vi "RDG822 User.vi"() -> ()   [LabVIEW 2013]
panel:
  in  "MenuCount":u32=1
  in  "RemoveReq?":bool=TRUE
  in  "userID":string="0001"
  out "error out":errorcluster
  in  "E:\\Study\\НИР_Маг\\FP":path=path "E:/Study/НИР_Маг/FP"
  in  "error in":errorcluster
  in  "DC":bool
  in  "FallEdgeDBL":dbl=10.0 format="%.3f"
  in  "RisEdgeDBL":dbl=10.0 format="%.3f"
  out "FallEdgeStr":string="10.0 ns"
  out "RisEdgeStr":string="10.0 ns"
  in  "Duty/Width":bool
  in  "Width":dbl=500.0 format="%.4f"
  in  "SymmDBL":dbl=50.0 format="%.1f"
  out "SymmStr":string="50.0 %"
  in  "Duty":dbl=50.0 format="%.3f"
  out "Duty-Width":string="50.000 %"
  in  "Noise":bool
  in  "Pulse":bool
  in  "Ramp":bool
  in  "Square":bool
  in  "Sine":bool
  in  "Slider":bool
  in  "PhaseDBL":dbl format="%.3f"
  in  "OK":bool
  out "PhaseStr":string="0.000 °"
  in  "LowL":dbl=-2.5 format="%.4f"
  in  "Offset":dbl format="%.4f"
  out "Offset-LowL":string="0.0000 Vdc"
  in  "Offset/LowL":bool
  in  "HighL":dbl=1.0 format="%.4f"
  in  "Ampl":dbl=5.0 format="%.4f"
  out "Ampl-HighL":string="5.0000 Vpp"
  in  "Ampl/HighL":bool
  in  "Freq":dbl=1000.0 format="%.6f"
  in  "Period":dbl=1.0 format="%.7f"
  out "Freq-Period":string="1000.000000000 kHz"
  in  "Freq/Period":bool
  in  "Left":bool
  in  "Right":bool
  in  "Out2":bool
  in  "Out1":bool
  out "Screen":picture
  in  "Menu":bool
  in  "Home":bool
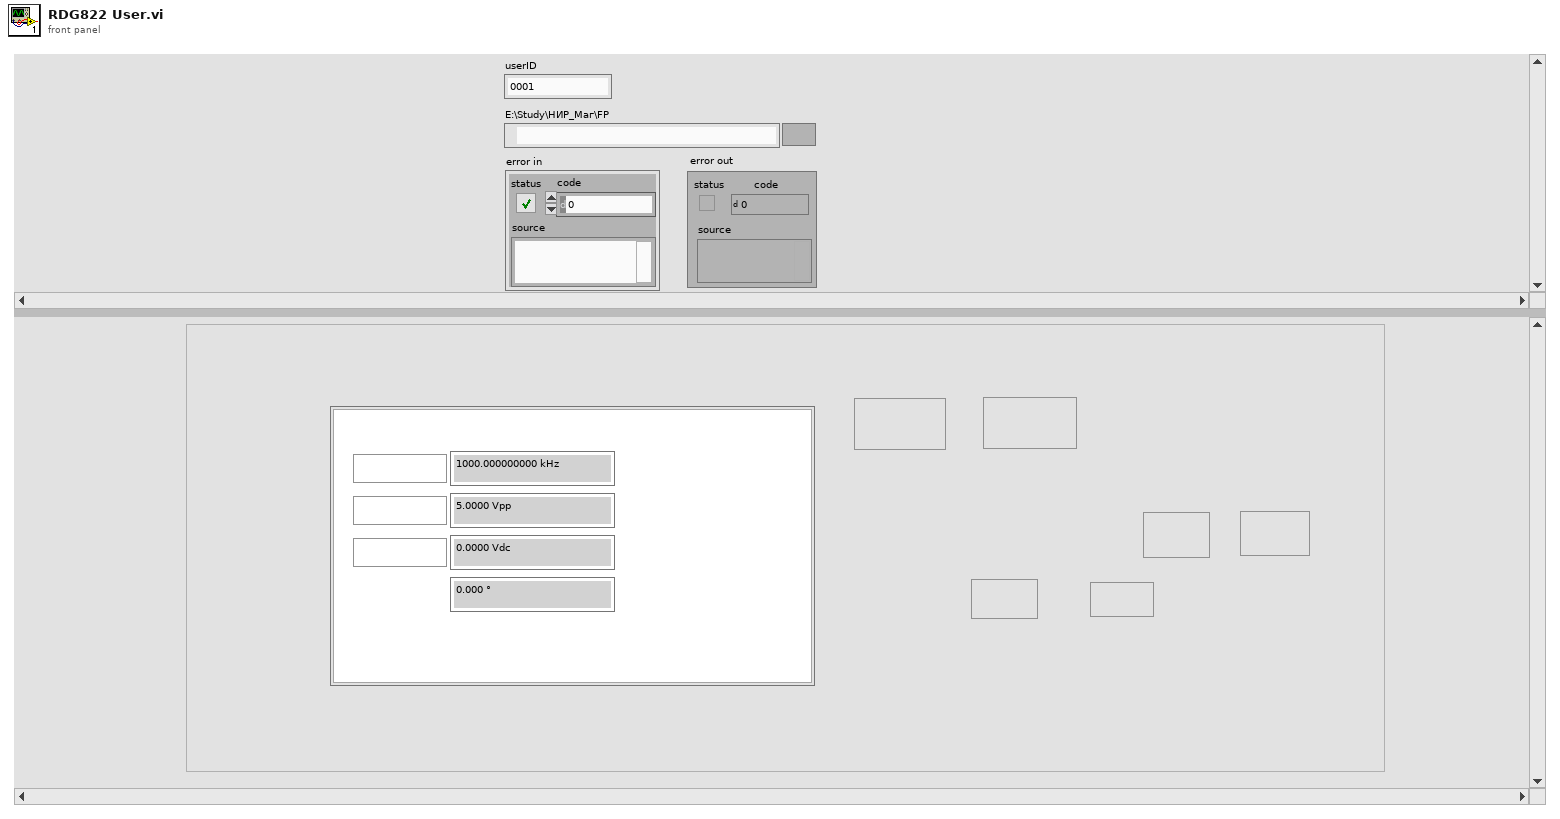
[diagram p1: front panel]
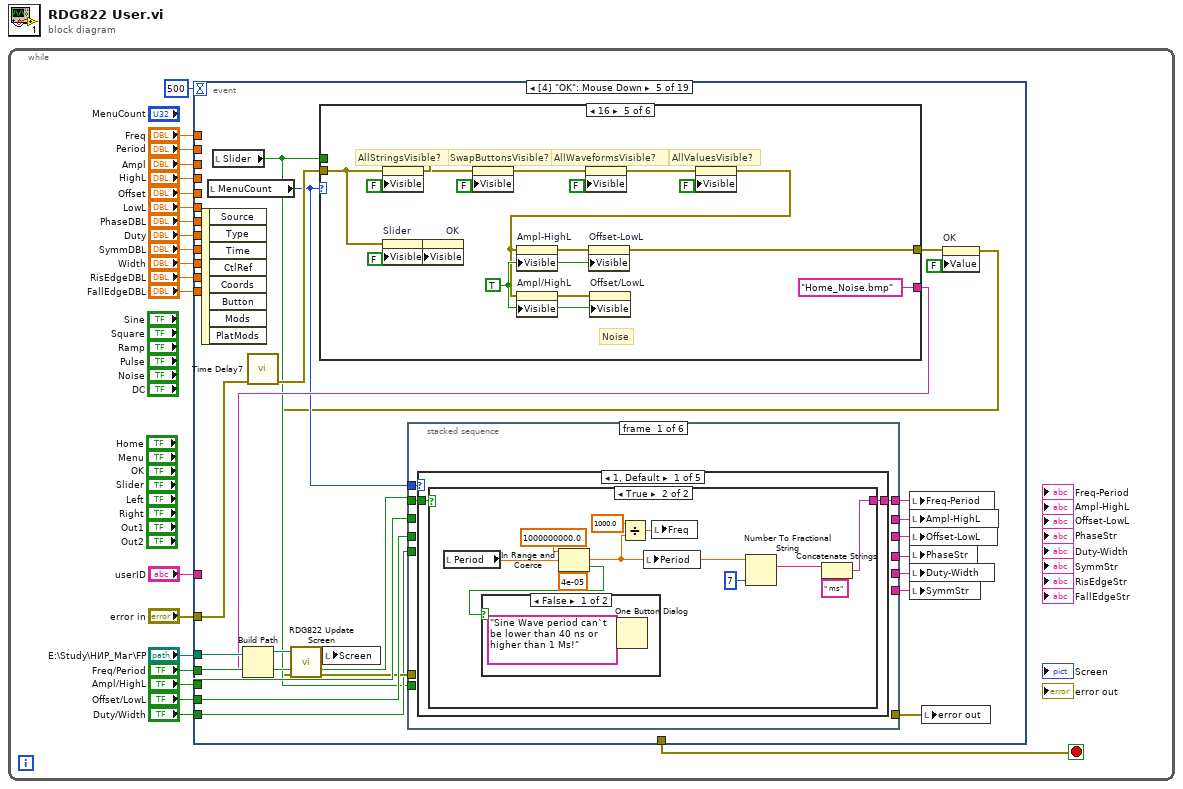
[diagram p0: block diagram]
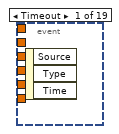
[diagram p2: hidden frame]
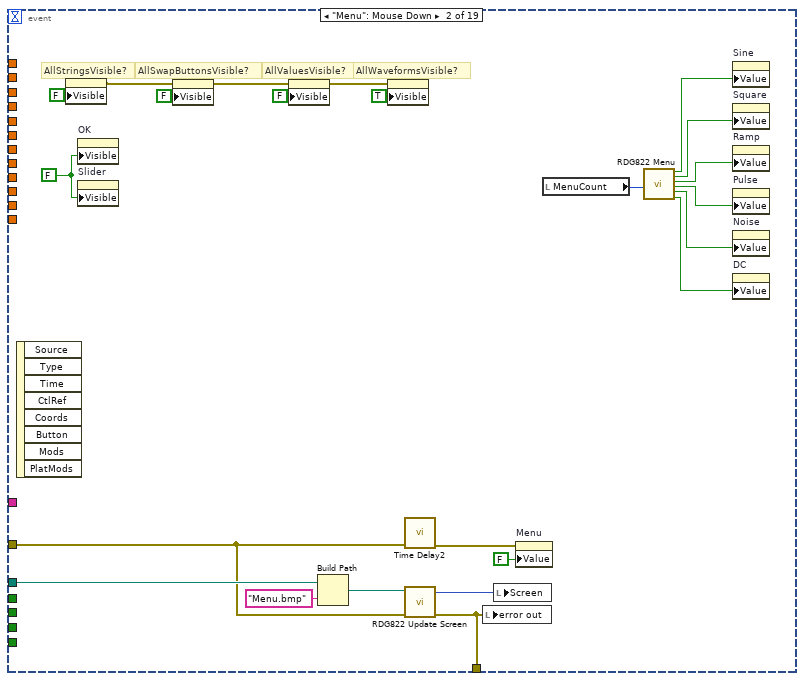
[diagram p3: hidden frame]
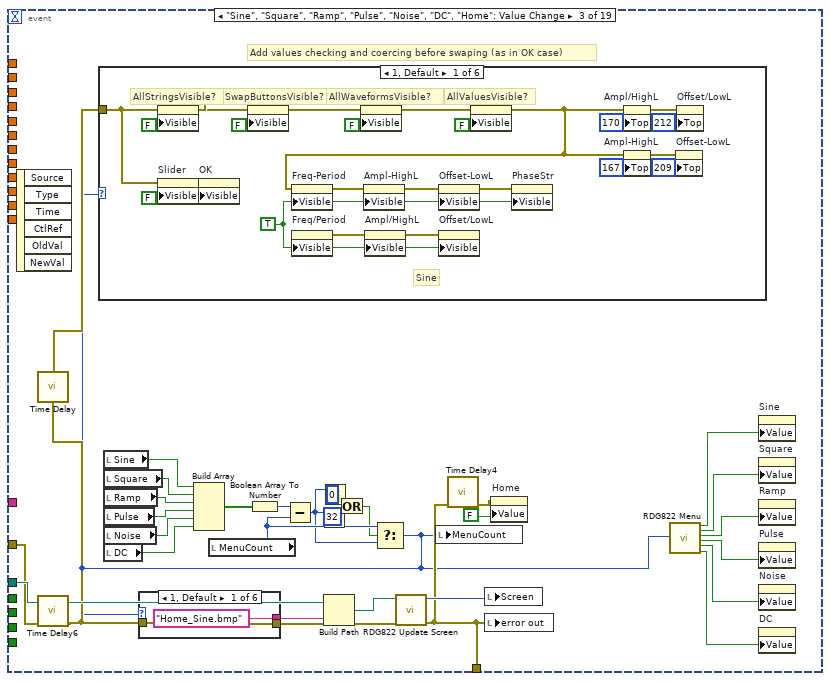
[diagram p4: hidden frame]
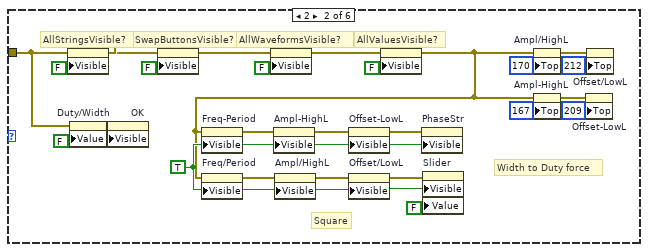
[diagram p5: hidden frame]
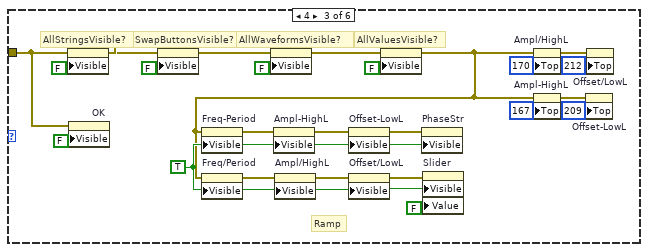
[diagram p6: hidden frame]
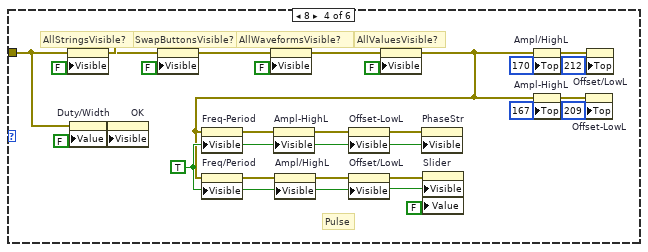
[diagram p7: hidden frame]
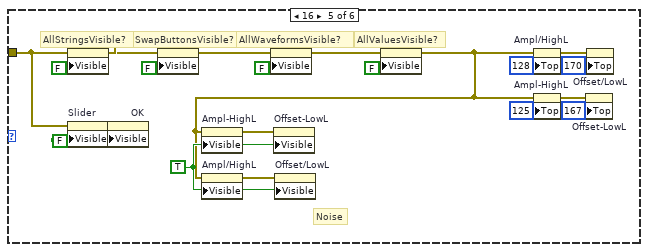
[diagram p8: hidden frame]
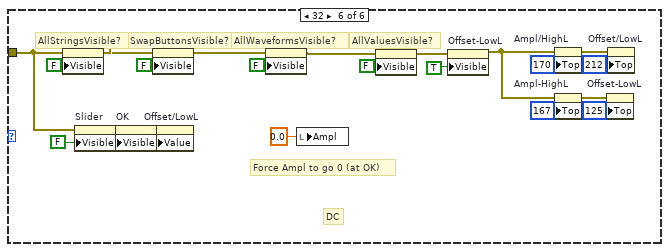
[diagram p9: hidden frame]
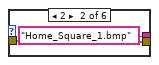
[diagram p10: hidden frame]
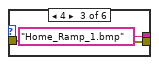
[diagram p11: hidden frame]
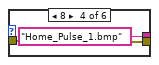
[diagram p12: hidden frame]
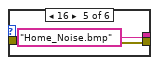
[diagram p13: hidden frame]
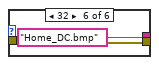
[diagram p14: hidden frame]
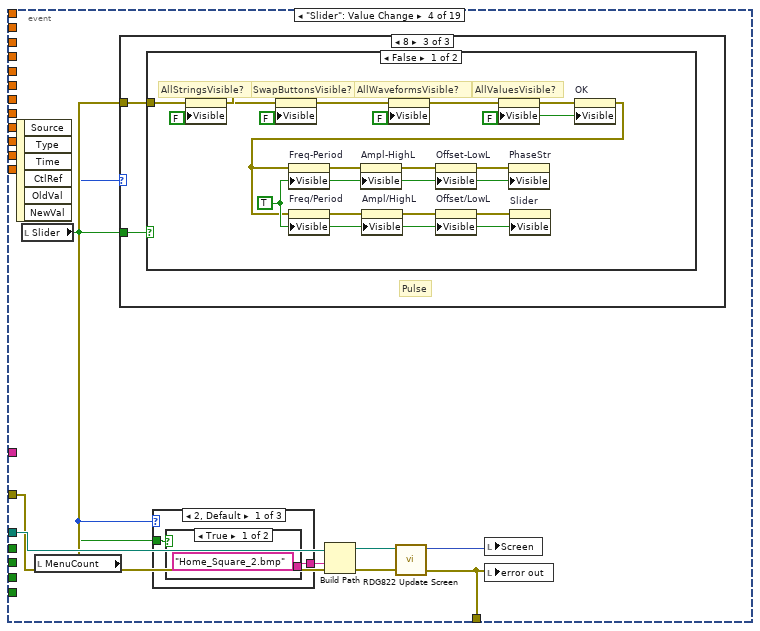
[diagram p15: hidden frame]
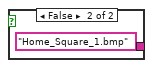
[diagram p16: hidden frame]
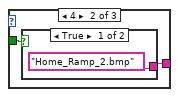
[diagram p17: hidden frame]
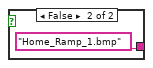
[diagram p18: hidden frame]
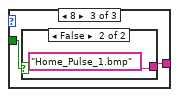
[diagram p19: hidden frame]
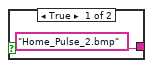
[diagram p20: hidden frame]
diagram:
  n1 = while {
    stop <- w21 stop-if-true
    n2 = event shown="[4] \"OK\": Mouse Down" {
      selector: _ -> [_ _ _ _ _ _ _ _ _ _ _ _ _ _ _ _ _ _ _]
      dyn-events: _ -> [_ _ _ _ _ _ _ _ _ _ _ _ _ _ _ _ _ _ _]
      timeout: 500 -> [_ _ _ _ _ _ _ _ _ _ _ _ _ _ _ _ _ _ _]
      tunnel: [_ w65 w89 w409 _ w1410 w1457 w1504 w1551 w1591 w1635 w1670 w1704 _ _ _ _ w1825 _] -> w21
      tunnel: "error in" -> [_ w63 w85 w408 w684 _ _ _ _ _ _ _ _ _ _ _ _ w1892 _]
      tunnel: "E:\\Study\\НИР_Маг\\FP" -> [_ w66 w93 w410 w693 w1415 w1462 w1509 w1556 w1587 w1639 w1675 w1709 _ _ _ _ w1880 _]
      tunnel: "Freq/Period" -> [_ _ _ _ w696 w1414 _ _ _ _ _ _ _ _ _ _ _ w1902 _]
      tunnel: "Ampl/HighL" -> [_ _ _ _ w695 _ w1461 _ _ _ _ _ _ _ _ _ _ w1903 _]
      tunnel: "Freq" -> [_ _ _ _ _ _ _ _ _ _ _ _ _ _ _ _ _ w1901 _]
      tunnel: "Ampl" -> [_ _ _ _ _ _ _ _ _ _ _ _ _ _ _ _ _ w1900 _]
      tunnel: "Period" -> [_ _ _ _ _ _ _ _ _ _ _ _ _ _ _ _ _ w1862 _]
      tunnel: "HighL" -> [_ _ _ _ _ _ _ _ _ _ _ _ _ _ _ _ _ w1897 _]
      tunnel: "Offset/LowL" -> [_ _ _ _ w694 _ _ w1508 _ _ _ _ _ _ _ _ _ w1899 _]
      tunnel: "Offset" -> [_ _ _ _ _ _ _ _ _ _ _ _ _ _ _ _ _ w1873 _]
      tunnel: "LowL" -> [_ _ _ _ _ _ _ _ _ _ _ _ _ _ _ _ _ w1898 _]
      tunnel: "PhaseDBL" -> [_ _ _ _ _ _ _ _ _ _ _ _ _ _ _ _ _ w1860 _]
      tunnel: "userID" -> [_ _ _ _ _ _ _ _ _ _ _ _ _ _ _ _ _ w1891 _]
      tunnel: "Duty" -> [_ _ _ _ _ _ _ _ _ _ _ _ _ _ _ _ _ w1865 _]
      tunnel: "SymmDBL" -> [_ _ _ _ _ _ _ _ _ _ _ _ _ _ _ _ _ w1868 _]
      tunnel: "Width" -> [_ _ _ _ _ _ _ _ _ _ _ _ _ _ _ _ _ w1863 _]
      tunnel: "Duty/Width" -> [_ _ _ _ w678 _ _ _ _ w1586 _ _ _ _ _ _ _ w1866 _]
      tunnel: "RisEdgeDBL" -> [_ _ _ _ _ _ _ _ _ _ _ _ _ _ _ _ _ _ _]
      tunnel: "FallEdgeDBL" -> [_ _ _ _ _ _ _ _ _ _ _ _ _ _ _ _ _ _ _]
      event Timeout {
        n3 = event-data() -> ()  [unwired: 1 in, 3 out]
      }
      event "Menu": Mouse Down {
        w34 = TRUE ("Visible")
        w47 = FALSE ("Visible")
        w54 = FALSE ("Visible")
        w57 = FALSE ("Visible")
        w61 = FALSE ("Visible")
        # "AllWaveformsVisible?"
        # "AllValuesVisible?"
        # "AllStringsVisible?"
        # "AllSwapButtonsVisible?"
        n4 = event-data() -> ()  [unwired: 1 in, 8 out]
        n5 = property on="Freq-Period" class="Str"("Visible"=w54) -> (error out=w52:errorcluster)  [unwired: 2 in, 1 out]
        n6 = property on="Ampl-HighL" class="Str"(error in=w52, "Visible"=w54) -> (error out=w51:errorcluster)  [unwired: 1 in, 1 out]
        n7 = property on="Offset-LowL" class="Str"(error in=w51, "Visible"=w54) -> (error out=w50:errorcluster)  [unwired: 1 in, 1 out]
        n8 = property on="PhaseStr" class="Str"(error in=w50, "Visible"=w54) -> (error out=w53:errorcluster)  [unwired: 1 in, 1 out]
        n9 = property on="Duty-Width" class="Str"(error in=w53, "Visible"=w54) -> (error out=w56:errorcluster)  [unwired: 1 in, 1 out]
        n10 = property on="SymmStr" class="Str"(error in=w56, "Visible"=w54) -> (error out=w55:errorcluster)  [unwired: 1 in, 1 out]
        n11 = property on="RisEdgeStr" class="Str"(error in=w55, "Visible"=w54) -> (error out=w49:errorcluster)  [unwired: 1 in, 1 out]
        n12 = property on="FallEdgeStr" class="Str"(error in=w49, "Visible"=w54) -> (error out=w48:errorcluster)  [unwired: 1 in, 1 out]
        n13 = property on="OK" class="Bool (strict)"("Visible"=w61) -> ()  [unwired: 2 in, 2 out]
        n14 = property on="Slider" class="Bool (strict)"("Visible"=w61) -> ()  [unwired: 2 in, 2 out]
        n15 = property on="Freq/Period" class="Bool (strict)"(error in=w48, "Visible"=w57) -> (error out=w60:errorcluster)  [unwired: 1 in, 1 out]
        n16 = property on="Ampl/HighL" class="Bool (strict)"(error in=w60, "Visible"=w57) -> (error out=w59:errorcluster)  [unwired: 1 in, 1 out]
        n17 = property on="Offset/LowL" class="Bool (strict)"(error in=w59, "Visible"=w57) -> (error out=w58:errorcluster)  [unwired: 1 in, 1 out]
        n18 = property on="Duty/Width" class="Bool (strict)"(error in=w58, "Visible"=w57) -> (error out=w35:errorcluster)  [unwired: 1 in, 1 out]
        n19 = property on="Freq" class="DigNum (strict)"(error in=w35, "Visible"=w47) -> (error out=w43:errorcluster)  [unwired: 1 in, 1 out]
        n20 = property on="Period" class="DigNum (strict)"(error in=w43, "Visible"=w47) -> (error out=w42:errorcluster)  [unwired: 1 in, 1 out]
        n21 = property on="Ampl" class="DigNum (strict)"(error in=w42, "Visible"=w47) -> (error out=w41:errorcluster)  [unwired: 1 in, 1 out]
        n22 = property on="HighL" class="DigNum (strict)"(error in=w41, "Visible"=w47) -> (error out=w44:errorcluster)  [unwired: 1 in, 1 out]
        n23 = property on="Offset" class="DigNum (strict)"(error in=w44, "Visible"=w47) -> (error out=w40:errorcluster)  [unwired: 1 in, 1 out]
        n24 = property on="LowL" class="DigNum (strict)"(error in=w40, "Visible"=w47) -> (error out=w39:errorcluster)  [unwired: 1 in, 1 out]
        n25 = property on="PhaseDBL" class="DigNum (strict)"(error in=w39, "Visible"=w47) -> (error out=w45:errorcluster)  [unwired: 1 in, 1 out]
        n26 = property on="Duty" class="DigNum (strict)"(error in=w45, "Visible"=w47) -> (error out=w46:errorcluster)  [unwired: 1 in, 1 out]
        n27 = property on="SymmDBL" class="DigNum (strict)"(error in=w46, "Visible"=w47) -> (error out=w38:errorcluster)  [unwired: 1 in, 1 out]
        n28 = property on="Width" class="DigNum (strict)"(error in=w38, "Visible"=w47) -> (error out=w37:errorcluster)  [unwired: 1 in, 1 out]
        n29 = property on="RisEdgeDBL" class="DigNum (strict)"(error in=w37, "Visible"=w47) -> (error out=w36:errorcluster)  [unwired: 1 in, 1 out]
        n30 = property on="FallEdgeDBL" class="DigNum (strict)"(error in=w36, "Visible"=w47) -> (error out=w28:errorcluster)  [unwired: 1 in, 1 out]
        n31 = Build Path(base path=w66, name or relative path="Menu.bmp") -> (appended path=w67:path)
        n32 = property on="Sine" class="Bool (strict)"(error in=w28, "Visible"=w34) -> (error out=w31:errorcluster)  [unwired: 1 in, 1 out]
        n33 = property on="Square" class="Bool (strict)"(error in=w31, "Visible"=w34) -> (error out=w30:errorcluster)  [unwired: 1 in, 1 out]
        n34 = property on="Ramp" class="Bool (strict)"(error in=w30, "Visible"=w34) -> (error out=w29:errorcluster)  [unwired: 1 in, 1 out]
        n35 = property on="Pulse" class="Bool (strict)"(error in=w29, "Visible"=w34) -> (error out=w32:errorcluster)  [unwired: 1 in, 1 out]
        n36 = property on="Noise" class="Bool (strict)"(error in=w32, "Visible"=w34) -> (error out=w33:errorcluster)  [unwired: 1 in, 1 out]
        n37 = property on="DC" class="Bool (strict)"(error in=w33, "Visible"=w34) -> ()  [unwired: 1 in, 2 out]
        n38 = call "Time Delay2"("error in (no error)"=w63) -> ("error out"=w70:errorcluster)  [unwired: 10 in]
        n39 = call "RDG822 Update Screen.vi"("error in"=w63, "Path to file"=w67) -> ("error out"=w65:errorcluster, "Screen"=w64:picture)  [unwired: 8 in]
        n40 = local write "error out"(w65) -> ()
        n41 = local write "Screen"(w64) -> ()
        n42 = property on="Menu" class="Bool (strict)"(error in=w70, "Value"=FALSE ("Visible")) -> ()  [unwired: 1 in, 2 out]
        n43 = local read "MenuCount"() -> (w62:u32)
        n44 = call "RDG822 Menu.vi"("MenuID"=w62) -> ("Sine"=w27:bool, "Square"=w26:bool, "Ramp"=w25:bool, "Pulse"=w24:bool, "Noise"=w23:bool, "DC"=w22:bool)  [unwired: 13 in]
        n45 = property on="Sine" class="Bool (strict)"("Value"=w27) -> ()  [unwired: 2 in, 2 out]
        n46 = property on="Square" class="Bool (strict)"("Value"=w26) -> ()  [unwired: 2 in, 2 out]
        n47 = property on="Ramp" class="Bool (strict)"("Value"=w25) -> ()  [unwired: 2 in, 2 out]
        n48 = property on="Pulse" class="Bool (strict)"("Value"=w24) -> ()  [unwired: 2 in, 2 out]
        n49 = property on="Noise" class="Bool (strict)"("Value"=w23) -> ()  [unwired: 2 in, 2 out]
        n50 = property on="DC" class="Bool (strict)"("Value"=w22) -> ()  [unwired: 2 in, 2 out]
      }
      event "Sine", "Square", "Ramp", "Pulse", "Noise", "DC", "Home": Value Change {
        # "Add values checking and coercing before swaping (as in OK case)"
        n51 = event-data() -> ()  [unwired: 1 in, 6 out]
        n52 = call "Time Delay6"("error in (no error)"=w85) -> ("error out"=w82:errorcluster)  [unwired: 10 in]
        n53 = call "Time Delay"("error in (no error)"=w82) -> ("error out"=w83:errorcluster)  [unwired: 10 in]
        n54 = local read "Sine"() -> (w98:bool)
        n55 = local read "Square"() -> (w99:bool)
        n56 = local read "Ramp"() -> (w100:bool)
        n57 = local read "Pulse"() -> (w97:bool)
        n58 = local read "Noise"() -> (w96:bool)
        n59 = local read "DC"() -> (w78:bool)
        n60 = Build Array(w98, w99, w100, w97, w96, w78) -> (w101:bool[])
        n61 = local read "MenuCount"() -> (w81:u32)
        n62 = Boolean Array To Number(Boolean array=w101) -> (number=w95:u32)
        n63 = Subtract(x=w95, y=w81) -> (x-y=w80:u32)
        n64 = Greater?(x=w80, y=u32 32) -> (0:w87:bool)
        n65 = Less Or Equal?(x=w80, y=u32 0) -> (x <= y?=w88:bool)
        n66 = Or(x=w88, y=w87) -> (x .or. y?=w79:bool)
        n67 = Select(t=w81, s=w79, f=w80) -> (s? t:f=w71:u32)
        n68 = case shown="1, Default" w71 {
          tunnel: w83 -> [w105 w157 w203 w257 w305 w350]
          frame 1, Default {
            w108 = FALSE ("Visible")
            w117 = FALSE ("Visible")
            w132 = FALSE ("Visible")
            w138 = FALSE ("Visible")
            w139 = FALSE ("Visible")
            w140 = TRUE ("Visible")
            # "Sine"
            # "AllSwapButtonsVisible?"
            # "AllStringsVisible?"
            # "AllValuesVisible?"
            # "AllWaveformsVisible?"
            n69 = property on="Freq-Period" class="Str"(error in=w105, "Visible"=w117) -> (error out=w115:errorcluster)  [unwired: 1 in, 1 out]
            n70 = property on="Ampl-HighL" class="Str"(error in=w115, "Visible"=w117) -> (error out=w114:errorcluster)  [unwired: 1 in, 1 out]
            n71 = property on="Offset-LowL" class="Str"(error in=w114, "Visible"=w117) -> (error out=w113:errorcluster)  [unwired: 1 in, 1 out]
            n72 = property on="PhaseStr" class="Str"(error in=w113, "Visible"=w117) -> (error out=w116:errorcluster)  [unwired: 1 in, 1 out]
            n73 = property on="Duty-Width" class="Str"(error in=w116, "Visible"=w117) -> (error out=w119:errorcluster)  [unwired: 1 in, 1 out]
            n74 = property on="SymmStr" class="Str"(error in=w119, "Visible"=w117) -> (error out=w118:errorcluster)  [unwired: 1 in, 1 out]
            n75 = property on="RisEdgeStr" class="Str"(error in=w118, "Visible"=w117) -> (error out=w112:errorcluster)  [unwired: 1 in, 1 out]
            n76 = property on="FallEdgeStr" class="Str"(error in=w112, "Visible"=w117) -> (error out=w107:errorcluster)  [unwired: 1 in, 1 out]
            n77 = property on="Slider" class="Bool (strict)"(error in=w105, "Visible"=w139) -> ()  [unwired: 1 in, 2 out]
            n78 = property on="OK" class="Bool (strict)"("Visible"=w139) -> ()  [unwired: 2 in, 2 out]
            n79 = property on="Freq/Period" class="Bool (strict)"(error in=w107, "Visible"=w108) -> (error out=w111:errorcluster)  [unwired: 1 in, 1 out]
            n80 = property on="Ampl/HighL" class="Bool (strict)"(error in=w111, "Visible"=w108) -> (error out=w110:errorcluster)  [unwired: 1 in, 1 out]
            n81 = property on="Offset/LowL" class="Bool (strict)"(error in=w110, "Visible"=w108) -> (error out=w109:errorcluster)  [unwired: 1 in, 1 out]
            n82 = property on="Duty/Width" class="Bool (strict)"(error in=w109, "Visible"=w108) -> (error out=w106:errorcluster)  [unwired: 1 in, 1 out]
            n83 = property on="Freq/Period" class="Bool (strict)"("Visible"=w140) -> (error out=w148:errorcluster)  [unwired: 2 in, 1 out]
            n84 = property on="Sine" class="Bool (strict)"(error in=w106, "Visible"=w138) -> (error out=w135:errorcluster)  [unwired: 1 in, 1 out]
            n85 = property on="Square" class="Bool (strict)"(error in=w135, "Visible"=w138) -> (error out=w134:errorcluster)  [unwired: 1 in, 1 out]
            n86 = property on="Ramp" class="Bool (strict)"(error in=w134, "Visible"=w138) -> (error out=w133:errorcluster)  [unwired: 1 in, 1 out]
            n87 = property on="Pulse" class="Bool (strict)"(error in=w133, "Visible"=w138) -> (error out=w136:errorcluster)  [unwired: 1 in, 1 out]
            n88 = property on="Noise" class="Bool (strict)"(error in=w136, "Visible"=w138) -> (error out=w137:errorcluster)  [unwired: 1 in, 1 out]
            n89 = property on="DC" class="Bool (strict)"(error in=w137, "Visible"=w138) -> (error out=w120:errorcluster)  [unwired: 1 in, 1 out]
            n90 = property on="Ampl/HighL" class="Bool (strict)"(error in=w148, "Visible"=w140) -> (error out=w147:errorcluster)  [unwired: 1 in, 1 out]
            n91 = property on="Offset/LowL" class="Bool (strict)"(error in=w147, "Visible"=w140) -> ()  [unwired: 1 in, 2 out]
            n92 = property on="Freq" class="DigNum (strict)"(error in=w120, "Visible"=w132) -> (error out=w128:errorcluster)  [unwired: 1 in, 1 out]
            n93 = property on="Period" class="DigNum (strict)"(error in=w128, "Visible"=w132) -> (error out=w127:errorcluster)  [unwired: 1 in, 1 out]
            n94 = property on="Ampl" class="DigNum (strict)"(error in=w127, "Visible"=w132) -> (error out=w126:errorcluster)  [unwired: 1 in, 1 out]
            n95 = property on="HighL" class="DigNum (strict)"(error in=w126, "Visible"=w132) -> (error out=w129:errorcluster)  [unwired: 1 in, 1 out]
            n96 = property on="Offset" class="DigNum (strict)"(error in=w129, "Visible"=w132) -> (error out=w125:errorcluster)  [unwired: 1 in, 1 out]
            n97 = property on="LowL" class="DigNum (strict)"(error in=w125, "Visible"=w132) -> (error out=w124:errorcluster)  [unwired: 1 in, 1 out]
            n98 = property on="PhaseDBL" class="DigNum (strict)"(error in=w124, "Visible"=w132) -> (error out=w130:errorcluster)  [unwired: 1 in, 1 out]
            n99 = property on="Duty" class="DigNum (strict)"(error in=w130, "Visible"=w132) -> (error out=w131:errorcluster)  [unwired: 1 in, 1 out]
            n100 = property on="SymmDBL" class="DigNum (strict)"(error in=w131, "Visible"=w132) -> (error out=w123:errorcluster)  [unwired: 1 in, 1 out]
            n101 = property on="Width" class="DigNum (strict)"(error in=w123, "Visible"=w132) -> (error out=w122:errorcluster)  [unwired: 1 in, 1 out]
            n102 = property on="RisEdgeDBL" class="DigNum (strict)"(error in=w122, "Visible"=w132) -> (error out=w121:errorcluster)  [unwired: 1 in, 1 out]
            n103 = property on="FallEdgeDBL" class="DigNum (strict)"(error in=w121, "Visible"=w132) -> (error out=w104:errorcluster)  [unwired: 1 in, 1 out]
            n104 = property on="Freq-Period" class="Str"(error in=w104, "Visible"=w140) -> (error out=w151:errorcluster)  [unwired: 1 in, 1 out]
            n105 = property on="Ampl-HighL" class="Str"(error in=w151, "Visible"=w140) -> (error out=w150:errorcluster)  [unwired: 1 in, 1 out]
            n106 = property on="Offset-LowL" class="Str"(error in=w150, "Visible"=w140) -> (error out=w149:errorcluster)  [unwired: 1 in, 1 out]
            n107 = property on="PhaseStr" class="Str"(error in=w149, "Visible"=w140) -> ()  [unwired: 1 in, 2 out]
            n108 = property on="Ampl/HighL" class="Bool (strict)"(error in=w104, "Top"=170 ("Position:Top")) -> (error out=w144:errorcluster)  [unwired: 1 in, 1 out]
            n109 = property on="Ampl-HighL" class="Str"(error in=w104, "Top"=167 ("Position:Top")) -> (error out=w141:errorcluster)  [unwired: 1 in, 1 out]
            n110 = property on="Offset-LowL" class="Str"(error in=w141, "Top"=209 ("Position:Top")) -> ()  [unwired: 1 in, 2 out]
            n111 = property on="Offset/LowL" class="Bool (strict)"(error in=w144, "Top"=212 ("Position:Top")) -> ()  [unwired: 1 in, 2 out]
          }
          frame 2 {
            w160 = FALSE ("Visible")
            w169 = FALSE ("Visible")
            w184 = FALSE ("Visible")
            w190 = FALSE ("Visible")
            w156 = FALSE ("Visible")
            w154 = TRUE ("Visible")
            # "Square"
            # "Width to Duty force"
            # "AllSwapButtonsVisible?"
            # "AllStringsVisible?"
            # "AllValuesVisible?"
            # "AllWaveformsVisible?"
            n112 = property on="Freq-Period" class="Str"(error in=w157, "Visible"=w169) -> (error out=w167:errorcluster)  [unwired: 1 in, 1 out]
            n113 = property on="Ampl-HighL" class="Str"(error in=w167, "Visible"=w169) -> (error out=w166:errorcluster)  [unwired: 1 in, 1 out]
            n114 = property on="Offset-LowL" class="Str"(error in=w166, "Visible"=w169) -> (error out=w165:errorcluster)  [unwired: 1 in, 1 out]
            n115 = property on="PhaseStr" class="Str"(error in=w165, "Visible"=w169) -> (error out=w168:errorcluster)  [unwired: 1 in, 1 out]
            n116 = property on="Duty-Width" class="Str"(error in=w168, "Visible"=w169) -> (error out=w171:errorcluster)  [unwired: 1 in, 1 out]
            n117 = property on="SymmStr" class="Str"(error in=w171, "Visible"=w169) -> (error out=w170:errorcluster)  [unwired: 1 in, 1 out]
            n118 = property on="RisEdgeStr" class="Str"(error in=w170, "Visible"=w169) -> (error out=w164:errorcluster)  [unwired: 1 in, 1 out]
            n119 = property on="FallEdgeStr" class="Str"(error in=w164, "Visible"=w169) -> (error out=w159:errorcluster)  [unwired: 1 in, 1 out]
            n120 = property on="Duty/Width" class="Bool (strict)"(error in=w157, "Value"=w156) -> ()  [unwired: 1 in, 2 out]
            n121 = property on="OK" class="Bool (strict)"("Visible"=w156) -> ()  [unwired: 2 in, 2 out]
            n122 = property on="Freq/Period" class="Bool (strict)"(error in=w159, "Visible"=w160) -> (error out=w163:errorcluster)  [unwired: 1 in, 1 out]
            n123 = property on="Ampl/HighL" class="Bool (strict)"(error in=w163, "Visible"=w160) -> (error out=w162:errorcluster)  [unwired: 1 in, 1 out]
            n124 = property on="Offset/LowL" class="Bool (strict)"(error in=w162, "Visible"=w160) -> (error out=w161:errorcluster)  [unwired: 1 in, 1 out]
            n125 = property on="Duty/Width" class="Bool (strict)"(error in=w161, "Visible"=w160) -> (error out=w158:errorcluster)  [unwired: 1 in, 1 out]
            n126 = property on="Sine" class="Bool (strict)"(error in=w158, "Visible"=w190) -> (error out=w187:errorcluster)  [unwired: 1 in, 1 out]
            n127 = property on="Square" class="Bool (strict)"(error in=w187, "Visible"=w190) -> (error out=w186:errorcluster)  [unwired: 1 in, 1 out]
            n128 = property on="Ramp" class="Bool (strict)"(error in=w186, "Visible"=w190) -> (error out=w185:errorcluster)  [unwired: 1 in, 1 out]
            n129 = property on="Pulse" class="Bool (strict)"(error in=w185, "Visible"=w190) -> (error out=w188:errorcluster)  [unwired: 1 in, 1 out]
            n130 = property on="Noise" class="Bool (strict)"(error in=w188, "Visible"=w190) -> (error out=w189:errorcluster)  [unwired: 1 in, 1 out]
            n131 = property on="DC" class="Bool (strict)"(error in=w189, "Visible"=w190) -> (error out=w172:errorcluster)  [unwired: 1 in, 1 out]
            n132 = property on="Freq" class="DigNum (strict)"(error in=w172, "Visible"=w184) -> (error out=w180:errorcluster)  [unwired: 1 in, 1 out]
            n133 = property on="Period" class="DigNum (strict)"(error in=w180, "Visible"=w184) -> (error out=w179:errorcluster)  [unwired: 1 in, 1 out]
            n134 = property on="Ampl" class="DigNum (strict)"(error in=w179, "Visible"=w184) -> (error out=w178:errorcluster)  [unwired: 1 in, 1 out]
            n135 = property on="HighL" class="DigNum (strict)"(error in=w178, "Visible"=w184) -> (error out=w181:errorcluster)  [unwired: 1 in, 1 out]
            n136 = property on="Offset" class="DigNum (strict)"(error in=w181, "Visible"=w184) -> (error out=w177:errorcluster)  [unwired: 1 in, 1 out]
            n137 = property on="LowL" class="DigNum (strict)"(error in=w177, "Visible"=w184) -> (error out=w176:errorcluster)  [unwired: 1 in, 1 out]
            n138 = property on="PhaseDBL" class="DigNum (strict)"(error in=w176, "Visible"=w184) -> (error out=w182:errorcluster)  [unwired: 1 in, 1 out]
            n139 = property on="Duty" class="DigNum (strict)"(error in=w182, "Visible"=w184) -> (error out=w183:errorcluster)  [unwired: 1 in, 1 out]
            n140 = property on="SymmDBL" class="DigNum (strict)"(error in=w183, "Visible"=w184) -> (error out=w175:errorcluster)  [unwired: 1 in, 1 out]
            n141 = property on="Width" class="DigNum (strict)"(error in=w175, "Visible"=w184) -> (error out=w174:errorcluster)  [unwired: 1 in, 1 out]
            n142 = property on="RisEdgeDBL" class="DigNum (strict)"(error in=w174, "Visible"=w184) -> (error out=w173:errorcluster)  [unwired: 1 in, 1 out]
            n143 = property on="FallEdgeDBL" class="DigNum (strict)"(error in=w173, "Visible"=w184) -> (error out=w152:errorcluster)  [unwired: 1 in, 1 out]
            n144 = property on="Freq-Period" class="Str"(error in=w152, "Visible"=w154) -> (error out=w201:errorcluster)  [unwired: 1 in, 1 out]
            n145 = property on="Freq/Period" class="Bool (strict)"(error in=w152, "Visible"=w154) -> (error out=w198:errorcluster)  [unwired: 1 in, 1 out]
            n146 = property on="Ampl-HighL" class="Str"(error in=w201, "Visible"=w154) -> (error out=w200:errorcluster)  [unwired: 1 in, 1 out]
            n147 = property on="Ampl/HighL" class="Bool (strict)"(error in=w198, "Visible"=w154) -> (error out=w197:errorcluster)  [unwired: 1 in, 1 out]
            n148 = property on="Offset-LowL" class="Str"(error in=w200, "Visible"=w154) -> (error out=w199:errorcluster)  [unwired: 1 in, 1 out]
            n149 = property on="Offset/LowL" class="Bool (strict)"(error in=w197, "Visible"=w154) -> (error out=w155:errorcluster)  [unwired: 1 in, 1 out]
            n150 = property on="PhaseStr" class="Str"(error in=w199, "Visible"=w154) -> ()  [unwired: 1 in, 2 out]
            n151 = property on="Slider" class="Bool (strict)"(error in=w155, "Visible"=w154, "Value"=FALSE ("Slider")) -> ()  [unwired: 1 in, 2 out]
            n152 = property on="Ampl/HighL" class="Bool (strict)"(error in=w152, "Top"=170 ("Position:Top")) -> (error out=w194:errorcluster)  [unwired: 1 in, 1 out]
            n153 = property on="Ampl-HighL" class="Str"(error in=w152, "Top"=167 ("Position:Top")) -> (error out=w191:errorcluster)  [unwired: 1 in, 1 out]
            n154 = property on="Offset-LowL" class="Str"(error in=w191, "Top"=209 ("Position:Top")) -> ()  [unwired: 1 in, 2 out]
            n155 = property on="Offset/LowL" class="Bool (strict)"(error in=w194, "Top"=212 ("Position:Top")) -> ()  [unwired: 1 in, 2 out]
          }
          frame 4 {
            w210 = FALSE ("Visible")
            w219 = FALSE ("Visible")
            w234 = FALSE ("Visible")
            w240 = FALSE ("Visible")
            w205 = TRUE ("Visible")
            # "Ramp"
            # "AllSwapButtonsVisible?"
            # "AllStringsVisible?"
            # "AllValuesVisible?"
            # "AllWaveformsVisible?"
            n156 = property on="Freq-Period" class="Str"(error in=w203, "Visible"=w219) -> (error out=w217:errorcluster)  [unwired: 1 in, 1 out]
            n157 = property on="Ampl-HighL" class="Str"(error in=w217, "Visible"=w219) -> (error out=w216:errorcluster)  [unwired: 1 in, 1 out]
            n158 = property on="Offset-LowL" class="Str"(error in=w216, "Visible"=w219) -> (error out=w215:errorcluster)  [unwired: 1 in, 1 out]
            n159 = property on="PhaseStr" class="Str"(error in=w215, "Visible"=w219) -> (error out=w218:errorcluster)  [unwired: 1 in, 1 out]
            n160 = property on="Duty-Width" class="Str"(error in=w218, "Visible"=w219) -> (error out=w221:errorcluster)  [unwired: 1 in, 1 out]
            n161 = property on="SymmStr" class="Str"(error in=w221, "Visible"=w219) -> (error out=w220:errorcluster)  [unwired: 1 in, 1 out]
            n162 = property on="RisEdgeStr" class="Str"(error in=w220, "Visible"=w219) -> (error out=w214:errorcluster)  [unwired: 1 in, 1 out]
            n163 = property on="FallEdgeStr" class="Str"(error in=w214, "Visible"=w219) -> (error out=w209:errorcluster)  [unwired: 1 in, 1 out]
            n164 = property on="OK" class="Bool (strict)"(error in=w203, "Visible"=FALSE) -> ()  [unwired: 1 in, 2 out]
            n165 = property on="Freq/Period" class="Bool (strict)"(error in=w209, "Visible"=w210) -> (error out=w213:errorcluster)  [unwired: 1 in, 1 out]
            n166 = property on="Ampl/HighL" class="Bool (strict)"(error in=w213, "Visible"=w210) -> (error out=w212:errorcluster)  [unwired: 1 in, 1 out]
            n167 = property on="Offset/LowL" class="Bool (strict)"(error in=w212, "Visible"=w210) -> (error out=w211:errorcluster)  [unwired: 1 in, 1 out]
            n168 = property on="Duty/Width" class="Bool (strict)"(error in=w211, "Visible"=w210) -> (error out=w208:errorcluster)  [unwired: 1 in, 1 out]
            n169 = property on="Sine" class="Bool (strict)"(error in=w208, "Visible"=w240) -> (error out=w237:errorcluster)  [unwired: 1 in, 1 out]
            n170 = property on="Square" class="Bool (strict)"(error in=w237, "Visible"=w240) -> (error out=w236:errorcluster)  [unwired: 1 in, 1 out]
            n171 = property on="Ramp" class="Bool (strict)"(error in=w236, "Visible"=w240) -> (error out=w235:errorcluster)  [unwired: 1 in, 1 out]
            n172 = property on="Pulse" class="Bool (strict)"(error in=w235, "Visible"=w240) -> (error out=w238:errorcluster)  [unwired: 1 in, 1 out]
            n173 = property on="Noise" class="Bool (strict)"(error in=w238, "Visible"=w240) -> (error out=w239:errorcluster)  [unwired: 1 in, 1 out]
            n174 = property on="DC" class="Bool (strict)"(error in=w239, "Visible"=w240) -> (error out=w222:errorcluster)  [unwired: 1 in, 1 out]
            n175 = property on="Freq" class="DigNum (strict)"(error in=w222, "Visible"=w234) -> (error out=w230:errorcluster)  [unwired: 1 in, 1 out]
            n176 = property on="Period" class="DigNum (strict)"(error in=w230, "Visible"=w234) -> (error out=w229:errorcluster)  [unwired: 1 in, 1 out]
            n177 = property on="Ampl" class="DigNum (strict)"(error in=w229, "Visible"=w234) -> (error out=w228:errorcluster)  [unwired: 1 in, 1 out]
            n178 = property on="HighL" class="DigNum (strict)"(error in=w228, "Visible"=w234) -> (error out=w231:errorcluster)  [unwired: 1 in, 1 out]
            n179 = property on="Offset" class="DigNum (strict)"(error in=w231, "Visible"=w234) -> (error out=w227:errorcluster)  [unwired: 1 in, 1 out]
            n180 = property on="LowL" class="DigNum (strict)"(error in=w227, "Visible"=w234) -> (error out=w226:errorcluster)  [unwired: 1 in, 1 out]
            n181 = property on="PhaseDBL" class="DigNum (strict)"(error in=w226, "Visible"=w234) -> (error out=w232:errorcluster)  [unwired: 1 in, 1 out]
            n182 = property on="Duty" class="DigNum (strict)"(error in=w232, "Visible"=w234) -> (error out=w233:errorcluster)  [unwired: 1 in, 1 out]
            n183 = property on="SymmDBL" class="DigNum (strict)"(error in=w233, "Visible"=w234) -> (error out=w225:errorcluster)  [unwired: 1 in, 1 out]
            n184 = property on="Width" class="DigNum (strict)"(error in=w225, "Visible"=w234) -> (error out=w224:errorcluster)  [unwired: 1 in, 1 out]
            n185 = property on="RisEdgeDBL" class="DigNum (strict)"(error in=w224, "Visible"=w234) -> (error out=w223:errorcluster)  [unwired: 1 in, 1 out]
            n186 = property on="FallEdgeDBL" class="DigNum (strict)"(error in=w223, "Visible"=w234) -> (error out=w202:errorcluster)  [unwired: 1 in, 1 out]
            n187 = property on="Freq-Period" class="Str"(error in=w202, "Visible"=w205) -> (error out=w251:errorcluster)  [unwired: 1 in, 1 out]
            n188 = property on="Freq/Period" class="Bool (strict)"(error in=w202, "Visible"=w205) -> (error out=w248:errorcluster)  [unwired: 1 in, 1 out]
            n189 = property on="Ampl-HighL" class="Str"(error in=w251, "Visible"=w205) -> (error out=w250:errorcluster)  [unwired: 1 in, 1 out]
            n190 = property on="Ampl/HighL" class="Bool (strict)"(error in=w248, "Visible"=w205) -> (error out=w247:errorcluster)  [unwired: 1 in, 1 out]
            n191 = property on="Offset-LowL" class="Str"(error in=w250, "Visible"=w205) -> (error out=w249:errorcluster)  [unwired: 1 in, 1 out]
            n192 = property on="Offset/LowL" class="Bool (strict)"(error in=w247, "Visible"=w205) -> (error out=w206:errorcluster)  [unwired: 1 in, 1 out]
            n193 = property on="PhaseStr" class="Str"(error in=w249, "Visible"=w205) -> ()  [unwired: 1 in, 2 out]
            n194 = property on="Slider" class="Bool (strict)"(error in=w206, "Visible"=w205, "Value"=FALSE ("Slider")) -> ()  [unwired: 1 in, 2 out]
            n195 = property on="Ampl/HighL" class="Bool (strict)"(error in=w202, "Top"=170 ("Position:Top")) -> (error out=w244:errorcluster)  [unwired: 1 in, 1 out]
            n196 = property on="Ampl-HighL" class="Str"(error in=w202, "Top"=167 ("Position:Top")) -> (error out=w241:errorcluster)  [unwired: 1 in, 1 out]
            n197 = property on="Offset-LowL" class="Str"(error in=w241, "Top"=209 ("Position:Top")) -> ()  [unwired: 1 in, 2 out]
            n198 = property on="Offset/LowL" class="Bool (strict)"(error in=w244, "Top"=212 ("Position:Top")) -> ()  [unwired: 1 in, 2 out]
          }
          frame 8 {
            w260 = FALSE ("Visible")
            w269 = FALSE ("Visible")
            w284 = FALSE ("Visible")
            w290 = FALSE ("Visible")
            w256 = FALSE ("Visible")
            w254 = TRUE ("Visible")
            # "Pulse"
            # "AllSwapButtonsVisible?"
            # "AllStringsVisible?"
            # "AllValuesVisible?"
            # "AllWaveformsVisible?"
            n199 = property on="Freq-Period" class="Str"(error in=w257, "Visible"=w269) -> (error out=w267:errorcluster)  [unwired: 1 in, 1 out]
            n200 = property on="Ampl-HighL" class="Str"(error in=w267, "Visible"=w269) -> (error out=w266:errorcluster)  [unwired: 1 in, 1 out]
            n201 = property on="Offset-LowL" class="Str"(error in=w266, "Visible"=w269) -> (error out=w265:errorcluster)  [unwired: 1 in, 1 out]
            n202 = property on="PhaseStr" class="Str"(error in=w265, "Visible"=w269) -> (error out=w268:errorcluster)  [unwired: 1 in, 1 out]
            n203 = property on="Duty-Width" class="Str"(error in=w268, "Visible"=w269) -> (error out=w271:errorcluster)  [unwired: 1 in, 1 out]
            n204 = property on="SymmStr" class="Str"(error in=w271, "Visible"=w269) -> (error out=w270:errorcluster)  [unwired: 1 in, 1 out]
            n205 = property on="RisEdgeStr" class="Str"(error in=w270, "Visible"=w269) -> (error out=w264:errorcluster)  [unwired: 1 in, 1 out]
            n206 = property on="FallEdgeStr" class="Str"(error in=w264, "Visible"=w269) -> (error out=w259:errorcluster)  [unwired: 1 in, 1 out]
            n207 = property on="Duty/Width" class="Bool (strict)"(error in=w257, "Value"=w256) -> ()  [unwired: 1 in, 2 out]
            n208 = property on="OK" class="Bool (strict)"("Visible"=w256) -> ()  [unwired: 2 in, 2 out]
            n209 = property on="Freq/Period" class="Bool (strict)"(error in=w259, "Visible"=w260) -> (error out=w263:errorcluster)  [unwired: 1 in, 1 out]
            n210 = property on="Ampl/HighL" class="Bool (strict)"(error in=w263, "Visible"=w260) -> (error out=w262:errorcluster)  [unwired: 1 in, 1 out]
            n211 = property on="Offset/LowL" class="Bool (strict)"(error in=w262, "Visible"=w260) -> (error out=w261:errorcluster)  [unwired: 1 in, 1 out]
            n212 = property on="Duty/Width" class="Bool (strict)"(error in=w261, "Visible"=w260) -> (error out=w258:errorcluster)  [unwired: 1 in, 1 out]
            n213 = property on="Sine" class="Bool (strict)"(error in=w258, "Visible"=w290) -> (error out=w287:errorcluster)  [unwired: 1 in, 1 out]
            n214 = property on="Square" class="Bool (strict)"(error in=w287, "Visible"=w290) -> (error out=w286:errorcluster)  [unwired: 1 in, 1 out]
            n215 = property on="Ramp" class="Bool (strict)"(error in=w286, "Visible"=w290) -> (error out=w285:errorcluster)  [unwired: 1 in, 1 out]
            n216 = property on="Pulse" class="Bool (strict)"(error in=w285, "Visible"=w290) -> (error out=w288:errorcluster)  [unwired: 1 in, 1 out]
            n217 = property on="Noise" class="Bool (strict)"(error in=w288, "Visible"=w290) -> (error out=w289:errorcluster)  [unwired: 1 in, 1 out]
            n218 = property on="DC" class="Bool (strict)"(error in=w289, "Visible"=w290) -> (error out=w272:errorcluster)  [unwired: 1 in, 1 out]
            n219 = property on="Freq" class="DigNum (strict)"(error in=w272, "Visible"=w284) -> (error out=w280:errorcluster)  [unwired: 1 in, 1 out]
            n220 = property on="Period" class="DigNum (strict)"(error in=w280, "Visible"=w284) -> (error out=w279:errorcluster)  [unwired: 1 in, 1 out]
            n221 = property on="Ampl" class="DigNum (strict)"(error in=w279, "Visible"=w284) -> (error out=w278:errorcluster)  [unwired: 1 in, 1 out]
            n222 = property on="HighL" class="DigNum (strict)"(error in=w278, "Visible"=w284) -> (error out=w281:errorcluster)  [unwired: 1 in, 1 out]
            n223 = property on="Offset" class="DigNum (strict)"(error in=w281, "Visible"=w284) -> (error out=w277:errorcluster)  [unwired: 1 in, 1 out]
            n224 = property on="LowL" class="DigNum (strict)"(error in=w277, "Visible"=w284) -> (error out=w276:errorcluster)  [unwired: 1 in, 1 out]
            n225 = property on="PhaseDBL" class="DigNum (strict)"(error in=w276, "Visible"=w284) -> (error out=w282:errorcluster)  [unwired: 1 in, 1 out]
            n226 = property on="Duty" class="DigNum (strict)"(error in=w282, "Visible"=w284) -> (error out=w283:errorcluster)  [unwired: 1 in, 1 out]
            n227 = property on="SymmDBL" class="DigNum (strict)"(error in=w283, "Visible"=w284) -> (error out=w275:errorcluster)  [unwired: 1 in, 1 out]
            n228 = property on="Width" class="DigNum (strict)"(error in=w275, "Visible"=w284) -> (error out=w274:errorcluster)  [unwired: 1 in, 1 out]
            n229 = property on="RisEdgeDBL" class="DigNum (strict)"(error in=w274, "Visible"=w284) -> (error out=w273:errorcluster)  [unwired: 1 in, 1 out]
            n230 = property on="FallEdgeDBL" class="DigNum (strict)"(error in=w273, "Visible"=w284) -> (error out=w252:errorcluster)  [unwired: 1 in, 1 out]
            n231 = property on="Freq-Period" class="Str"(error in=w252, "Visible"=w254) -> (error out=w301:errorcluster)  [unwired: 1 in, 1 out]
            n232 = property on="Freq/Period" class="Bool (strict)"(error in=w252, "Visible"=w254) -> (error out=w298:errorcluster)  [unwired: 1 in, 1 out]
            n233 = property on="Ampl-HighL" class="Str"(error in=w301, "Visible"=w254) -> (error out=w300:errorcluster)  [unwired: 1 in, 1 out]
            n234 = property on="Ampl/HighL" class="Bool (strict)"(error in=w298, "Visible"=w254) -> (error out=w297:errorcluster)  [unwired: 1 in, 1 out]
            n235 = property on="Offset-LowL" class="Str"(error in=w300, "Visible"=w254) -> (error out=w299:errorcluster)  [unwired: 1 in, 1 out]
            n236 = property on="Offset/LowL" class="Bool (strict)"(error in=w297, "Visible"=w254) -> (error out=w255:errorcluster)  [unwired: 1 in, 1 out]
            n237 = property on="PhaseStr" class="Str"(error in=w299, "Visible"=w254) -> ()  [unwired: 1 in, 2 out]
            n238 = property on="Slider" class="Bool (strict)"(error in=w255, "Visible"=w254, "Value"=FALSE ("Slider")) -> ()  [unwired: 1 in, 2 out]
            n239 = property on="Ampl/HighL" class="Bool (strict)"(error in=w252, "Top"=170 ("Position:Top")) -> (error out=w294:errorcluster)  [unwired: 1 in, 1 out]
            n240 = property on="Ampl-HighL" class="Str"(error in=w252, "Top"=167 ("Position:Top")) -> (error out=w291:errorcluster)  [unwired: 1 in, 1 out]
            n241 = property on="Offset-LowL" class="Str"(error in=w291, "Top"=209 ("Position:Top")) -> ()  [unwired: 1 in, 2 out]
            n242 = property on="Offset/LowL" class="Bool (strict)"(error in=w294, "Top"=212 ("Position:Top")) -> ()  [unwired: 1 in, 2 out]
          }
          frame 16 {
            w308 = FALSE ("Visible")
            w317 = FALSE ("Visible")
            w332 = FALSE ("Visible")
            w338 = FALSE ("Visible")
            w302 = FALSE ("Visible")
            w304 = TRUE ("Visible")
            # "Noise"
            # "AllSwapButtonsVisible?"
            # "AllStringsVisible?"
            # "AllValuesVisible?"
            # "AllWaveformsVisible?"
            n243 = property on="Freq-Period" class="Str"(error in=w305, "Visible"=w317) -> (error out=w315:errorcluster)  [unwired: 1 in, 1 out]
            n244 = property on="Ampl-HighL" class="Str"(error in=w315, "Visible"=w317) -> (error out=w314:errorcluster)  [unwired: 1 in, 1 out]
            n245 = property on="Offset-LowL" class="Str"(error in=w314, "Visible"=w317) -> (error out=w313:errorcluster)  [unwired: 1 in, 1 out]
            n246 = property on="PhaseStr" class="Str"(error in=w313, "Visible"=w317) -> (error out=w316:errorcluster)  [unwired: 1 in, 1 out]
            n247 = property on="Duty-Width" class="Str"(error in=w316, "Visible"=w317) -> (error out=w319:errorcluster)  [unwired: 1 in, 1 out]
            n248 = property on="SymmStr" class="Str"(error in=w319, "Visible"=w317) -> (error out=w318:errorcluster)  [unwired: 1 in, 1 out]
            n249 = property on="RisEdgeStr" class="Str"(error in=w318, "Visible"=w317) -> (error out=w312:errorcluster)  [unwired: 1 in, 1 out]
            n250 = property on="FallEdgeStr" class="Str"(error in=w312, "Visible"=w317) -> (error out=w307:errorcluster)  [unwired: 1 in, 1 out]
            n251 = property on="Slider" class="Bool (strict)"(error in=w305, "Visible"=w302) -> ()  [unwired: 1 in, 2 out]
            n252 = property on="OK" class="Bool (strict)"("Visible"=w302) -> ()  [unwired: 2 in, 2 out]
            n253 = property on="Freq/Period" class="Bool (strict)"(error in=w307, "Visible"=w308) -> (error out=w311:errorcluster)  [unwired: 1 in, 1 out]
            n254 = property on="Ampl/HighL" class="Bool (strict)"(error in=w311, "Visible"=w308) -> (error out=w310:errorcluster)  [unwired: 1 in, 1 out]
            n255 = property on="Offset/LowL" class="Bool (strict)"(error in=w310, "Visible"=w308) -> (error out=w309:errorcluster)  [unwired: 1 in, 1 out]
            n256 = property on="Duty/Width" class="Bool (strict)"(error in=w309, "Visible"=w308) -> (error out=w306:errorcluster)  [unwired: 1 in, 1 out]
            n257 = property on="Sine" class="Bool (strict)"(error in=w306, "Visible"=w338) -> (error out=w335:errorcluster)  [unwired: 1 in, 1 out]
            n258 = property on="Square" class="Bool (strict)"(error in=w335, "Visible"=w338) -> (error out=w334:errorcluster)  [unwired: 1 in, 1 out]
            n259 = property on="Ramp" class="Bool (strict)"(error in=w334, "Visible"=w338) -> (error out=w333:errorcluster)  [unwired: 1 in, 1 out]
            n260 = property on="Pulse" class="Bool (strict)"(error in=w333, "Visible"=w338) -> (error out=w336:errorcluster)  [unwired: 1 in, 1 out]
            n261 = property on="Noise" class="Bool (strict)"(error in=w336, "Visible"=w338) -> (error out=w337:errorcluster)  [unwired: 1 in, 1 out]
            n262 = property on="DC" class="Bool (strict)"(error in=w337, "Visible"=w338) -> (error out=w320:errorcluster)  [unwired: 1 in, 1 out]
            n263 = property on="Freq" class="DigNum (strict)"(error in=w320, "Visible"=w332) -> (error out=w328:errorcluster)  [unwired: 1 in, 1 out]
            n264 = property on="Period" class="DigNum (strict)"(error in=w328, "Visible"=w332) -> (error out=w327:errorcluster)  [unwired: 1 in, 1 out]
            n265 = property on="Ampl" class="DigNum (strict)"(error in=w327, "Visible"=w332) -> (error out=w326:errorcluster)  [unwired: 1 in, 1 out]
            n266 = property on="HighL" class="DigNum (strict)"(error in=w326, "Visible"=w332) -> (error out=w329:errorcluster)  [unwired: 1 in, 1 out]
            n267 = property on="Offset" class="DigNum (strict)"(error in=w329, "Visible"=w332) -> (error out=w325:errorcluster)  [unwired: 1 in, 1 out]
            n268 = property on="LowL" class="DigNum (strict)"(error in=w325, "Visible"=w332) -> (error out=w324:errorcluster)  [unwired: 1 in, 1 out]
            n269 = property on="PhaseDBL" class="DigNum (strict)"(error in=w324, "Visible"=w332) -> (error out=w330:errorcluster)  [unwired: 1 in, 1 out]
            n270 = property on="Duty" class="DigNum (strict)"(error in=w330, "Visible"=w332) -> (error out=w331:errorcluster)  [unwired: 1 in, 1 out]
            n271 = property on="SymmDBL" class="DigNum (strict)"(error in=w331, "Visible"=w332) -> (error out=w323:errorcluster)  [unwired: 1 in, 1 out]
            n272 = property on="Width" class="DigNum (strict)"(error in=w323, "Visible"=w332) -> (error out=w322:errorcluster)  [unwired: 1 in, 1 out]
            n273 = property on="RisEdgeDBL" class="DigNum (strict)"(error in=w322, "Visible"=w332) -> (error out=w321:errorcluster)  [unwired: 1 in, 1 out]
            n274 = property on="FallEdgeDBL" class="DigNum (strict)"(error in=w321, "Visible"=w332) -> (error out=w303:errorcluster)  [unwired: 1 in, 1 out]
            n275 = property on="Ampl-HighL" class="Str"(error in=w303, "Visible"=w304) -> (error out=w346:errorcluster)  [unwired: 1 in, 1 out]
            n276 = property on="Ampl/HighL" class="Bool (strict)"(error in=w303, "Visible"=w304) -> (error out=w345:errorcluster)  [unwired: 1 in, 1 out]
            n277 = property on="Offset-LowL" class="Str"(error in=w346, "Visible"=w304) -> ()  [unwired: 1 in, 2 out]
            n278 = property on="Offset/LowL" class="Bool (strict)"(error in=w345, "Visible"=w304) -> ()  [unwired: 1 in, 2 out]
            n279 = property on="Ampl/HighL" class="Bool (strict)"(error in=w303, "Top"=128 ("Position:Top")) -> (error out=w342:errorcluster)  [unwired: 1 in, 1 out]
            n280 = property on="Ampl-HighL" class="Str"(error in=w303, "Top"=125 ("Position:Top")) -> (error out=w339:errorcluster)  [unwired: 1 in, 1 out]
            n281 = property on="Offset-LowL" class="Str"(error in=w339, "Top"=167 ("Position:Top")) -> ()  [unwired: 1 in, 2 out]
            n282 = property on="Offset/LowL" class="Bool (strict)"(error in=w342, "Top"=170 ("Position:Top")) -> ()  [unwired: 1 in, 2 out]
          }
          frame 32 {
            w353 = FALSE ("Visible")
            w362 = FALSE ("Visible")
            w379 = FALSE ("Visible")
            w385 = FALSE ("Visible")
            w348 = FALSE ("Visible")
            # "DC"
            # "Force Ampl to go 0 (at OK)"
            # "AllSwapButtonsVisible?"
            # "AllStringsVisible?"
            # "AllValuesVisible?"
            # "AllWaveformsVisible?"
            n283 = property on="Freq-Period" class="Str"(error in=w350, "Visible"=w362) -> (error out=w360:errorcluster)  [unwired: 1 in, 1 out]
            n284 = property on="Ampl-HighL" class="Str"(error in=w360, "Visible"=w362) -> (error out=w359:errorcluster)  [unwired: 1 in, 1 out]
            n285 = property on="Offset-LowL" class="Str"(error in=w359, "Visible"=w362) -> (error out=w358:errorcluster)  [unwired: 1 in, 1 out]
            n286 = property on="PhaseStr" class="Str"(error in=w358, "Visible"=w362) -> (error out=w361:errorcluster)  [unwired: 1 in, 1 out]
            n287 = property on="Duty-Width" class="Str"(error in=w361, "Visible"=w362) -> (error out=w364:errorcluster)  [unwired: 1 in, 1 out]
            n288 = property on="SymmStr" class="Str"(error in=w364, "Visible"=w362) -> (error out=w363:errorcluster)  [unwired: 1 in, 1 out]
            n289 = property on="RisEdgeStr" class="Str"(error in=w363, "Visible"=w362) -> (error out=w357:errorcluster)  [unwired: 1 in, 1 out]
            n290 = property on="FallEdgeStr" class="Str"(error in=w357, "Visible"=w362) -> (error out=w352:errorcluster)  [unwired: 1 in, 1 out]
            n291 = property on="Slider" class="Bool (strict)"(error in=w350, "Visible"=w348) -> ()  [unwired: 1 in, 2 out]
            n292 = property on="OK" class="Bool (strict)"("Visible"=w348) -> (error out=w349:errorcluster)  [unwired: 2 in, 1 out]
            n293 = property on="Freq/Period" class="Bool (strict)"(error in=w352, "Visible"=w353) -> (error out=w356:errorcluster)  [unwired: 1 in, 1 out]
            n294 = property on="Ampl/HighL" class="Bool (strict)"(error in=w356, "Visible"=w353) -> (error out=w355:errorcluster)  [unwired: 1 in, 1 out]
            n295 = property on="Offset/LowL" class="Bool (strict)"(error in=w355, "Visible"=w353) -> (error out=w354:errorcluster)  [unwired: 1 in, 1 out]
            n296 = property on="Duty/Width" class="Bool (strict)"(error in=w354, "Visible"=w353) -> (error out=w351:errorcluster)  [unwired: 1 in, 1 out]
            n297 = property on="Offset/LowL" class="Bool (strict)"(error in=w349, "Value"=w348) -> ()  [unwired: 1 in, 2 out]
            n298 = property on="Sine" class="Bool (strict)"(error in=w351, "Visible"=w385) -> (error out=w382:errorcluster)  [unwired: 1 in, 1 out]
            n299 = property on="Square" class="Bool (strict)"(error in=w382, "Visible"=w385) -> (error out=w381:errorcluster)  [unwired: 1 in, 1 out]
            n300 = property on="Ramp" class="Bool (strict)"(error in=w381, "Visible"=w385) -> (error out=w380:errorcluster)  [unwired: 1 in, 1 out]
            n301 = property on="Pulse" class="Bool (strict)"(error in=w380, "Visible"=w385) -> (error out=w383:errorcluster)  [unwired: 1 in, 1 out]
            n302 = property on="Noise" class="Bool (strict)"(error in=w383, "Visible"=w385) -> (error out=w384:errorcluster)  [unwired: 1 in, 1 out]
            n303 = property on="DC" class="Bool (strict)"(error in=w384, "Visible"=w385) -> (error out=w367:errorcluster)  [unwired: 1 in, 1 out]
            n304 = local write "Ampl"(0.0 ("Ampl")) -> ()
            n305 = property on="Freq" class="DigNum (strict)"(error in=w367, "Visible"=w379) -> (error out=w375:errorcluster)  [unwired: 1 in, 1 out]
            n306 = property on="Period" class="DigNum (strict)"(error in=w375, "Visible"=w379) -> (error out=w374:errorcluster)  [unwired: 1 in, 1 out]
            n307 = property on="Ampl" class="DigNum (strict)"(error in=w374, "Visible"=w379) -> (error out=w373:errorcluster)  [unwired: 1 in, 1 out]
            n308 = property on="HighL" class="DigNum (strict)"(error in=w373, "Visible"=w379) -> (error out=w376:errorcluster)  [unwired: 1 in, 1 out]
            n309 = property on="Offset" class="DigNum (strict)"(error in=w376, "Visible"=w379) -> (error out=w372:errorcluster)  [unwired: 1 in, 1 out]
            n310 = property on="LowL" class="DigNum (strict)"(error in=w372, "Visible"=w379) -> (error out=w371:errorcluster)  [unwired: 1 in, 1 out]
            n311 = property on="PhaseDBL" class="DigNum (strict)"(error in=w371, "Visible"=w379) -> (error out=w377:errorcluster)  [unwired: 1 in, 1 out]
            n312 = property on="Duty" class="DigNum (strict)"(error in=w377, "Visible"=w379) -> (error out=w378:errorcluster)  [unwired: 1 in, 1 out]
            n313 = property on="SymmDBL" class="DigNum (strict)"(error in=w378, "Visible"=w379) -> (error out=w370:errorcluster)  [unwired: 1 in, 1 out]
            n314 = property on="Width" class="DigNum (strict)"(error in=w370, "Visible"=w379) -> (error out=w369:errorcluster)  [unwired: 1 in, 1 out]
            n315 = property on="RisEdgeDBL" class="DigNum (strict)"(error in=w369, "Visible"=w379) -> (error out=w368:errorcluster)  [unwired: 1 in, 1 out]
            n316 = property on="FallEdgeDBL" class="DigNum (strict)"(error in=w368, "Visible"=w379) -> (error out=w366:errorcluster)  [unwired: 1 in, 1 out]
            n317 = property on="Offset-LowL" class="Str"(error in=w366, "Visible"=TRUE) -> (error out=w365:errorcluster)  [unwired: 1 in, 1 out]
            n318 = property on="Ampl/HighL" class="Bool (strict)"(error in=w365, "Top"=170 ("Position:Top")) -> (error out=w389:errorcluster)  [unwired: 1 in, 1 out]
            n319 = property on="Ampl-HighL" class="Str"(error in=w365, "Top"=167 ("Position:Top")) -> (error out=w386:errorcluster)  [unwired: 1 in, 1 out]
            n320 = property on="Offset-LowL" class="Str"(error in=w386, "Top"=125 ("Position:Top")) -> ()  [unwired: 1 in, 2 out]
            n321 = property on="Offset/LowL" class="Bool (strict)"(error in=w389, "Top"=212 ("Position:Top")) -> ()  [unwired: 1 in, 2 out]
          }
        }
        n322 = case shown="1, Default" w71 {
          tunnel: ["Home_Sine.bmp" "Home_Square_1.bmp" "Home_Ramp_1.bmp" "Home_Pulse_1.bmp" "Home_Noise.bmp" "Home_DC.bmp"] -> w94
          tunnel: w82 -> [w393 w395 w397 w399 w401 w403]
          tunnel: [w393 w395 w397 w399 w401 w403] -> w84
          frame 1, Default {
          }
          frame 2 {
          }
          frame 4 {
          }
          frame 8 {
          }
          frame 16 {
          }
          frame 32 {
          }
        }
        n323 = Build Path(base path=w93, name or relative path=w94) -> (appended path=w103:path)
        n324 = call "RDG822 Update Screen.vi"("error in"=w84, "Path to file"=w103) -> ("error out"=w89:errorcluster, "Screen"=w102:picture)  [unwired: 8 in]
        n325 = local write "MenuCount"(w71) -> ()
        n326 = call "Time Delay4"("error in (no error)"=w89) -> ("error out"=w91:errorcluster)  [unwired: 10 in]
        n327 = local write "Screen"(w102) -> ()
        n328 = local write "error out"(w89) -> ()
        n329 = property on="Home" class="Bool (strict)"(error in=w91, "Value"=FALSE ("Home")) -> ()  [unwired: 1 in, 2 out]
        n330 = call "RDG822 Menu.vi"("MenuID"=w71) -> ("Sine"=w77:bool, "Square"=w76:bool, "Ramp"=w75:bool, "Pulse"=w74:bool, "Noise"=w73:bool, "DC"=w72:bool)  [unwired: 13 in]
        n331 = property on="Sine" class="Bool (strict)"("Value"=w77) -> ()  [unwired: 2 in, 2 out]
        n332 = property on="Square" class="Bool (strict)"("Value"=w76) -> ()  [unwired: 2 in, 2 out]
        n333 = property on="Ramp" class="Bool (strict)"("Value"=w75) -> ()  [unwired: 2 in, 2 out]
        n334 = property on="Pulse" class="Bool (strict)"("Value"=w74) -> ()  [unwired: 2 in, 2 out]
        n335 = property on="Noise" class="Bool (strict)"("Value"=w73) -> ()  [unwired: 2 in, 2 out]
        n336 = property on="DC" class="Bool (strict)"("Value"=w72) -> ()  [unwired: 2 in, 2 out]
      }
      event "Slider": Value Change {
        n337 = event-data() -> ()  [unwired: 1 in, 6 out]
        n338 = local read "Slider"() -> (w406:bool)
        n339 = local read "MenuCount"() -> (w407:u32)
        n340 = case shown="8" w407 {
          tunnel: w408 -> [w426 w508 w590]
          tunnel: w406 -> [w425 w507 w589]
          frame 2, Default {
            # "Square"
            n341 = case shown="True" w425 {
              tunnel: w426 -> [w430 w474]
              frame False {
                w433 = FALSE ("Visible")
                w442 = FALSE ("Visible")
                w428 = FALSE ("Visible")
                w462 = FALSE ("Visible")
                w463 = TRUE ("Visible")
                # "AllSwapButtonsVisible?"
                # "AllStringsVisible?"
                # "AllValuesVisible?"
                # "AllWaveformsVisible?"
                n342 = property on="Freq-Period" class="Str"(error in=w430, "Visible"=w442) -> (error out=w440:errorcluster)  [unwired: 1 in, 1 out]
                n343 = property on="Ampl-HighL" class="Str"(error in=w440, "Visible"=w442) -> (error out=w439:errorcluster)  [unwired: 1 in, 1 out]
                n344 = property on="Offset-LowL" class="Str"(error in=w439, "Visible"=w442) -> (error out=w438:errorcluster)  [unwired: 1 in, 1 out]
                n345 = property on="PhaseStr" class="Str"(error in=w438, "Visible"=w442) -> (error out=w441:errorcluster)  [unwired: 1 in, 1 out]
                n346 = property on="Duty-Width" class="Str"(error in=w441, "Visible"=w442) -> (error out=w444:errorcluster)  [unwired: 1 in, 1 out]
                n347 = property on="SymmStr" class="Str"(error in=w444, "Visible"=w442) -> (error out=w443:errorcluster)  [unwired: 1 in, 1 out]
                n348 = property on="RisEdgeStr" class="Str"(error in=w443, "Visible"=w442) -> (error out=w437:errorcluster)  [unwired: 1 in, 1 out]
                n349 = property on="FallEdgeStr" class="Str"(error in=w437, "Visible"=w442) -> (error out=w432:errorcluster)  [unwired: 1 in, 1 out]
                n350 = property on="Freq/Period" class="Bool (strict)"(error in=w432, "Visible"=w433) -> (error out=w436:errorcluster)  [unwired: 1 in, 1 out]
                n351 = property on="Ampl/HighL" class="Bool (strict)"(error in=w436, "Visible"=w433) -> (error out=w435:errorcluster)  [unwired: 1 in, 1 out]
                n352 = property on="Offset/LowL" class="Bool (strict)"(error in=w435, "Visible"=w433) -> (error out=w434:errorcluster)  [unwired: 1 in, 1 out]
                n353 = property on="Duty/Width" class="Bool (strict)"(error in=w434, "Visible"=w433) -> (error out=w431:errorcluster)  [unwired: 1 in, 1 out]
                n354 = property on="Sine" class="Bool (strict)"(error in=w431, "Visible"=w462) -> (error out=w459:errorcluster)  [unwired: 1 in, 1 out]
                n355 = property on="Square" class="Bool (strict)"(error in=w459, "Visible"=w462) -> (error out=w458:errorcluster)  [unwired: 1 in, 1 out]
                n356 = property on="Ramp" class="Bool (strict)"(error in=w458, "Visible"=w462) -> (error out=w457:errorcluster)  [unwired: 1 in, 1 out]
                n357 = property on="Pulse" class="Bool (strict)"(error in=w457, "Visible"=w462) -> (error out=w460:errorcluster)  [unwired: 1 in, 1 out]
                n358 = property on="Noise" class="Bool (strict)"(error in=w460, "Visible"=w462) -> (error out=w461:errorcluster)  [unwired: 1 in, 1 out]
                n359 = property on="DC" class="Bool (strict)"(error in=w461, "Visible"=w462) -> (error out=w445:errorcluster)  [unwired: 1 in, 1 out]
                n360 = property on="Freq" class="DigNum (strict)"(error in=w445, "Visible"=w428) -> (error out=w453:errorcluster)  [unwired: 1 in, 1 out]
                n361 = property on="Period" class="DigNum (strict)"(error in=w453, "Visible"=w428) -> (error out=w452:errorcluster)  [unwired: 1 in, 1 out]
                n362 = property on="Ampl" class="DigNum (strict)"(error in=w452, "Visible"=w428) -> (error out=w451:errorcluster)  [unwired: 1 in, 1 out]
                n363 = property on="HighL" class="DigNum (strict)"(error in=w451, "Visible"=w428) -> (error out=w454:errorcluster)  [unwired: 1 in, 1 out]
                n364 = property on="Offset" class="DigNum (strict)"(error in=w454, "Visible"=w428) -> (error out=w450:errorcluster)  [unwired: 1 in, 1 out]
                n365 = property on="LowL" class="DigNum (strict)"(error in=w450, "Visible"=w428) -> (error out=w449:errorcluster)  [unwired: 1 in, 1 out]
                n366 = property on="PhaseDBL" class="DigNum (strict)"(error in=w449, "Visible"=w428) -> (error out=w455:errorcluster)  [unwired: 1 in, 1 out]
                n367 = property on="Duty" class="DigNum (strict)"(error in=w455, "Visible"=w428) -> (error out=w456:errorcluster)  [unwired: 1 in, 1 out]
                n368 = property on="SymmDBL" class="DigNum (strict)"(error in=w456, "Visible"=w428) -> (error out=w448:errorcluster)  [unwired: 1 in, 1 out]
                n369 = property on="Width" class="DigNum (strict)"(error in=w448, "Visible"=w428) -> (error out=w447:errorcluster)  [unwired: 1 in, 1 out]
                n370 = property on="RisEdgeDBL" class="DigNum (strict)"(error in=w447, "Visible"=w428) -> (error out=w446:errorcluster)  [unwired: 1 in, 1 out]
                n371 = property on="FallEdgeDBL" class="DigNum (strict)"(error in=w446, "Visible"=w428) -> (error out=w429:errorcluster)  [unwired: 1 in, 1 out]
                n372 = property on="OK" class="Bool (strict)"(error in=w429, "Visible"=w428) -> (error out=w427:errorcluster)  [unwired: 1 in, 1 out]
                n373 = property on="Freq-Period" class="Str"(error in=w427, "Visible"=w463) -> (error out=w469:errorcluster)  [unwired: 1 in, 1 out]
                n374 = property on="Freq/Period" class="Bool (strict)"(error in=w427, "Visible"=w463) -> (error out=w466:errorcluster)  [unwired: 1 in, 1 out]
                n375 = property on="Ampl-HighL" class="Str"(error in=w469, "Visible"=w463) -> (error out=w468:errorcluster)  [unwired: 1 in, 1 out]
                n376 = property on="Ampl/HighL" class="Bool (strict)"(error in=w466, "Visible"=w463) -> (error out=w465:errorcluster)  [unwired: 1 in, 1 out]
                n377 = property on="Offset-LowL" class="Str"(error in=w468, "Visible"=w463) -> (error out=w467:errorcluster)  [unwired: 1 in, 1 out]
                n378 = property on="Offset/LowL" class="Bool (strict)"(error in=w465, "Visible"=w463) -> (error out=w464:errorcluster)  [unwired: 1 in, 1 out]
                n379 = property on="PhaseStr" class="Str"(error in=w467, "Visible"=w463) -> ()  [unwired: 1 in, 2 out]
                n380 = property on="Slider" class="Bool (strict)"(error in=w464, "Visible"=w463) -> ()  [unwired: 1 in, 2 out]
              }
              frame True {
                w477 = FALSE ("Visible")
                w486 = FALSE ("Visible")
                w472 = FALSE ("Visible")
                w506 = FALSE ("Visible")
                w471 = TRUE ("Visible")
                # "AllSwapButtonsVisible?"
                # "AllStringsVisible?"
                # "AllValuesVisible?"
                # "AllWaveformsVisible?"
                n381 = property on="Freq-Period" class="Str"(error in=w474, "Visible"=w486) -> (error out=w484:errorcluster)  [unwired: 1 in, 1 out]
                n382 = property on="Ampl-HighL" class="Str"(error in=w484, "Visible"=w486) -> (error out=w483:errorcluster)  [unwired: 1 in, 1 out]
                n383 = property on="Offset-LowL" class="Str"(error in=w483, "Visible"=w486) -> (error out=w482:errorcluster)  [unwired: 1 in, 1 out]
                n384 = property on="PhaseStr" class="Str"(error in=w482, "Visible"=w486) -> (error out=w485:errorcluster)  [unwired: 1 in, 1 out]
                n385 = property on="Duty-Width" class="Str"(error in=w485, "Visible"=w486) -> (error out=w488:errorcluster)  [unwired: 1 in, 1 out]
                n386 = property on="SymmStr" class="Str"(error in=w488, "Visible"=w486) -> (error out=w487:errorcluster)  [unwired: 1 in, 1 out]
                n387 = property on="RisEdgeStr" class="Str"(error in=w487, "Visible"=w486) -> (error out=w481:errorcluster)  [unwired: 1 in, 1 out]
                n388 = property on="FallEdgeStr" class="Str"(error in=w481, "Visible"=w486) -> (error out=w476:errorcluster)  [unwired: 1 in, 1 out]
                n389 = property on="Freq/Period" class="Bool (strict)"(error in=w476, "Visible"=w477) -> (error out=w480:errorcluster)  [unwired: 1 in, 1 out]
                n390 = property on="Ampl/HighL" class="Bool (strict)"(error in=w480, "Visible"=w477) -> (error out=w479:errorcluster)  [unwired: 1 in, 1 out]
                n391 = property on="Offset/LowL" class="Bool (strict)"(error in=w479, "Visible"=w477) -> (error out=w478:errorcluster)  [unwired: 1 in, 1 out]
                n392 = property on="Duty/Width" class="Bool (strict)"(error in=w478, "Visible"=w477) -> (error out=w475:errorcluster)  [unwired: 1 in, 1 out]
                n393 = property on="Sine" class="Bool (strict)"(error in=w475, "Visible"=w506) -> (error out=w503:errorcluster)  [unwired: 1 in, 1 out]
                n394 = property on="Square" class="Bool (strict)"(error in=w503, "Visible"=w506) -> (error out=w502:errorcluster)  [unwired: 1 in, 1 out]
                n395 = property on="Ramp" class="Bool (strict)"(error in=w502, "Visible"=w506) -> (error out=w501:errorcluster)  [unwired: 1 in, 1 out]
                n396 = property on="Pulse" class="Bool (strict)"(error in=w501, "Visible"=w506) -> (error out=w504:errorcluster)  [unwired: 1 in, 1 out]
                n397 = property on="Noise" class="Bool (strict)"(error in=w504, "Visible"=w506) -> (error out=w505:errorcluster)  [unwired: 1 in, 1 out]
                n398 = property on="DC" class="Bool (strict)"(error in=w505, "Visible"=w506) -> (error out=w489:errorcluster)  [unwired: 1 in, 1 out]
                n399 = property on="Freq" class="DigNum (strict)"(error in=w489, "Visible"=w472) -> (error out=w497:errorcluster)  [unwired: 1 in, 1 out]
                n400 = property on="Period" class="DigNum (strict)"(error in=w497, "Visible"=w472) -> (error out=w496:errorcluster)  [unwired: 1 in, 1 out]
                n401 = property on="Ampl" class="DigNum (strict)"(error in=w496, "Visible"=w472) -> (error out=w495:errorcluster)  [unwired: 1 in, 1 out]
                n402 = property on="HighL" class="DigNum (strict)"(error in=w495, "Visible"=w472) -> (error out=w498:errorcluster)  [unwired: 1 in, 1 out]
                n403 = property on="Offset" class="DigNum (strict)"(error in=w498, "Visible"=w472) -> (error out=w494:errorcluster)  [unwired: 1 in, 1 out]
                n404 = property on="LowL" class="DigNum (strict)"(error in=w494, "Visible"=w472) -> (error out=w493:errorcluster)  [unwired: 1 in, 1 out]
                n405 = property on="PhaseDBL" class="DigNum (strict)"(error in=w493, "Visible"=w472) -> (error out=w499:errorcluster)  [unwired: 1 in, 1 out]
                n406 = property on="Duty" class="DigNum (strict)"(error in=w499, "Visible"=w472) -> (error out=w500:errorcluster)  [unwired: 1 in, 1 out]
                n407 = property on="SymmDBL" class="DigNum (strict)"(error in=w500, "Visible"=w472) -> (error out=w492:errorcluster)  [unwired: 1 in, 1 out]
                n408 = property on="Width" class="DigNum (strict)"(error in=w492, "Visible"=w472) -> (error out=w491:errorcluster)  [unwired: 1 in, 1 out]
                n409 = property on="RisEdgeDBL" class="DigNum (strict)"(error in=w491, "Visible"=w472) -> (error out=w490:errorcluster)  [unwired: 1 in, 1 out]
                n410 = property on="FallEdgeDBL" class="DigNum (strict)"(error in=w490, "Visible"=w472) -> (error out=w473:errorcluster)  [unwired: 1 in, 1 out]
                n411 = property on="OK" class="Bool (strict)"(error in=w473, "Visible"=w472) -> (error out=w470:errorcluster)  [unwired: 1 in, 1 out]
                n412 = property on="Duty-Width" class="Str"(error in=w470, "Visible"=w471) -> ()  [unwired: 1 in, 2 out]
                n413 = property on="Slider" class="Bool (strict)"(error in=w470, "Visible"=w471) -> ()  [unwired: 1 in, 2 out]
              }
            }
          }
          frame 4 {
            # "Ramp"
            n414 = case shown="False" w507 {
              tunnel: w508 -> [w512 w556]
              frame False {
                w515 = FALSE ("Visible")
                w524 = FALSE ("Visible")
                w510 = FALSE ("Visible")
                w544 = FALSE ("Visible")
                w545 = TRUE ("Visible")
                # "AllSwapButtonsVisible?"
                # "AllStringsVisible?"
                # "AllValuesVisible?"
                # "AllWaveformsVisible?"
                n415 = property on="Freq-Period" class="Str"(error in=w512, "Visible"=w524) -> (error out=w522:errorcluster)  [unwired: 1 in, 1 out]
                n416 = property on="Ampl-HighL" class="Str"(error in=w522, "Visible"=w524) -> (error out=w521:errorcluster)  [unwired: 1 in, 1 out]
                n417 = property on="Offset-LowL" class="Str"(error in=w521, "Visible"=w524) -> (error out=w520:errorcluster)  [unwired: 1 in, 1 out]
                n418 = property on="PhaseStr" class="Str"(error in=w520, "Visible"=w524) -> (error out=w523:errorcluster)  [unwired: 1 in, 1 out]
                n419 = property on="Duty-Width" class="Str"(error in=w523, "Visible"=w524) -> (error out=w526:errorcluster)  [unwired: 1 in, 1 out]
                n420 = property on="SymmStr" class="Str"(error in=w526, "Visible"=w524) -> (error out=w525:errorcluster)  [unwired: 1 in, 1 out]
                n421 = property on="RisEdgeStr" class="Str"(error in=w525, "Visible"=w524) -> (error out=w519:errorcluster)  [unwired: 1 in, 1 out]
                n422 = property on="FallEdgeStr" class="Str"(error in=w519, "Visible"=w524) -> (error out=w514:errorcluster)  [unwired: 1 in, 1 out]
                n423 = property on="Freq/Period" class="Bool (strict)"(error in=w514, "Visible"=w515) -> (error out=w518:errorcluster)  [unwired: 1 in, 1 out]
                n424 = property on="Ampl/HighL" class="Bool (strict)"(error in=w518, "Visible"=w515) -> (error out=w517:errorcluster)  [unwired: 1 in, 1 out]
                n425 = property on="Offset/LowL" class="Bool (strict)"(error in=w517, "Visible"=w515) -> (error out=w516:errorcluster)  [unwired: 1 in, 1 out]
                n426 = property on="Duty/Width" class="Bool (strict)"(error in=w516, "Visible"=w515) -> (error out=w513:errorcluster)  [unwired: 1 in, 1 out]
                n427 = property on="Sine" class="Bool (strict)"(error in=w513, "Visible"=w544) -> (error out=w541:errorcluster)  [unwired: 1 in, 1 out]
                n428 = property on="Square" class="Bool (strict)"(error in=w541, "Visible"=w544) -> (error out=w540:errorcluster)  [unwired: 1 in, 1 out]
                n429 = property on="Ramp" class="Bool (strict)"(error in=w540, "Visible"=w544) -> (error out=w539:errorcluster)  [unwired: 1 in, 1 out]
                n430 = property on="Pulse" class="Bool (strict)"(error in=w539, "Visible"=w544) -> (error out=w542:errorcluster)  [unwired: 1 in, 1 out]
                n431 = property on="Noise" class="Bool (strict)"(error in=w542, "Visible"=w544) -> (error out=w543:errorcluster)  [unwired: 1 in, 1 out]
                n432 = property on="DC" class="Bool (strict)"(error in=w543, "Visible"=w544) -> (error out=w527:errorcluster)  [unwired: 1 in, 1 out]
                n433 = property on="Freq" class="DigNum (strict)"(error in=w527, "Visible"=w510) -> (error out=w535:errorcluster)  [unwired: 1 in, 1 out]
                n434 = property on="Period" class="DigNum (strict)"(error in=w535, "Visible"=w510) -> (error out=w534:errorcluster)  [unwired: 1 in, 1 out]
                n435 = property on="Ampl" class="DigNum (strict)"(error in=w534, "Visible"=w510) -> (error out=w533:errorcluster)  [unwired: 1 in, 1 out]
                n436 = property on="HighL" class="DigNum (strict)"(error in=w533, "Visible"=w510) -> (error out=w536:errorcluster)  [unwired: 1 in, 1 out]
                n437 = property on="Offset" class="DigNum (strict)"(error in=w536, "Visible"=w510) -> (error out=w532:errorcluster)  [unwired: 1 in, 1 out]
                n438 = property on="LowL" class="DigNum (strict)"(error in=w532, "Visible"=w510) -> (error out=w531:errorcluster)  [unwired: 1 in, 1 out]
                n439 = property on="PhaseDBL" class="DigNum (strict)"(error in=w531, "Visible"=w510) -> (error out=w537:errorcluster)  [unwired: 1 in, 1 out]
                n440 = property on="Duty" class="DigNum (strict)"(error in=w537, "Visible"=w510) -> (error out=w538:errorcluster)  [unwired: 1 in, 1 out]
                n441 = property on="SymmDBL" class="DigNum (strict)"(error in=w538, "Visible"=w510) -> (error out=w530:errorcluster)  [unwired: 1 in, 1 out]
                n442 = property on="Width" class="DigNum (strict)"(error in=w530, "Visible"=w510) -> (error out=w529:errorcluster)  [unwired: 1 in, 1 out]
                n443 = property on="RisEdgeDBL" class="DigNum (strict)"(error in=w529, "Visible"=w510) -> (error out=w528:errorcluster)  [unwired: 1 in, 1 out]
                n444 = property on="FallEdgeDBL" class="DigNum (strict)"(error in=w528, "Visible"=w510) -> (error out=w511:errorcluster)  [unwired: 1 in, 1 out]
                n445 = property on="OK" class="Bool (strict)"(error in=w511, "Visible"=w510) -> (error out=w509:errorcluster)  [unwired: 1 in, 1 out]
                n446 = property on="Freq-Period" class="Str"(error in=w509, "Visible"=w545) -> (error out=w551:errorcluster)  [unwired: 1 in, 1 out]
                n447 = property on="Freq/Period" class="Bool (strict)"(error in=w509, "Visible"=w545) -> (error out=w548:errorcluster)  [unwired: 1 in, 1 out]
                n448 = property on="Ampl-HighL" class="Str"(error in=w551, "Visible"=w545) -> (error out=w550:errorcluster)  [unwired: 1 in, 1 out]
                n449 = property on="Ampl/HighL" class="Bool (strict)"(error in=w548, "Visible"=w545) -> (error out=w547:errorcluster)  [unwired: 1 in, 1 out]
                n450 = property on="Offset-LowL" class="Str"(error in=w550, "Visible"=w545) -> (error out=w549:errorcluster)  [unwired: 1 in, 1 out]
                n451 = property on="Offset/LowL" class="Bool (strict)"(error in=w547, "Visible"=w545) -> (error out=w546:errorcluster)  [unwired: 1 in, 1 out]
                n452 = property on="PhaseStr" class="Str"(error in=w549, "Visible"=w545) -> ()  [unwired: 1 in, 2 out]
                n453 = property on="Slider" class="Bool (strict)"(error in=w546, "Visible"=w545) -> ()  [unwired: 1 in, 2 out]
              }
              frame True {
                w559 = FALSE ("Visible")
                w568 = FALSE ("Visible")
                w554 = FALSE ("Visible")
                w588 = FALSE ("Visible")
                w553 = TRUE ("Visible")
                # "AllSwapButtonsVisible?"
                # "AllStringsVisible?"
                # "AllValuesVisible?"
                # "AllWaveformsVisible?"
                n454 = property on="Freq-Period" class="Str"(error in=w556, "Visible"=w568) -> (error out=w566:errorcluster)  [unwired: 1 in, 1 out]
                n455 = property on="Ampl-HighL" class="Str"(error in=w566, "Visible"=w568) -> (error out=w565:errorcluster)  [unwired: 1 in, 1 out]
                n456 = property on="Offset-LowL" class="Str"(error in=w565, "Visible"=w568) -> (error out=w564:errorcluster)  [unwired: 1 in, 1 out]
                n457 = property on="PhaseStr" class="Str"(error in=w564, "Visible"=w568) -> (error out=w567:errorcluster)  [unwired: 1 in, 1 out]
                n458 = property on="Duty-Width" class="Str"(error in=w567, "Visible"=w568) -> (error out=w570:errorcluster)  [unwired: 1 in, 1 out]
                n459 = property on="SymmStr" class="Str"(error in=w570, "Visible"=w568) -> (error out=w569:errorcluster)  [unwired: 1 in, 1 out]
                n460 = property on="RisEdgeStr" class="Str"(error in=w569, "Visible"=w568) -> (error out=w563:errorcluster)  [unwired: 1 in, 1 out]
                n461 = property on="FallEdgeStr" class="Str"(error in=w563, "Visible"=w568) -> (error out=w558:errorcluster)  [unwired: 1 in, 1 out]
                n462 = property on="Freq/Period" class="Bool (strict)"(error in=w558, "Visible"=w559) -> (error out=w562:errorcluster)  [unwired: 1 in, 1 out]
                n463 = property on="Ampl/HighL" class="Bool (strict)"(error in=w562, "Visible"=w559) -> (error out=w561:errorcluster)  [unwired: 1 in, 1 out]
                n464 = property on="Offset/LowL" class="Bool (strict)"(error in=w561, "Visible"=w559) -> (error out=w560:errorcluster)  [unwired: 1 in, 1 out]
                n465 = property on="Duty/Width" class="Bool (strict)"(error in=w560, "Visible"=w559) -> (error out=w557:errorcluster)  [unwired: 1 in, 1 out]
                n466 = property on="Sine" class="Bool (strict)"(error in=w557, "Visible"=w588) -> (error out=w585:errorcluster)  [unwired: 1 in, 1 out]
                n467 = property on="Square" class="Bool (strict)"(error in=w585, "Visible"=w588) -> (error out=w584:errorcluster)  [unwired: 1 in, 1 out]
                n468 = property on="Ramp" class="Bool (strict)"(error in=w584, "Visible"=w588) -> (error out=w583:errorcluster)  [unwired: 1 in, 1 out]
                n469 = property on="Pulse" class="Bool (strict)"(error in=w583, "Visible"=w588) -> (error out=w586:errorcluster)  [unwired: 1 in, 1 out]
                n470 = property on="Noise" class="Bool (strict)"(error in=w586, "Visible"=w588) -> (error out=w587:errorcluster)  [unwired: 1 in, 1 out]
                n471 = property on="DC" class="Bool (strict)"(error in=w587, "Visible"=w588) -> (error out=w571:errorcluster)  [unwired: 1 in, 1 out]
                n472 = property on="Freq" class="DigNum (strict)"(error in=w571, "Visible"=w554) -> (error out=w579:errorcluster)  [unwired: 1 in, 1 out]
                n473 = property on="Period" class="DigNum (strict)"(error in=w579, "Visible"=w554) -> (error out=w578:errorcluster)  [unwired: 1 in, 1 out]
                n474 = property on="Ampl" class="DigNum (strict)"(error in=w578, "Visible"=w554) -> (error out=w577:errorcluster)  [unwired: 1 in, 1 out]
                n475 = property on="HighL" class="DigNum (strict)"(error in=w577, "Visible"=w554) -> (error out=w580:errorcluster)  [unwired: 1 in, 1 out]
                n476 = property on="Offset" class="DigNum (strict)"(error in=w580, "Visible"=w554) -> (error out=w576:errorcluster)  [unwired: 1 in, 1 out]
                n477 = property on="LowL" class="DigNum (strict)"(error in=w576, "Visible"=w554) -> (error out=w575:errorcluster)  [unwired: 1 in, 1 out]
                n478 = property on="PhaseDBL" class="DigNum (strict)"(error in=w575, "Visible"=w554) -> (error out=w581:errorcluster)  [unwired: 1 in, 1 out]
                n479 = property on="Duty" class="DigNum (strict)"(error in=w581, "Visible"=w554) -> (error out=w582:errorcluster)  [unwired: 1 in, 1 out]
                n480 = property on="SymmDBL" class="DigNum (strict)"(error in=w582, "Visible"=w554) -> (error out=w574:errorcluster)  [unwired: 1 in, 1 out]
                n481 = property on="Width" class="DigNum (strict)"(error in=w574, "Visible"=w554) -> (error out=w573:errorcluster)  [unwired: 1 in, 1 out]
                n482 = property on="RisEdgeDBL" class="DigNum (strict)"(error in=w573, "Visible"=w554) -> (error out=w572:errorcluster)  [unwired: 1 in, 1 out]
                n483 = property on="FallEdgeDBL" class="DigNum (strict)"(error in=w572, "Visible"=w554) -> (error out=w555:errorcluster)  [unwired: 1 in, 1 out]
                n484 = property on="OK" class="Bool (strict)"(error in=w555, "Visible"=w554) -> (error out=w552:errorcluster)  [unwired: 1 in, 1 out]
                n485 = property on="SymmStr" class="Str"(error in=w552, "Visible"=w553) -> ()  [unwired: 1 in, 2 out]
                n486 = property on="Slider" class="Bool (strict)"(error in=w552, "Visible"=w553) -> ()  [unwired: 1 in, 2 out]
              }
            }
          }
          frame 8 {
            # "Pulse"
            n487 = case shown="False" w589 {
              tunnel: w590 -> [w594 w641]
              frame False {
                w597 = FALSE ("Visible")
                w606 = FALSE ("Visible")
                w592 = FALSE ("Visible")
                w626 = FALSE ("Visible")
                w627 = TRUE ("Visible")
                # "AllSwapButtonsVisible?"
                # "AllStringsVisible?"
                # "AllValuesVisible?"
                # "AllWaveformsVisible?"
                n488 = property on="Freq-Period" class="Str"(error in=w594, "Visible"=w606) -> (error out=w604:errorcluster)  [unwired: 1 in, 1 out]
                n489 = property on="Ampl-HighL" class="Str"(error in=w604, "Visible"=w606) -> (error out=w603:errorcluster)  [unwired: 1 in, 1 out]
                n490 = property on="Offset-LowL" class="Str"(error in=w603, "Visible"=w606) -> (error out=w602:errorcluster)  [unwired: 1 in, 1 out]
                n491 = property on="PhaseStr" class="Str"(error in=w602, "Visible"=w606) -> (error out=w605:errorcluster)  [unwired: 1 in, 1 out]
                n492 = property on="Duty-Width" class="Str"(error in=w605, "Visible"=w606) -> (error out=w608:errorcluster)  [unwired: 1 in, 1 out]
                n493 = property on="SymmStr" class="Str"(error in=w608, "Visible"=w606) -> (error out=w607:errorcluster)  [unwired: 1 in, 1 out]
                n494 = property on="RisEdgeStr" class="Str"(error in=w607, "Visible"=w606) -> (error out=w601:errorcluster)  [unwired: 1 in, 1 out]
                n495 = property on="FallEdgeStr" class="Str"(error in=w601, "Visible"=w606) -> (error out=w596:errorcluster)  [unwired: 1 in, 1 out]
                n496 = property on="Freq/Period" class="Bool (strict)"(error in=w596, "Visible"=w597) -> (error out=w600:errorcluster)  [unwired: 1 in, 1 out]
                n497 = property on="Ampl/HighL" class="Bool (strict)"(error in=w600, "Visible"=w597) -> (error out=w599:errorcluster)  [unwired: 1 in, 1 out]
                n498 = property on="Offset/LowL" class="Bool (strict)"(error in=w599, "Visible"=w597) -> (error out=w598:errorcluster)  [unwired: 1 in, 1 out]
                n499 = property on="Duty/Width" class="Bool (strict)"(error in=w598, "Visible"=w597) -> (error out=w595:errorcluster)  [unwired: 1 in, 1 out]
                n500 = property on="Sine" class="Bool (strict)"(error in=w595, "Visible"=w626) -> (error out=w623:errorcluster)  [unwired: 1 in, 1 out]
                n501 = property on="Square" class="Bool (strict)"(error in=w623, "Visible"=w626) -> (error out=w622:errorcluster)  [unwired: 1 in, 1 out]
                n502 = property on="Ramp" class="Bool (strict)"(error in=w622, "Visible"=w626) -> (error out=w621:errorcluster)  [unwired: 1 in, 1 out]
                n503 = property on="Pulse" class="Bool (strict)"(error in=w621, "Visible"=w626) -> (error out=w624:errorcluster)  [unwired: 1 in, 1 out]
                n504 = property on="Noise" class="Bool (strict)"(error in=w624, "Visible"=w626) -> (error out=w625:errorcluster)  [unwired: 1 in, 1 out]
                n505 = property on="DC" class="Bool (strict)"(error in=w625, "Visible"=w626) -> (error out=w609:errorcluster)  [unwired: 1 in, 1 out]
                n506 = property on="Freq" class="DigNum (strict)"(error in=w609, "Visible"=w592) -> (error out=w617:errorcluster)  [unwired: 1 in, 1 out]
                n507 = property on="Period" class="DigNum (strict)"(error in=w617, "Visible"=w592) -> (error out=w616:errorcluster)  [unwired: 1 in, 1 out]
                n508 = property on="Ampl" class="DigNum (strict)"(error in=w616, "Visible"=w592) -> (error out=w615:errorcluster)  [unwired: 1 in, 1 out]
                n509 = property on="HighL" class="DigNum (strict)"(error in=w615, "Visible"=w592) -> (error out=w618:errorcluster)  [unwired: 1 in, 1 out]
                n510 = property on="Offset" class="DigNum (strict)"(error in=w618, "Visible"=w592) -> (error out=w614:errorcluster)  [unwired: 1 in, 1 out]
                n511 = property on="LowL" class="DigNum (strict)"(error in=w614, "Visible"=w592) -> (error out=w613:errorcluster)  [unwired: 1 in, 1 out]
                n512 = property on="PhaseDBL" class="DigNum (strict)"(error in=w613, "Visible"=w592) -> (error out=w619:errorcluster)  [unwired: 1 in, 1 out]
                n513 = property on="Duty" class="DigNum (strict)"(error in=w619, "Visible"=w592) -> (error out=w620:errorcluster)  [unwired: 1 in, 1 out]
                n514 = property on="SymmDBL" class="DigNum (strict)"(error in=w620, "Visible"=w592) -> (error out=w612:errorcluster)  [unwired: 1 in, 1 out]
                n515 = property on="Width" class="DigNum (strict)"(error in=w612, "Visible"=w592) -> (error out=w611:errorcluster)  [unwired: 1 in, 1 out]
                n516 = property on="RisEdgeDBL" class="DigNum (strict)"(error in=w611, "Visible"=w592) -> (error out=w610:errorcluster)  [unwired: 1 in, 1 out]
                n517 = property on="FallEdgeDBL" class="DigNum (strict)"(error in=w610, "Visible"=w592) -> (error out=w593:errorcluster)  [unwired: 1 in, 1 out]
                n518 = property on="OK" class="Bool (strict)"(error in=w593, "Visible"=w592) -> (error out=w591:errorcluster)  [unwired: 1 in, 1 out]
                n519 = property on="Freq-Period" class="Str"(error in=w591, "Visible"=w627) -> (error out=w633:errorcluster)  [unwired: 1 in, 1 out]
                n520 = property on="Freq/Period" class="Bool (strict)"(error in=w591, "Visible"=w627) -> (error out=w630:errorcluster)  [unwired: 1 in, 1 out]
                n521 = property on="Ampl-HighL" class="Str"(error in=w633, "Visible"=w627) -> (error out=w632:errorcluster)  [unwired: 1 in, 1 out]
                n522 = property on="Ampl/HighL" class="Bool (strict)"(error in=w630, "Visible"=w627) -> (error out=w629:errorcluster)  [unwired: 1 in, 1 out]
                n523 = property on="Offset-LowL" class="Str"(error in=w632, "Visible"=w627) -> (error out=w631:errorcluster)  [unwired: 1 in, 1 out]
                n524 = property on="Offset/LowL" class="Bool (strict)"(error in=w629, "Visible"=w627) -> (error out=w628:errorcluster)  [unwired: 1 in, 1 out]
                n525 = property on="PhaseStr" class="Str"(error in=w631, "Visible"=w627) -> ()  [unwired: 1 in, 2 out]
                n526 = property on="Slider" class="Bool (strict)"(error in=w628, "Visible"=w627) -> ()  [unwired: 1 in, 2 out]
              }
              frame True {
                w644 = FALSE ("Visible")
                w653 = FALSE ("Visible")
                w639 = FALSE ("Visible")
                w673 = FALSE ("Visible")
                w634 = TRUE ("Visible")
                # "AllSwapButtonsVisible?"
                # "AllStringsVisible?"
                # "AllValuesVisible?"
                # "AllWaveformsVisible?"
                n527 = property on="Freq-Period" class="Str"(error in=w641, "Visible"=w653) -> (error out=w651:errorcluster)  [unwired: 1 in, 1 out]
                n528 = property on="Ampl-HighL" class="Str"(error in=w651, "Visible"=w653) -> (error out=w650:errorcluster)  [unwired: 1 in, 1 out]
                n529 = property on="Offset-LowL" class="Str"(error in=w650, "Visible"=w653) -> (error out=w649:errorcluster)  [unwired: 1 in, 1 out]
                n530 = property on="PhaseStr" class="Str"(error in=w649, "Visible"=w653) -> (error out=w652:errorcluster)  [unwired: 1 in, 1 out]
                n531 = property on="Duty-Width" class="Str"(error in=w652, "Visible"=w653) -> (error out=w655:errorcluster)  [unwired: 1 in, 1 out]
                n532 = property on="SymmStr" class="Str"(error in=w655, "Visible"=w653) -> (error out=w654:errorcluster)  [unwired: 1 in, 1 out]
                n533 = property on="RisEdgeStr" class="Str"(error in=w654, "Visible"=w653) -> (error out=w648:errorcluster)  [unwired: 1 in, 1 out]
                n534 = property on="FallEdgeStr" class="Str"(error in=w648, "Visible"=w653) -> (error out=w643:errorcluster)  [unwired: 1 in, 1 out]
                n535 = property on="Freq/Period" class="Bool (strict)"(error in=w643, "Visible"=w644) -> (error out=w647:errorcluster)  [unwired: 1 in, 1 out]
                n536 = property on="Ampl/HighL" class="Bool (strict)"(error in=w647, "Visible"=w644) -> (error out=w646:errorcluster)  [unwired: 1 in, 1 out]
                n537 = property on="Offset/LowL" class="Bool (strict)"(error in=w646, "Visible"=w644) -> (error out=w645:errorcluster)  [unwired: 1 in, 1 out]
                n538 = property on="Duty/Width" class="Bool (strict)"(error in=w645, "Visible"=w644) -> (error out=w642:errorcluster)  [unwired: 1 in, 1 out]
                n539 = property on="Sine" class="Bool (strict)"(error in=w642, "Visible"=w673) -> (error out=w670:errorcluster)  [unwired: 1 in, 1 out]
                n540 = property on="Square" class="Bool (strict)"(error in=w670, "Visible"=w673) -> (error out=w669:errorcluster)  [unwired: 1 in, 1 out]
                n541 = property on="Ramp" class="Bool (strict)"(error in=w669, "Visible"=w673) -> (error out=w668:errorcluster)  [unwired: 1 in, 1 out]
                n542 = property on="Pulse" class="Bool (strict)"(error in=w668, "Visible"=w673) -> (error out=w671:errorcluster)  [unwired: 1 in, 1 out]
                n543 = property on="Noise" class="Bool (strict)"(error in=w671, "Visible"=w673) -> (error out=w672:errorcluster)  [unwired: 1 in, 1 out]
                n544 = property on="DC" class="Bool (strict)"(error in=w672, "Visible"=w673) -> (error out=w656:errorcluster)  [unwired: 1 in, 1 out]
                n545 = property on="Freq" class="DigNum (strict)"(error in=w656, "Visible"=w639) -> (error out=w664:errorcluster)  [unwired: 1 in, 1 out]
                n546 = property on="Period" class="DigNum (strict)"(error in=w664, "Visible"=w639) -> (error out=w663:errorcluster)  [unwired: 1 in, 1 out]
                n547 = property on="Ampl" class="DigNum (strict)"(error in=w663, "Visible"=w639) -> (error out=w662:errorcluster)  [unwired: 1 in, 1 out]
                n548 = property on="HighL" class="DigNum (strict)"(error in=w662, "Visible"=w639) -> (error out=w665:errorcluster)  [unwired: 1 in, 1 out]
                n549 = property on="Offset" class="DigNum (strict)"(error in=w665, "Visible"=w639) -> (error out=w661:errorcluster)  [unwired: 1 in, 1 out]
                n550 = property on="LowL" class="DigNum (strict)"(error in=w661, "Visible"=w639) -> (error out=w660:errorcluster)  [unwired: 1 in, 1 out]
                n551 = property on="PhaseDBL" class="DigNum (strict)"(error in=w660, "Visible"=w639) -> (error out=w666:errorcluster)  [unwired: 1 in, 1 out]
                n552 = property on="Duty" class="DigNum (strict)"(error in=w666, "Visible"=w639) -> (error out=w667:errorcluster)  [unwired: 1 in, 1 out]
                n553 = property on="SymmDBL" class="DigNum (strict)"(error in=w667, "Visible"=w639) -> (error out=w659:errorcluster)  [unwired: 1 in, 1 out]
                n554 = property on="Width" class="DigNum (strict)"(error in=w659, "Visible"=w639) -> (error out=w658:errorcluster)  [unwired: 1 in, 1 out]
                n555 = property on="RisEdgeDBL" class="DigNum (strict)"(error in=w658, "Visible"=w639) -> (error out=w657:errorcluster)  [unwired: 1 in, 1 out]
                n556 = property on="FallEdgeDBL" class="DigNum (strict)"(error in=w657, "Visible"=w639) -> (error out=w640:errorcluster)  [unwired: 1 in, 1 out]
                n557 = property on="OK" class="Bool (strict)"(error in=w640, "Visible"=w639) -> (error out=w637:errorcluster)  [unwired: 1 in, 1 out]
                n558 = property on="Duty-Width" class="Str"(error in=w637, "Visible"=w634) -> (error out=w635:errorcluster)  [unwired: 1 in, 1 out]
                n559 = property on="Duty/Width" class="Bool (strict)"(error in=w637, "Visible"=w634) -> (error out=w638:errorcluster)  [unwired: 1 in, 1 out]
                n560 = property on="Slider" class="Bool (strict)"(error in=w638, "Visible"=w634) -> ()  [unwired: 1 in, 2 out]
                n561 = property on="RisEdgeStr" class="Str"(error in=w635, "Visible"=w634) -> (error out=w636:errorcluster)  [unwired: 1 in, 1 out]
                n562 = property on="FallEdgeStr" class="Str"(error in=w636, "Visible"=w634) -> ()  [unwired: 1 in, 2 out]
              }
            }
          }
        }
        n563 = case shown="2, Default" w407 {
          tunnel: [w414 w418 w422] -> w405
          tunnel: w406 -> [w413 w417 w421]
          frame 2, Default {
            n564 = case shown="True" w413 {
              tunnel: ["Home_Square_2.bmp" "Home_Square_1.bmp"] -> w414
              frame True {
              }
              frame False {
              }
            }
          }
          frame 4 {
            n565 = case shown="True" w417 {
              tunnel: ["Home_Ramp_2.bmp" "Home_Ramp_1.bmp"] -> w418
              frame True {
              }
              frame False {
              }
            }
          }
          frame 8 {
            n566 = case shown="False" w421 {
              tunnel: ["Home_Pulse_2.bmp" "Home_Pulse_1.bmp"] -> w422
              frame True {
              }
              frame False {
              }
            }
          }
        }
        n567 = Build Path(base path=w410, name or relative path=w405) -> (appended path=w412:path)
        n568 = call "RDG822 Update Screen.vi"("error in"=w408, "Path to file"=w412) -> ("error out"=w409:errorcluster, "Screen"=w411:picture)  [unwired: 8 in]
        n569 = local write "Screen"(w411) -> ()
        n570 = local write "error out"(w409) -> ()
      }
      event "OK": Mouse Down {
        n571 = event-data() -> ()  [unwired: 1 in, 8 out]
        n572 = local read "MenuCount"() -> (w682:u32)
        n573 = local read "Slider"() -> (w677:bool)
        n574 = call "Time Delay7"("error in (no error)"=w684) -> ("error out"=w683:errorcluster)  [unwired: 10 in]
        n575 = case shown="16" w682 {
          tunnel: w677 -> [_ w742 w831 w920 _ _]
          tunnel: w683 -> [w699 w743 w832 w919 w1009 w1052]
          tunnel: ["Home_Sine.bmp" w744 w829 w918 "Home_Noise.bmp" "Home_DC.bmp"] -> w685
          tunnel: [w698 w741 w830 w917 w1008 w1051] -> w676
          frame 1, Default {
            w702 = FALSE ("Visible")
            w711 = FALSE ("Visible")
            w726 = FALSE ("Visible")
            w732 = FALSE ("Visible")
            w733 = FALSE ("Visible")
            w734 = TRUE ("Visible")
            # "Sine"
            # "AllSwapButtonsVisible?"
            # "AllStringsVisible?"
            # "AllValuesVisible?"
            # "AllWaveformsVisible?"
            n576 = property on="Freq-Period" class="Str"(error in=w699, "Visible"=w711) -> (error out=w709:errorcluster)  [unwired: 1 in, 1 out]
            n577 = property on="Ampl-HighL" class="Str"(error in=w709, "Visible"=w711) -> (error out=w708:errorcluster)  [unwired: 1 in, 1 out]
            n578 = property on="Offset-LowL" class="Str"(error in=w708, "Visible"=w711) -> (error out=w707:errorcluster)  [unwired: 1 in, 1 out]
            n579 = property on="PhaseStr" class="Str"(error in=w707, "Visible"=w711) -> (error out=w710:errorcluster)  [unwired: 1 in, 1 out]
            n580 = property on="Duty-Width" class="Str"(error in=w710, "Visible"=w711) -> (error out=w713:errorcluster)  [unwired: 1 in, 1 out]
            n581 = property on="SymmStr" class="Str"(error in=w713, "Visible"=w711) -> (error out=w712:errorcluster)  [unwired: 1 in, 1 out]
            n582 = property on="RisEdgeStr" class="Str"(error in=w712, "Visible"=w711) -> (error out=w706:errorcluster)  [unwired: 1 in, 1 out]
            n583 = property on="FallEdgeStr" class="Str"(error in=w706, "Visible"=w711) -> (error out=w701:errorcluster)  [unwired: 1 in, 1 out]
            n584 = property on="Slider" class="Bool (strict)"(error in=w699, "Visible"=w733) -> ()  [unwired: 1 in, 2 out]
            n585 = property on="OK" class="Bool (strict)"("Visible"=w733) -> ()  [unwired: 2 in, 2 out]
            n586 = property on="Freq/Period" class="Bool (strict)"(error in=w701, "Visible"=w702) -> (error out=w705:errorcluster)  [unwired: 1 in, 1 out]
            n587 = property on="Ampl/HighL" class="Bool (strict)"(error in=w705, "Visible"=w702) -> (error out=w704:errorcluster)  [unwired: 1 in, 1 out]
            n588 = property on="Offset/LowL" class="Bool (strict)"(error in=w704, "Visible"=w702) -> (error out=w703:errorcluster)  [unwired: 1 in, 1 out]
            n589 = property on="Duty/Width" class="Bool (strict)"(error in=w703, "Visible"=w702) -> (error out=w700:errorcluster)  [unwired: 1 in, 1 out]
            n590 = property on="Sine" class="Bool (strict)"(error in=w700, "Visible"=w732) -> (error out=w729:errorcluster)  [unwired: 1 in, 1 out]
            n591 = property on="Square" class="Bool (strict)"(error in=w729, "Visible"=w732) -> (error out=w728:errorcluster)  [unwired: 1 in, 1 out]
            n592 = property on="Ramp" class="Bool (strict)"(error in=w728, "Visible"=w732) -> (error out=w727:errorcluster)  [unwired: 1 in, 1 out]
            n593 = property on="Pulse" class="Bool (strict)"(error in=w727, "Visible"=w732) -> (error out=w730:errorcluster)  [unwired: 1 in, 1 out]
            n594 = property on="Noise" class="Bool (strict)"(error in=w730, "Visible"=w732) -> (error out=w731:errorcluster)  [unwired: 1 in, 1 out]
            n595 = property on="DC" class="Bool (strict)"(error in=w731, "Visible"=w732) -> (error out=w714:errorcluster)  [unwired: 1 in, 1 out]
            n596 = property on="Freq" class="DigNum (strict)"(error in=w714, "Visible"=w726) -> (error out=w722:errorcluster)  [unwired: 1 in, 1 out]
            n597 = property on="Period" class="DigNum (strict)"(error in=w722, "Visible"=w726) -> (error out=w721:errorcluster)  [unwired: 1 in, 1 out]
            n598 = property on="Ampl" class="DigNum (strict)"(error in=w721, "Visible"=w726) -> (error out=w720:errorcluster)  [unwired: 1 in, 1 out]
            n599 = property on="HighL" class="DigNum (strict)"(error in=w720, "Visible"=w726) -> (error out=w723:errorcluster)  [unwired: 1 in, 1 out]
            n600 = property on="Offset" class="DigNum (strict)"(error in=w723, "Visible"=w726) -> (error out=w719:errorcluster)  [unwired: 1 in, 1 out]
            n601 = property on="LowL" class="DigNum (strict)"(error in=w719, "Visible"=w726) -> (error out=w718:errorcluster)  [unwired: 1 in, 1 out]
            n602 = property on="PhaseDBL" class="DigNum (strict)"(error in=w718, "Visible"=w726) -> (error out=w724:errorcluster)  [unwired: 1 in, 1 out]
            n603 = property on="Duty" class="DigNum (strict)"(error in=w724, "Visible"=w726) -> (error out=w725:errorcluster)  [unwired: 1 in, 1 out]
            n604 = property on="SymmDBL" class="DigNum (strict)"(error in=w725, "Visible"=w726) -> (error out=w717:errorcluster)  [unwired: 1 in, 1 out]
            n605 = property on="Width" class="DigNum (strict)"(error in=w717, "Visible"=w726) -> (error out=w716:errorcluster)  [unwired: 1 in, 1 out]
            n606 = property on="RisEdgeDBL" class="DigNum (strict)"(error in=w716, "Visible"=w726) -> (error out=w715:errorcluster)  [unwired: 1 in, 1 out]
            n607 = property on="FallEdgeDBL" class="DigNum (strict)"(error in=w715, "Visible"=w726) -> (error out=w697:errorcluster)  [unwired: 1 in, 1 out]
            n608 = property on="Freq-Period" class="Str"(error in=w697, "Visible"=w734) -> (error out=w739:errorcluster)  [unwired: 1 in, 1 out]
            n609 = property on="Freq/Period" class="Bool (strict)"(error in=w697, "Visible"=w734) -> (error out=w736:errorcluster)  [unwired: 1 in, 1 out]
            n610 = property on="Ampl-HighL" class="Str"(error in=w739, "Visible"=w734) -> (error out=w738:errorcluster)  [unwired: 1 in, 1 out]
            n611 = property on="Ampl/HighL" class="Bool (strict)"(error in=w736, "Visible"=w734) -> (error out=w735:errorcluster)  [unwired: 1 in, 1 out]
            n612 = property on="Offset-LowL" class="Str"(error in=w738, "Visible"=w734) -> (error out=w737:errorcluster)  [unwired: 1 in, 1 out]
            n613 = property on="Offset/LowL" class="Bool (strict)"(error in=w735, "Visible"=w734) -> ()  [unwired: 1 in, 2 out]
            n614 = property on="PhaseStr" class="Str"(error in=w737, "Visible"=w734) -> (error out=w698:errorcluster)  [unwired: 1 in, 1 out]
          }
          frame 2 {
            # "Square"
            n615 = case shown="True" w742 {
              tunnel: w743 -> [w750 w796]
              tunnel: ["Home_Square_1.bmp" "Home_Square_2.bmp"] -> w744
              tunnel: [w745 w790] -> w741
              frame False {
                w753 = FALSE ("Visible")
                w762 = FALSE ("Visible")
                w748 = FALSE ("Visible")
                w782 = FALSE ("Visible")
                w783 = TRUE ("Visible")
                # "AllSwapButtonsVisible?"
                # "AllStringsVisible?"
                # "AllValuesVisible?"
                # "AllWaveformsVisible?"
                n616 = property on="Freq-Period" class="Str"(error in=w750, "Visible"=w762) -> (error out=w760:errorcluster)  [unwired: 1 in, 1 out]
                n617 = property on="Ampl-HighL" class="Str"(error in=w760, "Visible"=w762) -> (error out=w759:errorcluster)  [unwired: 1 in, 1 out]
                n618 = property on="Offset-LowL" class="Str"(error in=w759, "Visible"=w762) -> (error out=w758:errorcluster)  [unwired: 1 in, 1 out]
                n619 = property on="PhaseStr" class="Str"(error in=w758, "Visible"=w762) -> (error out=w761:errorcluster)  [unwired: 1 in, 1 out]
                n620 = property on="Duty-Width" class="Str"(error in=w761, "Visible"=w762) -> (error out=w764:errorcluster)  [unwired: 1 in, 1 out]
                n621 = property on="SymmStr" class="Str"(error in=w764, "Visible"=w762) -> (error out=w763:errorcluster)  [unwired: 1 in, 1 out]
                n622 = property on="RisEdgeStr" class="Str"(error in=w763, "Visible"=w762) -> (error out=w757:errorcluster)  [unwired: 1 in, 1 out]
                n623 = property on="FallEdgeStr" class="Str"(error in=w757, "Visible"=w762) -> (error out=w752:errorcluster)  [unwired: 1 in, 1 out]
                n624 = property on="Freq/Period" class="Bool (strict)"(error in=w752, "Visible"=w753) -> (error out=w756:errorcluster)  [unwired: 1 in, 1 out]
                n625 = property on="Ampl/HighL" class="Bool (strict)"(error in=w756, "Visible"=w753) -> (error out=w755:errorcluster)  [unwired: 1 in, 1 out]
                n626 = property on="Offset/LowL" class="Bool (strict)"(error in=w755, "Visible"=w753) -> (error out=w754:errorcluster)  [unwired: 1 in, 1 out]
                n627 = property on="Duty/Width" class="Bool (strict)"(error in=w754, "Visible"=w753) -> (error out=w751:errorcluster)  [unwired: 1 in, 1 out]
                n628 = property on="Sine" class="Bool (strict)"(error in=w751, "Visible"=w782) -> (error out=w779:errorcluster)  [unwired: 1 in, 1 out]
                n629 = property on="Square" class="Bool (strict)"(error in=w779, "Visible"=w782) -> (error out=w778:errorcluster)  [unwired: 1 in, 1 out]
                n630 = property on="Ramp" class="Bool (strict)"(error in=w778, "Visible"=w782) -> (error out=w777:errorcluster)  [unwired: 1 in, 1 out]
                n631 = property on="Pulse" class="Bool (strict)"(error in=w777, "Visible"=w782) -> (error out=w780:errorcluster)  [unwired: 1 in, 1 out]
                n632 = property on="Noise" class="Bool (strict)"(error in=w780, "Visible"=w782) -> (error out=w781:errorcluster)  [unwired: 1 in, 1 out]
                n633 = property on="DC" class="Bool (strict)"(error in=w781, "Visible"=w782) -> (error out=w765:errorcluster)  [unwired: 1 in, 1 out]
                n634 = property on="Freq" class="DigNum (strict)"(error in=w765, "Visible"=w748) -> (error out=w773:errorcluster)  [unwired: 1 in, 1 out]
                n635 = property on="Period" class="DigNum (strict)"(error in=w773, "Visible"=w748) -> (error out=w772:errorcluster)  [unwired: 1 in, 1 out]
                n636 = property on="Ampl" class="DigNum (strict)"(error in=w772, "Visible"=w748) -> (error out=w771:errorcluster)  [unwired: 1 in, 1 out]
                n637 = property on="HighL" class="DigNum (strict)"(error in=w771, "Visible"=w748) -> (error out=w774:errorcluster)  [unwired: 1 in, 1 out]
                n638 = property on="Offset" class="DigNum (strict)"(error in=w774, "Visible"=w748) -> (error out=w770:errorcluster)  [unwired: 1 in, 1 out]
                n639 = property on="LowL" class="DigNum (strict)"(error in=w770, "Visible"=w748) -> (error out=w769:errorcluster)  [unwired: 1 in, 1 out]
                n640 = property on="PhaseDBL" class="DigNum (strict)"(error in=w769, "Visible"=w748) -> (error out=w775:errorcluster)  [unwired: 1 in, 1 out]
                n641 = property on="Duty" class="DigNum (strict)"(error in=w775, "Visible"=w748) -> (error out=w776:errorcluster)  [unwired: 1 in, 1 out]
                n642 = property on="SymmDBL" class="DigNum (strict)"(error in=w776, "Visible"=w748) -> (error out=w768:errorcluster)  [unwired: 1 in, 1 out]
                n643 = property on="Width" class="DigNum (strict)"(error in=w768, "Visible"=w748) -> (error out=w767:errorcluster)  [unwired: 1 in, 1 out]
                n644 = property on="RisEdgeDBL" class="DigNum (strict)"(error in=w767, "Visible"=w748) -> (error out=w766:errorcluster)  [unwired: 1 in, 1 out]
                n645 = property on="FallEdgeDBL" class="DigNum (strict)"(error in=w766, "Visible"=w748) -> (error out=w749:errorcluster)  [unwired: 1 in, 1 out]
                n646 = property on="OK" class="Bool (strict)"(error in=w749, "Visible"=w748) -> (error out=w747:errorcluster)  [unwired: 1 in, 1 out]
                n647 = property on="Freq-Period" class="Str"(error in=w747, "Visible"=w783) -> (error out=w789:errorcluster)  [unwired: 1 in, 1 out]
                n648 = property on="Freq/Period" class="Bool (strict)"(error in=w747, "Visible"=w783) -> (error out=w786:errorcluster)  [unwired: 1 in, 1 out]
                n649 = property on="Ampl-HighL" class="Str"(error in=w789, "Visible"=w783) -> (error out=w788:errorcluster)  [unwired: 1 in, 1 out]
                n650 = property on="Ampl/HighL" class="Bool (strict)"(error in=w786, "Visible"=w783) -> (error out=w785:errorcluster)  [unwired: 1 in, 1 out]
                n651 = property on="Offset-LowL" class="Str"(error in=w788, "Visible"=w783) -> (error out=w787:errorcluster)  [unwired: 1 in, 1 out]
                n652 = property on="Offset/LowL" class="Bool (strict)"(error in=w785, "Visible"=w783) -> (error out=w784:errorcluster)  [unwired: 1 in, 1 out]
                n653 = property on="PhaseStr" class="Str"(error in=w787, "Visible"=w783) -> (error out=w745:errorcluster)  [unwired: 1 in, 1 out]
                n654 = property on="Slider" class="Bool (strict)"(error in=w784, "Visible"=w783) -> ()  [unwired: 1 in, 2 out]
              }
              frame True {
                w799 = FALSE ("Visible")
                w808 = FALSE ("Visible")
                w794 = FALSE ("Visible")
                w828 = FALSE ("Visible")
                w793 = TRUE ("Visible")
                # "AllSwapButtonsVisible?"
                # "AllStringsVisible?"
                # "AllValuesVisible?"
                # "AllWaveformsVisible?"
                n655 = property on="Freq-Period" class="Str"(error in=w796, "Visible"=w808) -> (error out=w806:errorcluster)  [unwired: 1 in, 1 out]
                n656 = property on="Ampl-HighL" class="Str"(error in=w806, "Visible"=w808) -> (error out=w805:errorcluster)  [unwired: 1 in, 1 out]
                n657 = property on="Offset-LowL" class="Str"(error in=w805, "Visible"=w808) -> (error out=w804:errorcluster)  [unwired: 1 in, 1 out]
                n658 = property on="PhaseStr" class="Str"(error in=w804, "Visible"=w808) -> (error out=w807:errorcluster)  [unwired: 1 in, 1 out]
                n659 = property on="Duty-Width" class="Str"(error in=w807, "Visible"=w808) -> (error out=w810:errorcluster)  [unwired: 1 in, 1 out]
                n660 = property on="SymmStr" class="Str"(error in=w810, "Visible"=w808) -> (error out=w809:errorcluster)  [unwired: 1 in, 1 out]
                n661 = property on="RisEdgeStr" class="Str"(error in=w809, "Visible"=w808) -> (error out=w803:errorcluster)  [unwired: 1 in, 1 out]
                n662 = property on="FallEdgeStr" class="Str"(error in=w803, "Visible"=w808) -> (error out=w798:errorcluster)  [unwired: 1 in, 1 out]
                n663 = property on="Freq/Period" class="Bool (strict)"(error in=w798, "Visible"=w799) -> (error out=w802:errorcluster)  [unwired: 1 in, 1 out]
                n664 = property on="Ampl/HighL" class="Bool (strict)"(error in=w802, "Visible"=w799) -> (error out=w801:errorcluster)  [unwired: 1 in, 1 out]
                n665 = property on="Offset/LowL" class="Bool (strict)"(error in=w801, "Visible"=w799) -> (error out=w800:errorcluster)  [unwired: 1 in, 1 out]
                n666 = property on="Duty/Width" class="Bool (strict)"(error in=w800, "Visible"=w799) -> (error out=w797:errorcluster)  [unwired: 1 in, 1 out]
                n667 = property on="Sine" class="Bool (strict)"(error in=w797, "Visible"=w828) -> (error out=w825:errorcluster)  [unwired: 1 in, 1 out]
                n668 = property on="Square" class="Bool (strict)"(error in=w825, "Visible"=w828) -> (error out=w824:errorcluster)  [unwired: 1 in, 1 out]
                n669 = property on="Ramp" class="Bool (strict)"(error in=w824, "Visible"=w828) -> (error out=w823:errorcluster)  [unwired: 1 in, 1 out]
                n670 = property on="Pulse" class="Bool (strict)"(error in=w823, "Visible"=w828) -> (error out=w826:errorcluster)  [unwired: 1 in, 1 out]
                n671 = property on="Noise" class="Bool (strict)"(error in=w826, "Visible"=w828) -> (error out=w827:errorcluster)  [unwired: 1 in, 1 out]
                n672 = property on="DC" class="Bool (strict)"(error in=w827, "Visible"=w828) -> (error out=w811:errorcluster)  [unwired: 1 in, 1 out]
                n673 = property on="Freq" class="DigNum (strict)"(error in=w811, "Visible"=w794) -> (error out=w819:errorcluster)  [unwired: 1 in, 1 out]
                n674 = property on="Period" class="DigNum (strict)"(error in=w819, "Visible"=w794) -> (error out=w818:errorcluster)  [unwired: 1 in, 1 out]
                n675 = property on="Ampl" class="DigNum (strict)"(error in=w818, "Visible"=w794) -> (error out=w817:errorcluster)  [unwired: 1 in, 1 out]
                n676 = property on="HighL" class="DigNum (strict)"(error in=w817, "Visible"=w794) -> (error out=w820:errorcluster)  [unwired: 1 in, 1 out]
                n677 = property on="Offset" class="DigNum (strict)"(error in=w820, "Visible"=w794) -> (error out=w816:errorcluster)  [unwired: 1 in, 1 out]
                n678 = property on="LowL" class="DigNum (strict)"(error in=w816, "Visible"=w794) -> (error out=w815:errorcluster)  [unwired: 1 in, 1 out]
                n679 = property on="PhaseDBL" class="DigNum (strict)"(error in=w815, "Visible"=w794) -> (error out=w821:errorcluster)  [unwired: 1 in, 1 out]
                n680 = property on="Duty" class="DigNum (strict)"(error in=w821, "Visible"=w794) -> (error out=w822:errorcluster)  [unwired: 1 in, 1 out]
                n681 = property on="SymmDBL" class="DigNum (strict)"(error in=w822, "Visible"=w794) -> (error out=w814:errorcluster)  [unwired: 1 in, 1 out]
                n682 = property on="Width" class="DigNum (strict)"(error in=w814, "Visible"=w794) -> (error out=w813:errorcluster)  [unwired: 1 in, 1 out]
                n683 = property on="RisEdgeDBL" class="DigNum (strict)"(error in=w813, "Visible"=w794) -> (error out=w812:errorcluster)  [unwired: 1 in, 1 out]
                n684 = property on="FallEdgeDBL" class="DigNum (strict)"(error in=w812, "Visible"=w794) -> (error out=w795:errorcluster)  [unwired: 1 in, 1 out]
                n685 = property on="OK" class="Bool (strict)"(error in=w795, "Visible"=w794) -> (error out=w792:errorcluster)  [unwired: 1 in, 1 out]
                n686 = property on="Duty-Width" class="Str"(error in=w792, "Visible"=w793) -> (error out=w790:errorcluster)  [unwired: 1 in, 1 out]
                n687 = property on="Slider" class="Bool (strict)"(error in=w792, "Visible"=w793) -> ()  [unwired: 1 in, 2 out]
              }
            }
          }
          frame 4 {
            # "Ramp"
            n688 = case shown="False" w831 {
              tunnel: w832 -> [w838 w884]
              tunnel: ["Home_Ramp_1.bmp" "Home_Ramp_2.bmp"] -> w829
              tunnel: [w833 w878] -> w830
              frame False {
                w841 = FALSE ("Visible")
                w850 = FALSE ("Visible")
                w836 = FALSE ("Visible")
                w870 = FALSE ("Visible")
                w871 = TRUE ("Visible")
                # "AllSwapButtonsVisible?"
                # "AllStringsVisible?"
                # "AllValuesVisible?"
                # "AllWaveformsVisible?"
                n689 = property on="Freq-Period" class="Str"(error in=w838, "Visible"=w850) -> (error out=w848:errorcluster)  [unwired: 1 in, 1 out]
                n690 = property on="Ampl-HighL" class="Str"(error in=w848, "Visible"=w850) -> (error out=w847:errorcluster)  [unwired: 1 in, 1 out]
                n691 = property on="Offset-LowL" class="Str"(error in=w847, "Visible"=w850) -> (error out=w846:errorcluster)  [unwired: 1 in, 1 out]
                n692 = property on="PhaseStr" class="Str"(error in=w846, "Visible"=w850) -> (error out=w849:errorcluster)  [unwired: 1 in, 1 out]
                n693 = property on="Duty-Width" class="Str"(error in=w849, "Visible"=w850) -> (error out=w852:errorcluster)  [unwired: 1 in, 1 out]
                n694 = property on="SymmStr" class="Str"(error in=w852, "Visible"=w850) -> (error out=w851:errorcluster)  [unwired: 1 in, 1 out]
                n695 = property on="RisEdgeStr" class="Str"(error in=w851, "Visible"=w850) -> (error out=w845:errorcluster)  [unwired: 1 in, 1 out]
                n696 = property on="FallEdgeStr" class="Str"(error in=w845, "Visible"=w850) -> (error out=w840:errorcluster)  [unwired: 1 in, 1 out]
                n697 = property on="Freq/Period" class="Bool (strict)"(error in=w840, "Visible"=w841) -> (error out=w844:errorcluster)  [unwired: 1 in, 1 out]
                n698 = property on="Ampl/HighL" class="Bool (strict)"(error in=w844, "Visible"=w841) -> (error out=w843:errorcluster)  [unwired: 1 in, 1 out]
                n699 = property on="Offset/LowL" class="Bool (strict)"(error in=w843, "Visible"=w841) -> (error out=w842:errorcluster)  [unwired: 1 in, 1 out]
                n700 = property on="Duty/Width" class="Bool (strict)"(error in=w842, "Visible"=w841) -> (error out=w839:errorcluster)  [unwired: 1 in, 1 out]
                n701 = property on="Sine" class="Bool (strict)"(error in=w839, "Visible"=w870) -> (error out=w867:errorcluster)  [unwired: 1 in, 1 out]
                n702 = property on="Square" class="Bool (strict)"(error in=w867, "Visible"=w870) -> (error out=w866:errorcluster)  [unwired: 1 in, 1 out]
                n703 = property on="Ramp" class="Bool (strict)"(error in=w866, "Visible"=w870) -> (error out=w865:errorcluster)  [unwired: 1 in, 1 out]
                n704 = property on="Pulse" class="Bool (strict)"(error in=w865, "Visible"=w870) -> (error out=w868:errorcluster)  [unwired: 1 in, 1 out]
                n705 = property on="Noise" class="Bool (strict)"(error in=w868, "Visible"=w870) -> (error out=w869:errorcluster)  [unwired: 1 in, 1 out]
                n706 = property on="DC" class="Bool (strict)"(error in=w869, "Visible"=w870) -> (error out=w853:errorcluster)  [unwired: 1 in, 1 out]
                n707 = property on="Freq" class="DigNum (strict)"(error in=w853, "Visible"=w836) -> (error out=w861:errorcluster)  [unwired: 1 in, 1 out]
                n708 = property on="Period" class="DigNum (strict)"(error in=w861, "Visible"=w836) -> (error out=w860:errorcluster)  [unwired: 1 in, 1 out]
                n709 = property on="Ampl" class="DigNum (strict)"(error in=w860, "Visible"=w836) -> (error out=w859:errorcluster)  [unwired: 1 in, 1 out]
                n710 = property on="HighL" class="DigNum (strict)"(error in=w859, "Visible"=w836) -> (error out=w862:errorcluster)  [unwired: 1 in, 1 out]
                n711 = property on="Offset" class="DigNum (strict)"(error in=w862, "Visible"=w836) -> (error out=w858:errorcluster)  [unwired: 1 in, 1 out]
                n712 = property on="LowL" class="DigNum (strict)"(error in=w858, "Visible"=w836) -> (error out=w857:errorcluster)  [unwired: 1 in, 1 out]
                n713 = property on="PhaseDBL" class="DigNum (strict)"(error in=w857, "Visible"=w836) -> (error out=w863:errorcluster)  [unwired: 1 in, 1 out]
                n714 = property on="Duty" class="DigNum (strict)"(error in=w863, "Visible"=w836) -> (error out=w864:errorcluster)  [unwired: 1 in, 1 out]
                n715 = property on="SymmDBL" class="DigNum (strict)"(error in=w864, "Visible"=w836) -> (error out=w856:errorcluster)  [unwired: 1 in, 1 out]
                n716 = property on="Width" class="DigNum (strict)"(error in=w856, "Visible"=w836) -> (error out=w855:errorcluster)  [unwired: 1 in, 1 out]
                n717 = property on="RisEdgeDBL" class="DigNum (strict)"(error in=w855, "Visible"=w836) -> (error out=w854:errorcluster)  [unwired: 1 in, 1 out]
                n718 = property on="FallEdgeDBL" class="DigNum (strict)"(error in=w854, "Visible"=w836) -> (error out=w837:errorcluster)  [unwired: 1 in, 1 out]
                n719 = property on="OK" class="Bool (strict)"(error in=w837, "Visible"=w836) -> (error out=w835:errorcluster)  [unwired: 1 in, 1 out]
                n720 = property on="Freq-Period" class="Str"(error in=w835, "Visible"=w871) -> (error out=w877:errorcluster)  [unwired: 1 in, 1 out]
                n721 = property on="Freq/Period" class="Bool (strict)"(error in=w835, "Visible"=w871) -> (error out=w874:errorcluster)  [unwired: 1 in, 1 out]
                n722 = property on="Ampl-HighL" class="Str"(error in=w877, "Visible"=w871) -> (error out=w876:errorcluster)  [unwired: 1 in, 1 out]
                n723 = property on="Ampl/HighL" class="Bool (strict)"(error in=w874, "Visible"=w871) -> (error out=w873:errorcluster)  [unwired: 1 in, 1 out]
                n724 = property on="Offset-LowL" class="Str"(error in=w876, "Visible"=w871) -> (error out=w875:errorcluster)  [unwired: 1 in, 1 out]
                n725 = property on="Offset/LowL" class="Bool (strict)"(error in=w873, "Visible"=w871) -> (error out=w872:errorcluster)  [unwired: 1 in, 1 out]
                n726 = property on="PhaseStr" class="Str"(error in=w875, "Visible"=w871) -> (error out=w833:errorcluster)  [unwired: 1 in, 1 out]
                n727 = property on="Slider" class="Bool (strict)"(error in=w872, "Visible"=w871) -> ()  [unwired: 1 in, 2 out]
              }
              frame True {
                w887 = FALSE ("Visible")
                w896 = FALSE ("Visible")
                w882 = FALSE ("Visible")
                w916 = FALSE ("Visible")
                w881 = TRUE ("Visible")
                # "AllSwapButtonsVisible?"
                # "AllStringsVisible?"
                # "AllValuesVisible?"
                # "AllWaveformsVisible?"
                n728 = property on="Freq-Period" class="Str"(error in=w884, "Visible"=w896) -> (error out=w894:errorcluster)  [unwired: 1 in, 1 out]
                n729 = property on="Ampl-HighL" class="Str"(error in=w894, "Visible"=w896) -> (error out=w893:errorcluster)  [unwired: 1 in, 1 out]
                n730 = property on="Offset-LowL" class="Str"(error in=w893, "Visible"=w896) -> (error out=w892:errorcluster)  [unwired: 1 in, 1 out]
                n731 = property on="PhaseStr" class="Str"(error in=w892, "Visible"=w896) -> (error out=w895:errorcluster)  [unwired: 1 in, 1 out]
                n732 = property on="Duty-Width" class="Str"(error in=w895, "Visible"=w896) -> (error out=w898:errorcluster)  [unwired: 1 in, 1 out]
                n733 = property on="SymmStr" class="Str"(error in=w898, "Visible"=w896) -> (error out=w897:errorcluster)  [unwired: 1 in, 1 out]
                n734 = property on="RisEdgeStr" class="Str"(error in=w897, "Visible"=w896) -> (error out=w891:errorcluster)  [unwired: 1 in, 1 out]
                n735 = property on="FallEdgeStr" class="Str"(error in=w891, "Visible"=w896) -> (error out=w886:errorcluster)  [unwired: 1 in, 1 out]
                n736 = property on="Freq/Period" class="Bool (strict)"(error in=w886, "Visible"=w887) -> (error out=w890:errorcluster)  [unwired: 1 in, 1 out]
                n737 = property on="Ampl/HighL" class="Bool (strict)"(error in=w890, "Visible"=w887) -> (error out=w889:errorcluster)  [unwired: 1 in, 1 out]
                n738 = property on="Offset/LowL" class="Bool (strict)"(error in=w889, "Visible"=w887) -> (error out=w888:errorcluster)  [unwired: 1 in, 1 out]
                n739 = property on="Duty/Width" class="Bool (strict)"(error in=w888, "Visible"=w887) -> (error out=w885:errorcluster)  [unwired: 1 in, 1 out]
                n740 = property on="Sine" class="Bool (strict)"(error in=w885, "Visible"=w916) -> (error out=w913:errorcluster)  [unwired: 1 in, 1 out]
                n741 = property on="Square" class="Bool (strict)"(error in=w913, "Visible"=w916) -> (error out=w912:errorcluster)  [unwired: 1 in, 1 out]
                n742 = property on="Ramp" class="Bool (strict)"(error in=w912, "Visible"=w916) -> (error out=w911:errorcluster)  [unwired: 1 in, 1 out]
                n743 = property on="Pulse" class="Bool (strict)"(error in=w911, "Visible"=w916) -> (error out=w914:errorcluster)  [unwired: 1 in, 1 out]
                n744 = property on="Noise" class="Bool (strict)"(error in=w914, "Visible"=w916) -> (error out=w915:errorcluster)  [unwired: 1 in, 1 out]
                n745 = property on="DC" class="Bool (strict)"(error in=w915, "Visible"=w916) -> (error out=w899:errorcluster)  [unwired: 1 in, 1 out]
                n746 = property on="Freq" class="DigNum (strict)"(error in=w899, "Visible"=w882) -> (error out=w907:errorcluster)  [unwired: 1 in, 1 out]
                n747 = property on="Period" class="DigNum (strict)"(error in=w907, "Visible"=w882) -> (error out=w906:errorcluster)  [unwired: 1 in, 1 out]
                n748 = property on="Ampl" class="DigNum (strict)"(error in=w906, "Visible"=w882) -> (error out=w905:errorcluster)  [unwired: 1 in, 1 out]
                n749 = property on="HighL" class="DigNum (strict)"(error in=w905, "Visible"=w882) -> (error out=w908:errorcluster)  [unwired: 1 in, 1 out]
                n750 = property on="Offset" class="DigNum (strict)"(error in=w908, "Visible"=w882) -> (error out=w904:errorcluster)  [unwired: 1 in, 1 out]
                n751 = property on="LowL" class="DigNum (strict)"(error in=w904, "Visible"=w882) -> (error out=w903:errorcluster)  [unwired: 1 in, 1 out]
                n752 = property on="PhaseDBL" class="DigNum (strict)"(error in=w903, "Visible"=w882) -> (error out=w909:errorcluster)  [unwired: 1 in, 1 out]
                n753 = property on="Duty" class="DigNum (strict)"(error in=w909, "Visible"=w882) -> (error out=w910:errorcluster)  [unwired: 1 in, 1 out]
                n754 = property on="SymmDBL" class="DigNum (strict)"(error in=w910, "Visible"=w882) -> (error out=w902:errorcluster)  [unwired: 1 in, 1 out]
                n755 = property on="Width" class="DigNum (strict)"(error in=w902, "Visible"=w882) -> (error out=w901:errorcluster)  [unwired: 1 in, 1 out]
                n756 = property on="RisEdgeDBL" class="DigNum (strict)"(error in=w901, "Visible"=w882) -> (error out=w900:errorcluster)  [unwired: 1 in, 1 out]
                n757 = property on="FallEdgeDBL" class="DigNum (strict)"(error in=w900, "Visible"=w882) -> (error out=w883:errorcluster)  [unwired: 1 in, 1 out]
                n758 = property on="OK" class="Bool (strict)"(error in=w883, "Visible"=w882) -> (error out=w880:errorcluster)  [unwired: 1 in, 1 out]
                n759 = property on="SymmStr" class="Str"(error in=w880, "Visible"=w881) -> (error out=w878:errorcluster)  [unwired: 1 in, 1 out]
                n760 = property on="Slider" class="Bool (strict)"(error in=w880, "Visible"=w881) -> ()  [unwired: 1 in, 2 out]
              }
            }
          }
          frame 8 {
            # "Pulse"
            n761 = case shown="False" w920 {
              tunnel: w919 -> [w926 w975]
              tunnel: ["Home_Pulse_1.bmp" "Home_Pulse_2.bmp"] -> w918
              tunnel: [w921 w966] -> w917
              frame False {
                w929 = FALSE ("Visible")
                w938 = FALSE ("Visible")
                w924 = FALSE ("Visible")
                w958 = FALSE ("Visible")
                w959 = TRUE ("Visible")
                # "AllSwapButtonsVisible?"
                # "AllStringsVisible?"
                # "AllValuesVisible?"
                # "AllWaveformsVisible?"
                n762 = property on="Freq-Period" class="Str"(error in=w926, "Visible"=w938) -> (error out=w936:errorcluster)  [unwired: 1 in, 1 out]
                n763 = property on="Ampl-HighL" class="Str"(error in=w936, "Visible"=w938) -> (error out=w935:errorcluster)  [unwired: 1 in, 1 out]
                n764 = property on="Offset-LowL" class="Str"(error in=w935, "Visible"=w938) -> (error out=w934:errorcluster)  [unwired: 1 in, 1 out]
                n765 = property on="PhaseStr" class="Str"(error in=w934, "Visible"=w938) -> (error out=w937:errorcluster)  [unwired: 1 in, 1 out]
                n766 = property on="Duty-Width" class="Str"(error in=w937, "Visible"=w938) -> (error out=w940:errorcluster)  [unwired: 1 in, 1 out]
                n767 = property on="SymmStr" class="Str"(error in=w940, "Visible"=w938) -> (error out=w939:errorcluster)  [unwired: 1 in, 1 out]
                n768 = property on="RisEdgeStr" class="Str"(error in=w939, "Visible"=w938) -> (error out=w933:errorcluster)  [unwired: 1 in, 1 out]
                n769 = property on="FallEdgeStr" class="Str"(error in=w933, "Visible"=w938) -> (error out=w928:errorcluster)  [unwired: 1 in, 1 out]
                n770 = property on="Freq/Period" class="Bool (strict)"(error in=w928, "Visible"=w929) -> (error out=w932:errorcluster)  [unwired: 1 in, 1 out]
                n771 = property on="Ampl/HighL" class="Bool (strict)"(error in=w932, "Visible"=w929) -> (error out=w931:errorcluster)  [unwired: 1 in, 1 out]
                n772 = property on="Offset/LowL" class="Bool (strict)"(error in=w931, "Visible"=w929) -> (error out=w930:errorcluster)  [unwired: 1 in, 1 out]
                n773 = property on="Duty/Width" class="Bool (strict)"(error in=w930, "Visible"=w929) -> (error out=w927:errorcluster)  [unwired: 1 in, 1 out]
                n774 = property on="Sine" class="Bool (strict)"(error in=w927, "Visible"=w958) -> (error out=w955:errorcluster)  [unwired: 1 in, 1 out]
                n775 = property on="Square" class="Bool (strict)"(error in=w955, "Visible"=w958) -> (error out=w954:errorcluster)  [unwired: 1 in, 1 out]
                n776 = property on="Ramp" class="Bool (strict)"(error in=w954, "Visible"=w958) -> (error out=w953:errorcluster)  [unwired: 1 in, 1 out]
                n777 = property on="Pulse" class="Bool (strict)"(error in=w953, "Visible"=w958) -> (error out=w956:errorcluster)  [unwired: 1 in, 1 out]
                n778 = property on="Noise" class="Bool (strict)"(error in=w956, "Visible"=w958) -> (error out=w957:errorcluster)  [unwired: 1 in, 1 out]
                n779 = property on="DC" class="Bool (strict)"(error in=w957, "Visible"=w958) -> (error out=w941:errorcluster)  [unwired: 1 in, 1 out]
                n780 = property on="Freq" class="DigNum (strict)"(error in=w941, "Visible"=w924) -> (error out=w949:errorcluster)  [unwired: 1 in, 1 out]
                n781 = property on="Period" class="DigNum (strict)"(error in=w949, "Visible"=w924) -> (error out=w948:errorcluster)  [unwired: 1 in, 1 out]
                n782 = property on="Ampl" class="DigNum (strict)"(error in=w948, "Visible"=w924) -> (error out=w947:errorcluster)  [unwired: 1 in, 1 out]
                n783 = property on="HighL" class="DigNum (strict)"(error in=w947, "Visible"=w924) -> (error out=w950:errorcluster)  [unwired: 1 in, 1 out]
                n784 = property on="Offset" class="DigNum (strict)"(error in=w950, "Visible"=w924) -> (error out=w946:errorcluster)  [unwired: 1 in, 1 out]
                n785 = property on="LowL" class="DigNum (strict)"(error in=w946, "Visible"=w924) -> (error out=w945:errorcluster)  [unwired: 1 in, 1 out]
                n786 = property on="PhaseDBL" class="DigNum (strict)"(error in=w945, "Visible"=w924) -> (error out=w951:errorcluster)  [unwired: 1 in, 1 out]
                n787 = property on="Duty" class="DigNum (strict)"(error in=w951, "Visible"=w924) -> (error out=w952:errorcluster)  [unwired: 1 in, 1 out]
                n788 = property on="SymmDBL" class="DigNum (strict)"(error in=w952, "Visible"=w924) -> (error out=w944:errorcluster)  [unwired: 1 in, 1 out]
                n789 = property on="Width" class="DigNum (strict)"(error in=w944, "Visible"=w924) -> (error out=w943:errorcluster)  [unwired: 1 in, 1 out]
                n790 = property on="RisEdgeDBL" class="DigNum (strict)"(error in=w943, "Visible"=w924) -> (error out=w942:errorcluster)  [unwired: 1 in, 1 out]
                n791 = property on="FallEdgeDBL" class="DigNum (strict)"(error in=w942, "Visible"=w924) -> (error out=w925:errorcluster)  [unwired: 1 in, 1 out]
                n792 = property on="OK" class="Bool (strict)"(error in=w925, "Visible"=w924) -> (error out=w923:errorcluster)  [unwired: 1 in, 1 out]
                n793 = property on="Freq-Period" class="Str"(error in=w923, "Visible"=w959) -> (error out=w965:errorcluster)  [unwired: 1 in, 1 out]
                n794 = property on="Freq/Period" class="Bool (strict)"(error in=w923, "Visible"=w959) -> (error out=w962:errorcluster)  [unwired: 1 in, 1 out]
                n795 = property on="Ampl-HighL" class="Str"(error in=w965, "Visible"=w959) -> (error out=w964:errorcluster)  [unwired: 1 in, 1 out]
                n796 = property on="Ampl/HighL" class="Bool (strict)"(error in=w962, "Visible"=w959) -> (error out=w961:errorcluster)  [unwired: 1 in, 1 out]
                n797 = property on="Offset-LowL" class="Str"(error in=w964, "Visible"=w959) -> (error out=w963:errorcluster)  [unwired: 1 in, 1 out]
                n798 = property on="Offset/LowL" class="Bool (strict)"(error in=w961, "Visible"=w959) -> (error out=w960:errorcluster)  [unwired: 1 in, 1 out]
                n799 = property on="PhaseStr" class="Str"(error in=w963, "Visible"=w959) -> (error out=w921:errorcluster)  [unwired: 1 in, 1 out]
                n800 = property on="Slider" class="Bool (strict)"(error in=w960, "Visible"=w959) -> ()  [unwired: 1 in, 2 out]
              }
              frame True {
                w978 = FALSE ("Visible")
                w987 = FALSE ("Visible")
                w973 = FALSE ("Visible")
                w1007 = FALSE ("Visible")
                w968 = TRUE ("Visible")
                # "AllSwapButtonsVisible?"
                # "AllStringsVisible?"
                # "AllValuesVisible?"
                # "AllWaveformsVisible?"
                n801 = property on="Freq-Period" class="Str"(error in=w975, "Visible"=w987) -> (error out=w985:errorcluster)  [unwired: 1 in, 1 out]
                n802 = property on="Ampl-HighL" class="Str"(error in=w985, "Visible"=w987) -> (error out=w984:errorcluster)  [unwired: 1 in, 1 out]
                n803 = property on="Offset-LowL" class="Str"(error in=w984, "Visible"=w987) -> (error out=w983:errorcluster)  [unwired: 1 in, 1 out]
                n804 = property on="PhaseStr" class="Str"(error in=w983, "Visible"=w987) -> (error out=w986:errorcluster)  [unwired: 1 in, 1 out]
                n805 = property on="Duty-Width" class="Str"(error in=w986, "Visible"=w987) -> (error out=w989:errorcluster)  [unwired: 1 in, 1 out]
                n806 = property on="SymmStr" class="Str"(error in=w989, "Visible"=w987) -> (error out=w988:errorcluster)  [unwired: 1 in, 1 out]
                n807 = property on="RisEdgeStr" class="Str"(error in=w988, "Visible"=w987) -> (error out=w982:errorcluster)  [unwired: 1 in, 1 out]
                n808 = property on="FallEdgeStr" class="Str"(error in=w982, "Visible"=w987) -> (error out=w977:errorcluster)  [unwired: 1 in, 1 out]
                n809 = property on="Freq/Period" class="Bool (strict)"(error in=w977, "Visible"=w978) -> (error out=w981:errorcluster)  [unwired: 1 in, 1 out]
                n810 = property on="Ampl/HighL" class="Bool (strict)"(error in=w981, "Visible"=w978) -> (error out=w980:errorcluster)  [unwired: 1 in, 1 out]
                n811 = property on="Offset/LowL" class="Bool (strict)"(error in=w980, "Visible"=w978) -> (error out=w979:errorcluster)  [unwired: 1 in, 1 out]
                n812 = property on="Duty/Width" class="Bool (strict)"(error in=w979, "Visible"=w978) -> (error out=w976:errorcluster)  [unwired: 1 in, 1 out]
                n813 = property on="Sine" class="Bool (strict)"(error in=w976, "Visible"=w1007) -> (error out=w1004:errorcluster)  [unwired: 1 in, 1 out]
                n814 = property on="Square" class="Bool (strict)"(error in=w1004, "Visible"=w1007) -> (error out=w1003:errorcluster)  [unwired: 1 in, 1 out]
                n815 = property on="Ramp" class="Bool (strict)"(error in=w1003, "Visible"=w1007) -> (error out=w1002:errorcluster)  [unwired: 1 in, 1 out]
                n816 = property on="Pulse" class="Bool (strict)"(error in=w1002, "Visible"=w1007) -> (error out=w1005:errorcluster)  [unwired: 1 in, 1 out]
                n817 = property on="Noise" class="Bool (strict)"(error in=w1005, "Visible"=w1007) -> (error out=w1006:errorcluster)  [unwired: 1 in, 1 out]
                n818 = property on="DC" class="Bool (strict)"(error in=w1006, "Visible"=w1007) -> (error out=w990:errorcluster)  [unwired: 1 in, 1 out]
                n819 = property on="Freq" class="DigNum (strict)"(error in=w990, "Visible"=w973) -> (error out=w998:errorcluster)  [unwired: 1 in, 1 out]
                n820 = property on="Period" class="DigNum (strict)"(error in=w998, "Visible"=w973) -> (error out=w997:errorcluster)  [unwired: 1 in, 1 out]
                n821 = property on="Ampl" class="DigNum (strict)"(error in=w997, "Visible"=w973) -> (error out=w996:errorcluster)  [unwired: 1 in, 1 out]
                n822 = property on="HighL" class="DigNum (strict)"(error in=w996, "Visible"=w973) -> (error out=w999:errorcluster)  [unwired: 1 in, 1 out]
                n823 = property on="Offset" class="DigNum (strict)"(error in=w999, "Visible"=w973) -> (error out=w995:errorcluster)  [unwired: 1 in, 1 out]
                n824 = property on="LowL" class="DigNum (strict)"(error in=w995, "Visible"=w973) -> (error out=w994:errorcluster)  [unwired: 1 in, 1 out]
                n825 = property on="PhaseDBL" class="DigNum (strict)"(error in=w994, "Visible"=w973) -> (error out=w1000:errorcluster)  [unwired: 1 in, 1 out]
                n826 = property on="Duty" class="DigNum (strict)"(error in=w1000, "Visible"=w973) -> (error out=w1001:errorcluster)  [unwired: 1 in, 1 out]
                n827 = property on="SymmDBL" class="DigNum (strict)"(error in=w1001, "Visible"=w973) -> (error out=w993:errorcluster)  [unwired: 1 in, 1 out]
                n828 = property on="Width" class="DigNum (strict)"(error in=w993, "Visible"=w973) -> (error out=w992:errorcluster)  [unwired: 1 in, 1 out]
                n829 = property on="RisEdgeDBL" class="DigNum (strict)"(error in=w992, "Visible"=w973) -> (error out=w991:errorcluster)  [unwired: 1 in, 1 out]
                n830 = property on="FallEdgeDBL" class="DigNum (strict)"(error in=w991, "Visible"=w973) -> (error out=w974:errorcluster)  [unwired: 1 in, 1 out]
                n831 = property on="OK" class="Bool (strict)"(error in=w974, "Visible"=w973) -> (error out=w971:errorcluster)  [unwired: 1 in, 1 out]
                n832 = property on="Duty-Width" class="Str"(error in=w971, "Visible"=w968) -> (error out=w969:errorcluster)  [unwired: 1 in, 1 out]
                n833 = property on="Duty/Width" class="Bool (strict)"(error in=w971, "Visible"=w968) -> (error out=w972:errorcluster)  [unwired: 1 in, 1 out]
                n834 = property on="Slider" class="Bool (strict)"(error in=w972, "Visible"=w968) -> ()  [unwired: 1 in, 2 out]
                n835 = property on="RisEdgeStr" class="Str"(error in=w969, "Visible"=w968) -> (error out=w970:errorcluster)  [unwired: 1 in, 1 out]
                n836 = property on="FallEdgeStr" class="Str"(error in=w970, "Visible"=w968) -> (error out=w966:errorcluster)  [unwired: 1 in, 1 out]
              }
            }
          }
          frame 16 {
            w1015 = FALSE ("Visible")
            w1024 = FALSE ("Visible")
            w1039 = FALSE ("Visible")
            w1045 = FALSE ("Visible")
            w1011 = FALSE ("Visible")
            w1012 = TRUE ("Visible")
            # "Noise"
            # "AllSwapButtonsVisible?"
            # "AllStringsVisible?"
            # "AllValuesVisible?"
            # "AllWaveformsVisible?"
            n837 = property on="Freq-Period" class="Str"(error in=w1009, "Visible"=w1024) -> (error out=w1022:errorcluster)  [unwired: 1 in, 1 out]
            n838 = property on="Ampl-HighL" class="Str"(error in=w1022, "Visible"=w1024) -> (error out=w1021:errorcluster)  [unwired: 1 in, 1 out]
            n839 = property on="Offset-LowL" class="Str"(error in=w1021, "Visible"=w1024) -> (error out=w1020:errorcluster)  [unwired: 1 in, 1 out]
            n840 = property on="PhaseStr" class="Str"(error in=w1020, "Visible"=w1024) -> (error out=w1023:errorcluster)  [unwired: 1 in, 1 out]
            n841 = property on="Duty-Width" class="Str"(error in=w1023, "Visible"=w1024) -> (error out=w1026:errorcluster)  [unwired: 1 in, 1 out]
            n842 = property on="SymmStr" class="Str"(error in=w1026, "Visible"=w1024) -> (error out=w1025:errorcluster)  [unwired: 1 in, 1 out]
            n843 = property on="RisEdgeStr" class="Str"(error in=w1025, "Visible"=w1024) -> (error out=w1019:errorcluster)  [unwired: 1 in, 1 out]
            n844 = property on="FallEdgeStr" class="Str"(error in=w1019, "Visible"=w1024) -> (error out=w1014:errorcluster)  [unwired: 1 in, 1 out]
            n845 = property on="Slider" class="Bool (strict)"(error in=w1009, "Visible"=w1011) -> ()  [unwired: 1 in, 2 out]
            n846 = property on="OK" class="Bool (strict)"("Visible"=w1011) -> ()  [unwired: 2 in, 2 out]
            n847 = property on="Freq/Period" class="Bool (strict)"(error in=w1014, "Visible"=w1015) -> (error out=w1018:errorcluster)  [unwired: 1 in, 1 out]
            n848 = property on="Ampl/HighL" class="Bool (strict)"(error in=w1018, "Visible"=w1015) -> (error out=w1017:errorcluster)  [unwired: 1 in, 1 out]
            n849 = property on="Offset/LowL" class="Bool (strict)"(error in=w1017, "Visible"=w1015) -> (error out=w1016:errorcluster)  [unwired: 1 in, 1 out]
            n850 = property on="Duty/Width" class="Bool (strict)"(error in=w1016, "Visible"=w1015) -> (error out=w1013:errorcluster)  [unwired: 1 in, 1 out]
            n851 = property on="Sine" class="Bool (strict)"(error in=w1013, "Visible"=w1045) -> (error out=w1042:errorcluster)  [unwired: 1 in, 1 out]
            n852 = property on="Square" class="Bool (strict)"(error in=w1042, "Visible"=w1045) -> (error out=w1041:errorcluster)  [unwired: 1 in, 1 out]
            n853 = property on="Ramp" class="Bool (strict)"(error in=w1041, "Visible"=w1045) -> (error out=w1040:errorcluster)  [unwired: 1 in, 1 out]
            n854 = property on="Pulse" class="Bool (strict)"(error in=w1040, "Visible"=w1045) -> (error out=w1043:errorcluster)  [unwired: 1 in, 1 out]
            n855 = property on="Noise" class="Bool (strict)"(error in=w1043, "Visible"=w1045) -> (error out=w1044:errorcluster)  [unwired: 1 in, 1 out]
            n856 = property on="DC" class="Bool (strict)"(error in=w1044, "Visible"=w1045) -> (error out=w1027:errorcluster)  [unwired: 1 in, 1 out]
            n857 = property on="Freq" class="DigNum (strict)"(error in=w1027, "Visible"=w1039) -> (error out=w1035:errorcluster)  [unwired: 1 in, 1 out]
            n858 = property on="Period" class="DigNum (strict)"(error in=w1035, "Visible"=w1039) -> (error out=w1034:errorcluster)  [unwired: 1 in, 1 out]
            n859 = property on="Ampl" class="DigNum (strict)"(error in=w1034, "Visible"=w1039) -> (error out=w1033:errorcluster)  [unwired: 1 in, 1 out]
            n860 = property on="HighL" class="DigNum (strict)"(error in=w1033, "Visible"=w1039) -> (error out=w1036:errorcluster)  [unwired: 1 in, 1 out]
            n861 = property on="Offset" class="DigNum (strict)"(error in=w1036, "Visible"=w1039) -> (error out=w1032:errorcluster)  [unwired: 1 in, 1 out]
            n862 = property on="LowL" class="DigNum (strict)"(error in=w1032, "Visible"=w1039) -> (error out=w1031:errorcluster)  [unwired: 1 in, 1 out]
            n863 = property on="PhaseDBL" class="DigNum (strict)"(error in=w1031, "Visible"=w1039) -> (error out=w1037:errorcluster)  [unwired: 1 in, 1 out]
            n864 = property on="Duty" class="DigNum (strict)"(error in=w1037, "Visible"=w1039) -> (error out=w1038:errorcluster)  [unwired: 1 in, 1 out]
            n865 = property on="SymmDBL" class="DigNum (strict)"(error in=w1038, "Visible"=w1039) -> (error out=w1030:errorcluster)  [unwired: 1 in, 1 out]
            n866 = property on="Width" class="DigNum (strict)"(error in=w1030, "Visible"=w1039) -> (error out=w1029:errorcluster)  [unwired: 1 in, 1 out]
            n867 = property on="RisEdgeDBL" class="DigNum (strict)"(error in=w1029, "Visible"=w1039) -> (error out=w1028:errorcluster)  [unwired: 1 in, 1 out]
            n868 = property on="FallEdgeDBL" class="DigNum (strict)"(error in=w1028, "Visible"=w1039) -> (error out=w1010:errorcluster)  [unwired: 1 in, 1 out]
            n869 = property on="Ampl-HighL" class="Str"(error in=w1010, "Visible"=w1012) -> (error out=w1047:errorcluster)  [unwired: 1 in, 1 out]
            n870 = property on="Ampl/HighL" class="Bool (strict)"(error in=w1010, "Visible"=w1012) -> (error out=w1046:errorcluster)  [unwired: 1 in, 1 out]
            n871 = property on="Offset-LowL" class="Str"(error in=w1047, "Visible"=w1012) -> (error out=w1008:errorcluster)  [unwired: 1 in, 1 out]
            n872 = property on="Offset/LowL" class="Bool (strict)"(error in=w1046, "Visible"=w1012) -> ()  [unwired: 1 in, 2 out]
          }
          frame 32 {
            w1056 = FALSE ("Visible")
            w1065 = FALSE ("Visible")
            w1080 = FALSE ("Visible")
            w1086 = FALSE ("Visible")
            w1053 = FALSE ("Visible")
            # "DC"
            # "AllSwapButtonsVisible?"
            # "AllStringsVisible?"
            # "AllValuesVisible?"
            # "AllWaveformsVisible?"
            n873 = property on="Freq-Period" class="Str"(error in=w1052, "Visible"=w1065) -> (error out=w1063:errorcluster)  [unwired: 1 in, 1 out]
            n874 = property on="Ampl-HighL" class="Str"(error in=w1063, "Visible"=w1065) -> (error out=w1062:errorcluster)  [unwired: 1 in, 1 out]
            n875 = property on="Offset-LowL" class="Str"(error in=w1062, "Visible"=w1065) -> (error out=w1061:errorcluster)  [unwired: 1 in, 1 out]
            n876 = property on="PhaseStr" class="Str"(error in=w1061, "Visible"=w1065) -> (error out=w1064:errorcluster)  [unwired: 1 in, 1 out]
            n877 = property on="Duty-Width" class="Str"(error in=w1064, "Visible"=w1065) -> (error out=w1067:errorcluster)  [unwired: 1 in, 1 out]
            n878 = property on="SymmStr" class="Str"(error in=w1067, "Visible"=w1065) -> (error out=w1066:errorcluster)  [unwired: 1 in, 1 out]
            n879 = property on="RisEdgeStr" class="Str"(error in=w1066, "Visible"=w1065) -> (error out=w1060:errorcluster)  [unwired: 1 in, 1 out]
            n880 = property on="FallEdgeStr" class="Str"(error in=w1060, "Visible"=w1065) -> (error out=w1055:errorcluster)  [unwired: 1 in, 1 out]
            n881 = property on="Slider" class="Bool (strict)"(error in=w1052, "Visible"=w1053) -> ()  [unwired: 1 in, 2 out]
            n882 = property on="OK" class="Bool (strict)"("Visible"=w1053) -> ()  [unwired: 2 in, 2 out]
            n883 = property on="Freq/Period" class="Bool (strict)"(error in=w1055, "Visible"=w1056) -> (error out=w1059:errorcluster)  [unwired: 1 in, 1 out]
            n884 = property on="Ampl/HighL" class="Bool (strict)"(error in=w1059, "Visible"=w1056) -> (error out=w1058:errorcluster)  [unwired: 1 in, 1 out]
            n885 = property on="Offset/LowL" class="Bool (strict)"(error in=w1058, "Visible"=w1056) -> (error out=w1057:errorcluster)  [unwired: 1 in, 1 out]
            n886 = property on="Duty/Width" class="Bool (strict)"(error in=w1057, "Visible"=w1056) -> (error out=w1054:errorcluster)  [unwired: 1 in, 1 out]
            n887 = property on="Sine" class="Bool (strict)"(error in=w1054, "Visible"=w1086) -> (error out=w1083:errorcluster)  [unwired: 1 in, 1 out]
            n888 = property on="Square" class="Bool (strict)"(error in=w1083, "Visible"=w1086) -> (error out=w1082:errorcluster)  [unwired: 1 in, 1 out]
            n889 = property on="Ramp" class="Bool (strict)"(error in=w1082, "Visible"=w1086) -> (error out=w1081:errorcluster)  [unwired: 1 in, 1 out]
            n890 = property on="Pulse" class="Bool (strict)"(error in=w1081, "Visible"=w1086) -> (error out=w1084:errorcluster)  [unwired: 1 in, 1 out]
            n891 = property on="Noise" class="Bool (strict)"(error in=w1084, "Visible"=w1086) -> (error out=w1085:errorcluster)  [unwired: 1 in, 1 out]
            n892 = property on="DC" class="Bool (strict)"(error in=w1085, "Visible"=w1086) -> (error out=w1068:errorcluster)  [unwired: 1 in, 1 out]
            n893 = property on="Freq" class="DigNum (strict)"(error in=w1068, "Visible"=w1080) -> (error out=w1076:errorcluster)  [unwired: 1 in, 1 out]
            n894 = property on="Period" class="DigNum (strict)"(error in=w1076, "Visible"=w1080) -> (error out=w1075:errorcluster)  [unwired: 1 in, 1 out]
            n895 = property on="Ampl" class="DigNum (strict)"(error in=w1075, "Visible"=w1080) -> (error out=w1074:errorcluster)  [unwired: 1 in, 1 out]
            n896 = property on="HighL" class="DigNum (strict)"(error in=w1074, "Visible"=w1080) -> (error out=w1077:errorcluster)  [unwired: 1 in, 1 out]
            n897 = property on="Offset" class="DigNum (strict)"(error in=w1077, "Visible"=w1080) -> (error out=w1073:errorcluster)  [unwired: 1 in, 1 out]
            n898 = property on="LowL" class="DigNum (strict)"(error in=w1073, "Visible"=w1080) -> (error out=w1072:errorcluster)  [unwired: 1 in, 1 out]
            n899 = property on="PhaseDBL" class="DigNum (strict)"(error in=w1072, "Visible"=w1080) -> (error out=w1078:errorcluster)  [unwired: 1 in, 1 out]
            n900 = property on="Duty" class="DigNum (strict)"(error in=w1078, "Visible"=w1080) -> (error out=w1079:errorcluster)  [unwired: 1 in, 1 out]
            n901 = property on="SymmDBL" class="DigNum (strict)"(error in=w1079, "Visible"=w1080) -> (error out=w1071:errorcluster)  [unwired: 1 in, 1 out]
            n902 = property on="Width" class="DigNum (strict)"(error in=w1071, "Visible"=w1080) -> (error out=w1070:errorcluster)  [unwired: 1 in, 1 out]
            n903 = property on="RisEdgeDBL" class="DigNum (strict)"(error in=w1070, "Visible"=w1080) -> (error out=w1069:errorcluster)  [unwired: 1 in, 1 out]
            n904 = property on="FallEdgeDBL" class="DigNum (strict)"(error in=w1069, "Visible"=w1080) -> (error out=w1050:errorcluster)  [unwired: 1 in, 1 out]
            n905 = property on="Offset-LowL" class="Str"(error in=w1050, "Visible"=TRUE) -> (error out=w1051:errorcluster)  [unwired: 1 in, 1 out]
          }
        }
        n906 = Build Path(base path=w693, name or relative path=w685) -> (appended path=w692:path)
        n907 = property on="OK" class="Bool (strict)"(error in=w676, "Value"=FALSE ("OK")) -> (error out=w675:errorcluster)  [unwired: 1 in, 1 out]
        n908 = call "RDG822 Update Screen.vi"("error in"=w675, "Path to file"=w692) -> ("error out"=w680:errorcluster, "Screen"=w691:picture)  [unwired: 8 in]
        n909 = local write "Screen"(w691) -> ()
        n910 = stacked-sequence {
          tunnel: [_ _ w1253 _ _ _] -> w688
          tunnel: [_ w1200 _ _ _ _] -> w689
          tunnel: [w1089 _ _ _ _ _] -> w690
          tunnel: w696 -> [w1090 _ _ _ _ _]
          tunnel: w695 -> [_ w1199 _ _ _ _]
          tunnel: w694 -> [_ _ w1252 _ _ _]
          tunnel: [_ _ _ w1321 _ _] -> w687
          tunnel: [_ _ _ _ w1327 _] -> w686
          tunnel: w682 -> [w1088 _ _ _ _ _]
          tunnel: [_ _ _ _ _ w1371] -> w681
          tunnel: w680 -> [_ _ _ _ _ w1370]
          tunnel: [_ _ _ _ _ w1370] -> w679
          tunnel: w678 -> [_ _ _ _ w1326 _]
          tunnel: w677 -> [_ _ _ _ w1325 _]
          frame #0 {
            n911 = case shown="1, Default" w1088 {
              tunnel: w1090 -> [w1091 w1118 w1144 w1170 _]
              tunnel: [w1092 w1117 w1143 w1169 w1195] -> w1089
              frame 1, Default {
                n912 = case shown="True" w1091 {
                  tunnel: [w1101 w1113] -> w1092
                  frame False {
                    n913 = local read "Freq"() -> (w1097:dbl)
                    n914 = In Range and Coerce(upper limit=25000000.0, x=w1097, lower limit=1e-06 ("t")) -> (coerced(x)=w1094:dbl, In Range?=w1096:bool)
                    n915 = case shown="False" w1096 {
                      frame False {
                        n916 = One Button Dialog(message="Sine Wave frequency can`t be lower than 1 uHz\nor higher than 25 MHz!") -> ()  [unwired: 1 in, 1 out]
                      }
                      frame True {
                      }
                    }
                    n917 = Divide(x=1000.0, y=w1094) -> (x/y=w1093:dbl)
                    n918 = local write "Period"(w1093) -> ()
                    n919 = local write "Freq"(w1094) -> ()
                    n920 = Number To Fractional String(number=w1094, precision (6)=i16 6) -> (F-format string=w1100:string)  [unwired: 2 in]
                    n921 = Concatenate Strings(w1100, " Hz" ("string")) -> (w1101:string)
                  }
                  frame True {
                    n922 = local read "Period"() -> (w1108:dbl)
                    n923 = In Range and Coerce(upper limit=1000000000.0, x=w1108, lower limit=4e-05 ("t")) -> (coerced(x)=w1106:dbl, In Range?=w1109:bool)
                    n924 = case shown="False" w1109 {
                      frame False {
                        n925 = One Button Dialog(message="Sine Wave period can`t be lower than 40 ns or higher than 1 Ms!") -> ()  [unwired: 1 in, 1 out]
                      }
                      frame True {
                      }
                    }
                    n926 = Divide(x=1000.0, y=w1106) -> (x/y=w1105:dbl)
                    n927 = local write "Period"(w1106) -> ()
                    n928 = local write "Freq"(w1105) -> ()
                    n929 = Number To Fractional String(number=w1106, precision (6)=i16 7) -> (F-format string=w1112:string)  [unwired: 2 in]
                    n930 = Concatenate Strings(w1112, " ms" ("string")) -> (w1113:string)
                  }
                }
              }
              frame 2 {
                n931 = case shown="False" w1118 {
                  tunnel: [w1127 w1139] -> w1117
                  frame False {
                    n932 = local read "Freq"() -> (w1123:dbl)
                    n933 = In Range and Coerce(upper limit=10000000.0, x=w1123, lower limit=1e-06 ("t")) -> (coerced(x)=w1120:dbl, In Range?=w1122:bool)
                    n934 = case shown="False" w1122 {
                      frame False {
                        n935 = One Button Dialog(message="Square Wave frequency can`t be lower than 1 uHz\nor higher than 10 MHz!") -> ()  [unwired: 1 in, 1 out]
                      }
                      frame True {
                      }
                    }
                    n936 = Divide(x=1000.0, y=w1120) -> (x/y=w1119:dbl)
                    n937 = local write "Period"(w1119) -> ()
                    n938 = local write "Freq"(w1120) -> ()
                    n939 = Number To Fractional String(number=w1120, precision (6)=i16 6) -> (F-format string=w1126:string)  [unwired: 2 in]
                    n940 = Concatenate Strings(w1126, " Hz" ("string")) -> (w1127:string)
                  }
                  frame True {
                    n941 = local read "Period"() -> (w1134:dbl)
                    n942 = In Range and Coerce(upper limit=1000000000.0, x=w1134, lower limit=0.0001 ("t")) -> (coerced(x)=w1132:dbl, In Range?=w1135:bool)
                    n943 = case shown="False" w1135 {
                      frame False {
                        n944 = One Button Dialog(message="Square Wave period can`t be lower than 100 ns or higher than 1 Ms!") -> ()  [unwired: 1 in, 1 out]
                      }
                      frame True {
                      }
                    }
                    n945 = Divide(x=1000.0, y=w1132) -> (x/y=w1131:dbl)
                    n946 = local write "Period"(w1132) -> ()
                    n947 = local write "Freq"(w1131) -> ()
                    n948 = Number To Fractional String(number=w1132, precision (6)=i16 7) -> (F-format string=w1138:string)  [unwired: 2 in]
                    n949 = Concatenate Strings(w1138, " ms" ("string")) -> (w1139:string)
                  }
                }
              }
              frame 4 {
                n950 = case shown="True" w1144 {
                  tunnel: [w1153 w1165] -> w1143
                  frame False {
                    n951 = local read "Freq"() -> (w1149:dbl)
                    n952 = In Range and Coerce(upper limit=500000.0, x=w1149, lower limit=1e-06 ("t")) -> (coerced(x)=w1146:dbl, In Range?=w1148:bool)
                    n953 = case shown="False" w1148 {
                      frame False {
                        n954 = One Button Dialog(message="Ramp Wave frequency can`t be lower than 1 uHz\nor higher than 500 kHz!") -> ()  [unwired: 1 in, 1 out]
                      }
                      frame True {
                      }
                    }
                    n955 = Divide(x=1000.0, y=w1146) -> (x/y=w1145:dbl)
                    n956 = local write "Period"(w1145) -> ()
                    n957 = local write "Freq"(w1146) -> ()
                    n958 = Number To Fractional String(number=w1146, precision (6)=i16 6) -> (F-format string=w1152:string)  [unwired: 2 in]
                    n959 = Concatenate Strings(w1152, " Hz" ("string")) -> (w1153:string)
                  }
                  frame True {
                    n960 = local read "Period"() -> (w1160:dbl)
                    n961 = In Range and Coerce(upper limit=1000000000.0, x=w1160, lower limit=0.002 ("t")) -> (coerced(x)=w1158:dbl, In Range?=w1161:bool)
                    n962 = case shown="False" w1161 {
                      frame False {
                        n963 = One Button Dialog(message="Ramp Wave period can`t be lower than 2 us or higher than 1 Ms!") -> ()  [unwired: 1 in, 1 out]
                      }
                      frame True {
                      }
                    }
                    n964 = Divide(x=1000.0, y=w1158) -> (x/y=w1157:dbl)
                    n965 = local write "Period"(w1158) -> ()
                    n966 = local write "Freq"(w1157) -> ()
                    n967 = Number To Fractional String(number=w1158, precision (6)=i16 7) -> (F-format string=w1164:string)  [unwired: 2 in]
                    n968 = Concatenate Strings(w1164, " ms" ("string")) -> (w1165:string)
                  }
                }
              }
              frame 8 {
                n969 = case shown="False" w1170 {
                  tunnel: [w1179 w1191] -> w1169
                  frame False {
                    n970 = local read "Freq"() -> (w1175:dbl)
                    n971 = In Range and Coerce(upper limit=10000000.0, x=w1175, lower limit=1e-06 ("t")) -> (coerced(x)=w1172:dbl, In Range?=w1174:bool)
                    n972 = case shown="False" w1174 {
                      frame False {
                        n973 = One Button Dialog(message="Pulse Wave frequency can`t be lower than 1 uHz\nor higher than 10 MHz!") -> ()  [unwired: 1 in, 1 out]
                      }
                      frame True {
                      }
                    }
                    n974 = Divide(x=1000.0, y=w1172) -> (x/y=w1171:dbl)
                    n975 = local write "Period"(w1171) -> ()
                    n976 = local write "Freq"(w1172) -> ()
                    n977 = Number To Fractional String(number=w1172, precision (6)=i16 6) -> (F-format string=w1178:string)  [unwired: 2 in]
                    n978 = Concatenate Strings(w1178, " Hz" ("string")) -> (w1179:string)
                  }
                  frame True {
                    n979 = local read "Period"() -> (w1186:dbl)
                    n980 = In Range and Coerce(upper limit=1000000000.0, x=w1186, lower limit=0.0001 ("t")) -> (coerced(x)=w1184:dbl, In Range?=w1187:bool)
                    n981 = case shown="False" w1187 {
                      frame False {
                        n982 = One Button Dialog(message="Pulse Wave period can`t be lower than 100 ns or higher than 1 Ms!") -> ()  [unwired: 1 in, 1 out]
                      }
                      frame True {
                      }
                    }
                    n983 = Divide(x=1000.0, y=w1184) -> (x/y=w1183:dbl)
                    n984 = local write "Period"(w1184) -> ()
                    n985 = local write "Freq"(w1183) -> ()
                    n986 = Number To Fractional String(number=w1184, precision (6)=i16 7) -> (F-format string=w1190:string)  [unwired: 2 in]
                    n987 = Concatenate Strings(w1190, " ms" ("string")) -> (w1191:string)
                  }
                }
              }
              frame 16 {
                n988 = local read "Freq-Period"() -> (w1195:string)
              }
            }
          }
          frame #1 {
            n989 = local read "Freq"() -> (w1198:dbl)
            n990 = Greater?(x=w1198, y=10000000.0 ("upper limit")) -> (0:w1196:bool)
            n991 = case shown="False" w1196 {
              tunnel: [w1202 w1225] -> w1200
              tunnel: w1199 -> [w1201 w1226]
              frame False {
                n992 = case shown="False" w1201 {
                  tunnel: [w1205 w1220] -> w1202
                  frame False {
                    n993 = local read "Ampl"() -> (w1210:dbl)
                    n994 = In Range and Coerce(upper limit=20.0, x=w1210, lower limit=0.002 ("t")) -> (coerced(x)=w1204:dbl, In Range?=w1208:bool)
                    n995 = case shown="False" w1208 {
                      frame False {
                        n996 = One Button Dialog(message="Amplitude can`t be lower than 2 mVpp\nor higher than 20 Vpp!") -> ()  [unwired: 1 in, 1 out]
                      }
                      frame True {
                      }
                    }
                    n997 = local write "Ampl"(w1204) -> ()
                    n998 = Number To Fractional String(number=w1204, precision (6)=i16 4) -> (F-format string=w1206:string)  [unwired: 2 in]
                    n999 = Concatenate Strings(w1206, " Vpp" ("string")) -> (w1205:string)
                  }
                  frame True {
                    n1000 = local read "HighL"() -> (w1218:dbl)
                    n1001 = local read "LowL"() -> (w1214:dbl)
                    n1002 = Add(x=w1214, y=0.002) -> (x+y=w1213:dbl)
                    n1003 = In Range and Coerce(upper limit=10.0, x=w1218, lower limit=w1213) -> (coerced(x)=w1217:dbl, In Range?=w1216:bool)
                    n1004 = case shown="False" w1216 {
                      frame False {
                        n1005 = One Button Dialog(message="HighL can`t be higher than 10 V or less than 2 mV higher than LowL!\n") -> ()  [unwired: 1 in, 1 out]
                      }
                      frame True {
                      }
                    }
                    n1006 = local write "HighL"(w1217) -> ()
                    n1007 = Number To Fractional String(number=w1217, precision (6)=i16 4) -> (F-format string=w1221:string)  [unwired: 2 in]
                    n1008 = Concatenate Strings(w1221, " V" ("string")) -> (w1220:string)
                  }
                }
              }
              frame True {
                n1009 = case shown="True" w1226 {
                  tunnel: [w1229 w1244] -> w1225
                  frame False {
                    n1010 = local read "Ampl"() -> (w1234:dbl)
                    n1011 = In Range and Coerce(upper limit=10.0, x=w1234, lower limit=0.002 ("t")) -> (coerced(x)=w1228:dbl, In Range?=w1232:bool)
                    n1012 = case shown="False" w1232 {
                      frame False {
                        n1013 = One Button Dialog(message="Amplitude can`t be lower than 2 mVpp\nor higher than 10 Vpp!") -> ()  [unwired: 1 in, 1 out]
                      }
                      frame True {
                      }
                    }
                    n1014 = local write "Ampl"(w1228) -> ()
                    n1015 = Number To Fractional String(number=w1228, precision (6)=i16 4) -> (F-format string=w1230:string)  [unwired: 2 in]
                    n1016 = Concatenate Strings(w1230, " Vpp" ("string")) -> (w1229:string)
                  }
                  frame True {
                    n1017 = local read "HighL"() -> (w1242:dbl)
                    n1018 = local read "LowL"() -> (w1238:dbl)
                    n1019 = Add(x=w1238, y=0.002) -> (x+y=w1237:dbl)
                    n1020 = In Range and Coerce(upper limit=5.0, x=w1242, lower limit=w1237) -> (coerced(x)=w1241:dbl, In Range?=w1240:bool)
                    n1021 = case shown="False" w1240 {
                      frame False {
                        n1022 = One Button Dialog(message="HighL can`t be higher than 5 V or less than 2 mV higher than LowL!\n") -> ()  [unwired: 1 in, 1 out]
                      }
                      frame True {
                      }
                    }
                    n1023 = local write "HighL"(w1241) -> ()
                    n1024 = Number To Fractional String(number=w1241, precision (6)=i16 4) -> (F-format string=w1245:string)  [unwired: 2 in]
                    n1025 = Concatenate Strings(w1245, " V" ("string")) -> (w1244:string)
                  }
                }
              }
            }
          }
          frame #2 {
            n1026 = local read "Freq"() -> (w1251:dbl)
            n1027 = Greater?(x=w1251, y=10000000.0 ("upper limit")) -> (0:w1249:bool)
            n1028 = case shown="False" w1249 {
              tunnel: [w1255 w1287] -> w1253
              tunnel: w1252 -> [w1254 w1286]
              frame False {
                n1029 = case shown="False" w1254 {
                  tunnel: [w1270 w1281] -> w1255
                  frame False {
                    n1030 = local read "Ampl"() -> (w1265:dbl)
                    n1031 = local read "Ampl"() -> (w1260:dbl)
                    n1032 = Subtract(x=20.0, y=w1265) -> (x-y=w1264:dbl)
                    n1033 = Add(x=-20.0, y=w1260) -> (x+y=w1261:dbl)
                    n1034 = local read "Offset"() -> (w1267:dbl)
                    n1035 = Divide(x=w1264, y=2.0) -> (x/y=w1262:dbl)
                    n1036 = Divide(x=w1261, y=2.0) -> (x/y=w1259:dbl)
                    n1037 = In Range and Coerce(upper limit=w1262, x=w1267, lower limit=w1259) -> (coerced(x)=w1256:dbl, In Range?=w1268:bool)
                    n1038 = case shown="False" w1268 {
                      frame False {
                        n1039 = One Button Dialog(message="Offset upper and lower limit can`t exceed (20 - Ampl)/2 value") -> ()  [unwired: 1 in, 1 out]
                      }
                      frame True {
                      }
                    }
                    n1040 = local write "Offset"(w1256) -> ()
                    n1041 = Number To Fractional String(number=w1256, precision (6)=i16 4) -> (F-format string=w1269:string)  [unwired: 2 in]
                    n1042 = Concatenate Strings(w1269, " Vdc" ("string")) -> (w1270:string)
                  }
                  frame True {
                    n1043 = local read "LowL"() -> (w1279:dbl)
                    n1044 = local read "HighL"() -> (w1276:dbl)
                    n1045 = Subtract(x=w1276, y=0.002) -> (x-y=w1274:dbl)
                    n1046 = In Range and Coerce(upper limit=w1274, x=w1279, lower limit=-10.0 ("upper limit")) -> (coerced(x)=w1278:dbl, In Range?=w1277:bool)
                    n1047 = case shown="False" w1277 {
                      frame False {
                        n1048 = One Button Dialog(message="LowL can`t be lower  than -10 V or less than 2 mV lower than HighL!\n") -> ()  [unwired: 1 in, 1 out]
                      }
                      frame True {
                      }
                    }
                    n1049 = local write "LowL"(w1278) -> ()
                    n1050 = Number To Fractional String(number=w1278, precision (6)=i16 4) -> (F-format string=w1282:string)  [unwired: 2 in]
                    n1051 = Concatenate Strings(w1282, " V" ("string")) -> (w1281:string)
                  }
                }
              }
              frame True {
                n1052 = case shown="False" w1286 {
                  tunnel: [w1302 w1313] -> w1287
                  frame False {
                    n1053 = local read "Ampl"() -> (w1297:dbl)
                    n1054 = local read "Ampl"() -> (w1292:dbl)
                    n1055 = Subtract(x=10.0, y=w1297) -> (x-y=w1296:dbl)
                    n1056 = Add(x=-10.0, y=w1292) -> (x+y=w1293:dbl)
                    n1057 = local read "Offset"() -> (w1299:dbl)
                    n1058 = Divide(x=w1296, y=2.0) -> (x/y=w1294:dbl)
                    n1059 = Divide(x=w1293, y=2.0) -> (x/y=w1291:dbl)
                    n1060 = In Range and Coerce(upper limit=w1294, x=w1299, lower limit=w1291) -> (coerced(x)=w1288:dbl, In Range?=w1300:bool)
                    n1061 = case shown="False" w1300 {
                      frame False {
                        n1062 = One Button Dialog(message="Offset upper and lower limit can`t exceed (10 - Ampl)/2 value") -> ()  [unwired: 1 in, 1 out]
                      }
                      frame True {
                      }
                    }
                    n1063 = local write "Offset"(w1288) -> ()
                    n1064 = Number To Fractional String(number=w1288, precision (6)=i16 4) -> (F-format string=w1301:string)  [unwired: 2 in]
                    n1065 = Concatenate Strings(w1301, " Vdc" ("string")) -> (w1302:string)
                  }
                  frame True {
                    n1066 = local read "LowL"() -> (w1311:dbl)
                    n1067 = local read "HighL"() -> (w1308:dbl)
                    n1068 = Subtract(x=w1308, y=0.002) -> (x-y=w1306:dbl)
                    n1069 = In Range and Coerce(upper limit=w1306, x=w1311, lower limit=-5.0 ("upper limit")) -> (coerced(x)=w1310:dbl, In Range?=w1309:bool)
                    n1070 = case shown="False" w1309 {
                      frame False {
                        n1071 = One Button Dialog(message="LowL can`t be lower  than -5 V or less than 2 mV lower than HighL!\n") -> ()  [unwired: 1 in, 1 out]
                      }
                      frame True {
                      }
                    }
                    n1072 = local write "LowL"(w1310) -> ()
                    n1073 = Number To Fractional String(number=w1310, precision (6)=i16 4) -> (F-format string=w1314:string)  [unwired: 2 in]
                    n1074 = Concatenate Strings(w1314, " V" ("string")) -> (w1313:string)
                  }
                }
              }
            }
          }
          frame #3 {
            n1075 = local read "PhaseDBL"() -> (w1320:dbl)
            n1076 = Quotient & Remainder(x=w1320, y=360.0) -> (x-y*floor(x/y)=w1318:dbl)  [unwired: 1 out]
            n1077 = local write "PhaseDBL"(w1318) -> ()
            n1078 = Number To Fractional String(number=w1318, precision (6)=i16 3) -> (F-format string=w1322:string)  [unwired: 2 in]
            n1079 = Concatenate Strings(w1322, " °" ("string")) -> (w1321:string)
          }
          frame #4 {
            n1080 = case shown="True" w1326 {
              tunnel: [w1338 w1343] -> w1327
              tunnel: w1325 -> [_ w1342]
              frame False {
                n1081 = local read "Duty"() -> (w1336:dbl)
                n1082 = In Range and Coerce(upper limit=87.0, x=w1336, lower limit=13.0 ("upper limit")) -> (coerced(x)=w1331:dbl, In Range?=w1333:bool)
                n1083 = case shown="False" w1333 {
                  frame False {
                    n1084 = One Button Dialog(message="Duty Cycle can`t be lower than 13 %\nor higher than 87 %!") -> ()  [unwired: 1 in, 1 out]
                  }
                  frame True {
                  }
                }
                n1085 = Divide(x=w1331, y=0.1) -> (x/y=w1330:dbl)
                n1086 = local read "Period"() -> (w1329:dbl)
                n1087 = local write "Duty"(w1331) -> ()
                n1088 = Multiply(x=w1330, y=w1329) -> (x*y=w1328:dbl)
                n1089 = local write "Width"(w1328) -> ()
                n1090 = Number To Fractional String(number=w1331, precision (6)=i16 3) -> (F-format string=w1337:string)  [unwired: 2 in]
                n1091 = Concatenate Strings(w1337, " %" ("string")) -> (w1338:string)
              }
              frame True {
                n1092 = case shown="True" w1342 {
                  tunnel: [w1349 w1365] -> w1343
                  frame False {
                    n1093 = local read "Duty"() -> (w1346:dbl)
                    n1094 = local read "Period"() -> (w1345:dbl)
                    n1095 = Divide(x=w1346, y=0.1) -> (x/y=w1347:dbl)
                    n1096 = Multiply(x=w1347, y=w1345) -> (x*y=w1344:dbl)
                    n1097 = local write "Width"(w1344) -> ()
                    n1098 = Number To Fractional String(number=w1344, precision (6)=i16 4) -> (F-format string=w1352:string)  [unwired: 2 in]
                    n1099 = Concatenate Strings(w1352, " us" ("string")) -> (w1349:string)
                  }
                  frame True {
                    n1100 = local read "Period"() -> (w1358:dbl)
                    n1101 = local read "Period"() -> (w1354:dbl)
                    n1102 = local read "Width"() -> (w1364:dbl)
                    n1103 = Multiply(x=870.0 ("upper limit"), y=w1358) -> (x*y=w1361:dbl)
                    n1104 = Multiply(x=w1354, y=130.0 ("upper limit")) -> (x*y=w1360:dbl)
                    n1105 = In Range and Coerce(upper limit=w1361, x=w1364, lower limit=w1360) -> (coerced(x)=w1355:dbl, In Range?=w1363:bool)
                    n1106 = case shown="False" w1363 {
                      frame False {
                        n1107 = One Button Dialog(message="Pulse Width can`t be lower than 13 % \nor higher than 87 % of Pulse Period!") -> ()  [unwired: 1 in, 1 out]
                      }
                      frame True {
                      }
                    }
                    n1108 = local write "Width"(w1355) -> ()
                    n1109 = Divide(x=w1355, y=w1354) -> (x/y=w1357:dbl)
                    n1110 = Multiply(x=w1357, y=0.1) -> (x*y=w1353:dbl)
                    n1111 = local write "Duty"(w1353) -> ()
                    n1112 = Number To Fractional String(number=w1355, precision (6)=i16 4) -> (F-format string=w1368:string)  [unwired: 2 in]
                    n1113 = Concatenate Strings(w1368, " us" ("string")) -> (w1365:string)
                  }
                }
              }
            }
          }
          frame #5 {
            n1114 = local read "SymmDBL"() -> (w1376:dbl)
            n1115 = In Range and Coerce(upper limit=100.0, x=w1376, lower limit=0.0 ("upper limit")) -> (coerced(x)=w1372:dbl, In Range?=w1373:bool)
            n1116 = case shown="False" w1373 {
              frame False {
                n1117 = One Button Dialog(message="Symmetry value can`t be lower than 0 %\nor higher than 100 %!") -> ()  [unwired: 1 in, 1 out]
              }
              frame True {
              }
            }
            n1118 = local write "SymmDBL"(w1372) -> ()
            n1119 = Number To Fractional String(number=w1372, precision (6)=i16 1) -> (F-format string=w1377:string)  [unwired: 2 in]
            n1120 = Concatenate Strings(w1377, " %" ("string")) -> (w1371:string)
          }
        }
        n1121 = local write "Freq-Period"(w690) -> ()
        n1122 = local write "Ampl-HighL"(w689) -> ()
        n1123 = local write "Offset-LowL"(w688) -> ()
        n1124 = local write "PhaseStr"(w687) -> ()
        n1125 = local write "Duty-Width"(w686) -> ()
        n1126 = local write "SymmStr"(w681) -> ()
        n1127 = local write "error out"(w679) -> ()
      }
      event "Freq-Period": Mouse Down {
        w1394 = FALSE ("Visible")
        w1396 = FALSE ("Visible")
        w1406 = FALSE ("Visible")
        # "AllValuesVisible?"
        # "AllSwapButtonsVisible?"
        # "AllStringsVisible?"
        n1128 = event-data() -> ()  [unwired: 1 in, 8 out]
        n1129 = property on="Freq-Period" class="Str"("Visible"=w1406) -> (error out=w1404:errorcluster)  [unwired: 2 in, 1 out]
        n1130 = property on="Ampl-HighL" class="Str"(error in=w1404, "Visible"=w1406) -> (error out=w1403:errorcluster)  [unwired: 1 in, 1 out]
        n1131 = property on="Offset-LowL" class="Str"(error in=w1403, "Visible"=w1406) -> (error out=w1402:errorcluster)  [unwired: 1 in, 1 out]
        n1132 = property on="PhaseStr" class="Str"(error in=w1402, "Visible"=w1406) -> (error out=w1405:errorcluster)  [unwired: 1 in, 1 out]
        n1133 = property on="Duty-Width" class="Str"(error in=w1405, "Visible"=w1406) -> (error out=w1408:errorcluster)  [unwired: 1 in, 1 out]
        n1134 = property on="SymmStr" class="Str"(error in=w1408, "Visible"=w1406) -> (error out=w1407:errorcluster)  [unwired: 1 in, 1 out]
        n1135 = property on="RisEdgeStr" class="Str"(error in=w1407, "Visible"=w1406) -> (error out=w1401:errorcluster)  [unwired: 1 in, 1 out]
        n1136 = property on="FallEdgeStr" class="Str"(error in=w1401, "Visible"=w1406) -> (error out=w1395:errorcluster)  [unwired: 1 in, 1 out]
        n1137 = property on="Freq/Period" class="Bool (strict)"(error in=w1395, "Visible"=w1396) -> (error out=w1399:errorcluster)  [unwired: 1 in, 1 out]
        n1138 = property on="Ampl/HighL" class="Bool (strict)"(error in=w1399, "Visible"=w1396) -> (error out=w1398:errorcluster)  [unwired: 1 in, 1 out]
        n1139 = property on="Offset/LowL" class="Bool (strict)"(error in=w1398, "Visible"=w1396) -> (error out=w1397:errorcluster)  [unwired: 1 in, 1 out]
        n1140 = property on="Duty/Width" class="Bool (strict)"(error in=w1397, "Visible"=w1396) -> (error out=w1381:errorcluster)  [unwired: 1 in, 1 out]
        n1141 = property on="Freq" class="DigNum (strict)"(error in=w1381, "Visible"=w1394) -> (error out=w1390:errorcluster)  [unwired: 1 in, 1 out]
        n1142 = property on="Period" class="DigNum (strict)"(error in=w1390, "Visible"=w1394) -> (error out=w1389:errorcluster)  [unwired: 1 in, 1 out]
        n1143 = property on="Ampl" class="DigNum (strict)"(error in=w1389, "Visible"=w1394) -> (error out=w1388:errorcluster)  [unwired: 1 in, 1 out]
        n1144 = property on="HighL" class="DigNum (strict)"(error in=w1388, "Visible"=w1394) -> (error out=w1391:errorcluster)  [unwired: 1 in, 1 out]
        n1145 = property on="Offset" class="DigNum (strict)"(error in=w1391, "Visible"=w1394) -> (error out=w1387:errorcluster)  [unwired: 1 in, 1 out]
        n1146 = property on="LowL" class="DigNum (strict)"(error in=w1387, "Visible"=w1394) -> (error out=w1386:errorcluster)  [unwired: 1 in, 1 out]
        n1147 = property on="PhaseDBL" class="DigNum (strict)"(error in=w1386, "Visible"=w1394) -> (error out=w1392:errorcluster)  [unwired: 1 in, 1 out]
        n1148 = property on="Duty" class="DigNum (strict)"(error in=w1392, "Visible"=w1394) -> (error out=w1393:errorcluster)  [unwired: 1 in, 1 out]
        n1149 = property on="SymmDBL" class="DigNum (strict)"(error in=w1393, "Visible"=w1394) -> (error out=w1385:errorcluster)  [unwired: 1 in, 1 out]
        n1150 = property on="Width" class="DigNum (strict)"(error in=w1385, "Visible"=w1394) -> (error out=w1384:errorcluster)  [unwired: 1 in, 1 out]
        n1151 = property on="RisEdgeDBL" class="DigNum (strict)"(error in=w1384, "Visible"=w1394) -> (error out=w1383:errorcluster)  [unwired: 1 in, 1 out]
        n1152 = property on="FallEdgeDBL" class="DigNum (strict)"(error in=w1383, "Visible"=w1394) -> (error out=w1382:errorcluster)  [unwired: 1 in, 1 out]
        n1153 = case shown="False" w1414 {
          tunnel: [w1421 w1427] -> w1412
          tunnel: w1415 -> [w1419 w1425]
          tunnel: w1382 -> [w1417 w1423]
          tunnel: [w1416 w1422] -> w1411
          frame False {
            n1154 = property on="Freq" class="DigNum (strict)"(error in=w1417, "Visible"=TRUE) -> (error out=w1416:errorcluster)  [unwired: 1 in, 1 out]
            n1155 = Build Path(base path=w1419, name or relative path="Freq.bmp") -> (appended path=w1421:path)
          }
          frame True {
            n1156 = property on="Period" class="DigNum (strict)"(error in=w1423, "Visible"=TRUE) -> (error out=w1422:errorcluster)  [unwired: 1 in, 1 out]
            n1157 = Build Path(base path=w1425, name or relative path="Period.bmp") -> (appended path=w1427:path)
          }
        }
        n1158 = call "RDG822 Update Screen.vi"("error in"=w1411, "Path to file"=w1412) -> ("error out"=w1410:errorcluster, "Screen"=w1409:picture)  [unwired: 8 in]
        n1159 = local write "Screen"(w1409) -> ()
        n1160 = property on="Slider" class="Bool (strict)"("Visible"=FALSE) -> ()  [unwired: 2 in, 2 out]
        n1161 = property on="OK" class="Bool (strict)"("Visible"=TRUE) -> ()  [unwired: 2 in, 2 out]
      }
      event "Ampl-HighL": Mouse Down {
        w1441 = FALSE ("Visible")
        w1443 = FALSE ("Visible")
        w1453 = FALSE ("Visible")
        # "AllValuesVisible?"
        # "AllSwapButtonsVisible?"
        # "AllStringsVisible?"
        n1162 = event-data() -> ()  [unwired: 1 in, 8 out]
        n1163 = property on="Freq-Period" class="Str"("Visible"=w1453) -> (error out=w1451:errorcluster)  [unwired: 2 in, 1 out]
        n1164 = property on="Ampl-HighL" class="Str"(error in=w1451, "Visible"=w1453) -> (error out=w1450:errorcluster)  [unwired: 1 in, 1 out]
        n1165 = property on="Offset-LowL" class="Str"(error in=w1450, "Visible"=w1453) -> (error out=w1449:errorcluster)  [unwired: 1 in, 1 out]
        n1166 = property on="PhaseStr" class="Str"(error in=w1449, "Visible"=w1453) -> (error out=w1452:errorcluster)  [unwired: 1 in, 1 out]
        n1167 = property on="Duty-Width" class="Str"(error in=w1452, "Visible"=w1453) -> (error out=w1455:errorcluster)  [unwired: 1 in, 1 out]
        n1168 = property on="SymmStr" class="Str"(error in=w1455, "Visible"=w1453) -> (error out=w1454:errorcluster)  [unwired: 1 in, 1 out]
        n1169 = property on="RisEdgeStr" class="Str"(error in=w1454, "Visible"=w1453) -> (error out=w1448:errorcluster)  [unwired: 1 in, 1 out]
        n1170 = property on="FallEdgeStr" class="Str"(error in=w1448, "Visible"=w1453) -> (error out=w1442:errorcluster)  [unwired: 1 in, 1 out]
        n1171 = property on="Freq/Period" class="Bool (strict)"(error in=w1442, "Visible"=w1443) -> (error out=w1446:errorcluster)  [unwired: 1 in, 1 out]
        n1172 = property on="Ampl/HighL" class="Bool (strict)"(error in=w1446, "Visible"=w1443) -> (error out=w1445:errorcluster)  [unwired: 1 in, 1 out]
        n1173 = property on="Offset/LowL" class="Bool (strict)"(error in=w1445, "Visible"=w1443) -> (error out=w1444:errorcluster)  [unwired: 1 in, 1 out]
        n1174 = property on="Duty/Width" class="Bool (strict)"(error in=w1444, "Visible"=w1443) -> (error out=w1429:errorcluster)  [unwired: 1 in, 1 out]
        n1175 = property on="Freq" class="DigNum (strict)"(error in=w1429, "Visible"=w1441) -> (error out=w1437:errorcluster)  [unwired: 1 in, 1 out]
        n1176 = property on="Period" class="DigNum (strict)"(error in=w1437, "Visible"=w1441) -> (error out=w1436:errorcluster)  [unwired: 1 in, 1 out]
        n1177 = property on="Ampl" class="DigNum (strict)"(error in=w1436, "Visible"=w1441) -> (error out=w1435:errorcluster)  [unwired: 1 in, 1 out]
        n1178 = property on="HighL" class="DigNum (strict)"(error in=w1435, "Visible"=w1441) -> (error out=w1438:errorcluster)  [unwired: 1 in, 1 out]
        n1179 = property on="Offset" class="DigNum (strict)"(error in=w1438, "Visible"=w1441) -> (error out=w1434:errorcluster)  [unwired: 1 in, 1 out]
        n1180 = property on="LowL" class="DigNum (strict)"(error in=w1434, "Visible"=w1441) -> (error out=w1433:errorcluster)  [unwired: 1 in, 1 out]
        n1181 = property on="PhaseDBL" class="DigNum (strict)"(error in=w1433, "Visible"=w1441) -> (error out=w1439:errorcluster)  [unwired: 1 in, 1 out]
        n1182 = property on="Duty" class="DigNum (strict)"(error in=w1439, "Visible"=w1441) -> (error out=w1440:errorcluster)  [unwired: 1 in, 1 out]
        n1183 = property on="SymmDBL" class="DigNum (strict)"(error in=w1440, "Visible"=w1441) -> (error out=w1432:errorcluster)  [unwired: 1 in, 1 out]
        n1184 = property on="Width" class="DigNum (strict)"(error in=w1432, "Visible"=w1441) -> (error out=w1431:errorcluster)  [unwired: 1 in, 1 out]
        n1185 = property on="RisEdgeDBL" class="DigNum (strict)"(error in=w1431, "Visible"=w1441) -> (error out=w1430:errorcluster)  [unwired: 1 in, 1 out]
        n1186 = property on="FallEdgeDBL" class="DigNum (strict)"(error in=w1430, "Visible"=w1441) -> (error out=w1428:errorcluster)  [unwired: 1 in, 1 out]
        n1187 = case shown="False" w1461 {
          tunnel: [w1468 w1474] -> w1459
          tunnel: w1462 -> [w1466 w1472]
          tunnel: w1428 -> [w1464 w1471]
          tunnel: [w1463 w1469] -> w1458
          frame False {
            n1188 = property on="Ampl" class="DigNum (strict)"(error in=w1464, "Visible"=TRUE) -> (error out=w1463:errorcluster)  [unwired: 1 in, 1 out]
            n1189 = Build Path(base path=w1466, name or relative path="Ampl.bmp") -> (appended path=w1468:path)
          }
          frame True {
            n1190 = property on="HighL" class="DigNum (strict)"(error in=w1471, "Visible"=TRUE) -> (error out=w1469:errorcluster)  [unwired: 1 in, 1 out]
            n1191 = Build Path(base path=w1472, name or relative path="HighL.bmp") -> (appended path=w1474:path)
          }
        }
        n1192 = call "RDG822 Update Screen.vi"("error in"=w1458, "Path to file"=w1459) -> ("error out"=w1457:errorcluster, "Screen"=w1456:picture)  [unwired: 8 in]
        n1193 = local write "Screen"(w1456) -> ()
        n1194 = property on="OK" class="Bool (strict)"("Visible"=TRUE) -> ()  [unwired: 2 in, 2 out]
        n1195 = property on="Slider" class="Bool (strict)"("Visible"=FALSE) -> ()  [unwired: 2 in, 2 out]
      }
      event "Offset-LowL": Mouse Down {
        w1488 = FALSE ("Visible")
        w1490 = FALSE ("Visible")
        w1500 = FALSE ("Visible")
        # "AllValuesVisible?"
        # "AllSwapButtonsVisible?"
        # "AllStringsVisible?"
        n1196 = event-data() -> ()  [unwired: 1 in, 8 out]
        n1197 = property on="Freq-Period" class="Str"("Visible"=w1500) -> (error out=w1498:errorcluster)  [unwired: 2 in, 1 out]
        n1198 = property on="Ampl-HighL" class="Str"(error in=w1498, "Visible"=w1500) -> (error out=w1497:errorcluster)  [unwired: 1 in, 1 out]
        n1199 = property on="Offset-LowL" class="Str"(error in=w1497, "Visible"=w1500) -> (error out=w1496:errorcluster)  [unwired: 1 in, 1 out]
        n1200 = property on="PhaseStr" class="Str"(error in=w1496, "Visible"=w1500) -> (error out=w1499:errorcluster)  [unwired: 1 in, 1 out]
        n1201 = property on="Duty-Width" class="Str"(error in=w1499, "Visible"=w1500) -> (error out=w1502:errorcluster)  [unwired: 1 in, 1 out]
        n1202 = property on="SymmStr" class="Str"(error in=w1502, "Visible"=w1500) -> (error out=w1501:errorcluster)  [unwired: 1 in, 1 out]
        n1203 = property on="RisEdgeStr" class="Str"(error in=w1501, "Visible"=w1500) -> (error out=w1495:errorcluster)  [unwired: 1 in, 1 out]
        n1204 = property on="FallEdgeStr" class="Str"(error in=w1495, "Visible"=w1500) -> (error out=w1489:errorcluster)  [unwired: 1 in, 1 out]
        n1205 = property on="Freq/Period" class="Bool (strict)"(error in=w1489, "Visible"=w1490) -> (error out=w1493:errorcluster)  [unwired: 1 in, 1 out]
        n1206 = property on="Ampl/HighL" class="Bool (strict)"(error in=w1493, "Visible"=w1490) -> (error out=w1492:errorcluster)  [unwired: 1 in, 1 out]
        n1207 = property on="Offset/LowL" class="Bool (strict)"(error in=w1492, "Visible"=w1490) -> (error out=w1491:errorcluster)  [unwired: 1 in, 1 out]
        n1208 = property on="Duty/Width" class="Bool (strict)"(error in=w1491, "Visible"=w1490) -> (error out=w1476:errorcluster)  [unwired: 1 in, 1 out]
        n1209 = property on="Freq" class="DigNum (strict)"(error in=w1476, "Visible"=w1488) -> (error out=w1484:errorcluster)  [unwired: 1 in, 1 out]
        n1210 = property on="Period" class="DigNum (strict)"(error in=w1484, "Visible"=w1488) -> (error out=w1483:errorcluster)  [unwired: 1 in, 1 out]
        n1211 = property on="Ampl" class="DigNum (strict)"(error in=w1483, "Visible"=w1488) -> (error out=w1482:errorcluster)  [unwired: 1 in, 1 out]
        n1212 = property on="HighL" class="DigNum (strict)"(error in=w1482, "Visible"=w1488) -> (error out=w1485:errorcluster)  [unwired: 1 in, 1 out]
        n1213 = property on="Offset" class="DigNum (strict)"(error in=w1485, "Visible"=w1488) -> (error out=w1481:errorcluster)  [unwired: 1 in, 1 out]
        n1214 = property on="LowL" class="DigNum (strict)"(error in=w1481, "Visible"=w1488) -> (error out=w1480:errorcluster)  [unwired: 1 in, 1 out]
        n1215 = property on="PhaseDBL" class="DigNum (strict)"(error in=w1480, "Visible"=w1488) -> (error out=w1486:errorcluster)  [unwired: 1 in, 1 out]
        n1216 = property on="Duty" class="DigNum (strict)"(error in=w1486, "Visible"=w1488) -> (error out=w1487:errorcluster)  [unwired: 1 in, 1 out]
        n1217 = property on="SymmDBL" class="DigNum (strict)"(error in=w1487, "Visible"=w1488) -> (error out=w1479:errorcluster)  [unwired: 1 in, 1 out]
        n1218 = property on="Width" class="DigNum (strict)"(error in=w1479, "Visible"=w1488) -> (error out=w1478:errorcluster)  [unwired: 1 in, 1 out]
        n1219 = property on="RisEdgeDBL" class="DigNum (strict)"(error in=w1478, "Visible"=w1488) -> (error out=w1477:errorcluster)  [unwired: 1 in, 1 out]
        n1220 = property on="FallEdgeDBL" class="DigNum (strict)"(error in=w1477, "Visible"=w1488) -> (error out=w1475:errorcluster)  [unwired: 1 in, 1 out]
        n1221 = case shown="False" w1508 {
          tunnel: [w1515 w1521] -> w1506
          tunnel: w1509 -> [w1513 w1519]
          tunnel: w1475 -> [w1511 w1518]
          tunnel: [w1510 w1516] -> w1505
          frame False {
            n1222 = property on="Offset" class="DigNum (strict)"(error in=w1511, "Visible"=TRUE) -> (error out=w1510:errorcluster)  [unwired: 1 in, 1 out]
            n1223 = Build Path(base path=w1513, name or relative path="Offset.bmp") -> (appended path=w1515:path)
          }
          frame True {
            n1224 = property on="LowL" class="DigNum (strict)"(error in=w1518, "Visible"=TRUE) -> (error out=w1516:errorcluster)  [unwired: 1 in, 1 out]
            n1225 = Build Path(base path=w1519, name or relative path="LowL.bmp") -> (appended path=w1521:path)
          }
        }
        n1226 = call "RDG822 Update Screen.vi"("error in"=w1505, "Path to file"=w1506) -> ("error out"=w1504:errorcluster, "Screen"=w1503:picture)  [unwired: 8 in]
        n1227 = local write "Screen"(w1503) -> ()
        n1228 = property on="OK" class="Bool (strict)"("Visible"=TRUE) -> ()  [unwired: 2 in, 2 out]
        n1229 = property on="Slider" class="Bool (strict)"("Visible"=FALSE) -> ()  [unwired: 2 in, 2 out]
      }
      event "PhaseStr": Mouse Down {
        w1535 = FALSE ("Visible")
        w1537 = FALSE ("Visible")
        w1547 = FALSE ("Visible")
        # "AllValuesVisible?"
        # "AllSwapButtonsVisible?"
        # "AllStringsVisible?"
        n1230 = event-data() -> ()  [unwired: 1 in, 8 out]
        n1231 = property on="Freq-Period" class="Str"("Visible"=w1547) -> (error out=w1545:errorcluster)  [unwired: 2 in, 1 out]
        n1232 = property on="Ampl-HighL" class="Str"(error in=w1545, "Visible"=w1547) -> (error out=w1544:errorcluster)  [unwired: 1 in, 1 out]
        n1233 = property on="Offset-LowL" class="Str"(error in=w1544, "Visible"=w1547) -> (error out=w1543:errorcluster)  [unwired: 1 in, 1 out]
        n1234 = property on="PhaseStr" class="Str"(error in=w1543, "Visible"=w1547) -> (error out=w1546:errorcluster)  [unwired: 1 in, 1 out]
        n1235 = property on="Duty-Width" class="Str"(error in=w1546, "Visible"=w1547) -> (error out=w1549:errorcluster)  [unwired: 1 in, 1 out]
        n1236 = property on="SymmStr" class="Str"(error in=w1549, "Visible"=w1547) -> (error out=w1548:errorcluster)  [unwired: 1 in, 1 out]
        n1237 = property on="RisEdgeStr" class="Str"(error in=w1548, "Visible"=w1547) -> (error out=w1542:errorcluster)  [unwired: 1 in, 1 out]
        n1238 = property on="FallEdgeStr" class="Str"(error in=w1542, "Visible"=w1547) -> (error out=w1536:errorcluster)  [unwired: 1 in, 1 out]
        n1239 = property on="Freq/Period" class="Bool (strict)"(error in=w1536, "Visible"=w1537) -> (error out=w1540:errorcluster)  [unwired: 1 in, 1 out]
        n1240 = property on="Ampl/HighL" class="Bool (strict)"(error in=w1540, "Visible"=w1537) -> (error out=w1539:errorcluster)  [unwired: 1 in, 1 out]
        n1241 = property on="Offset/LowL" class="Bool (strict)"(error in=w1539, "Visible"=w1537) -> (error out=w1538:errorcluster)  [unwired: 1 in, 1 out]
        n1242 = property on="Duty/Width" class="Bool (strict)"(error in=w1538, "Visible"=w1537) -> (error out=w1522:errorcluster)  [unwired: 1 in, 1 out]
        n1243 = Build Path(base path=w1556, name or relative path="Phase.bmp") -> (appended path=w1553:path)
        n1244 = property on="Freq" class="DigNum (strict)"(error in=w1522, "Visible"=w1535) -> (error out=w1531:errorcluster)  [unwired: 1 in, 1 out]
        n1245 = property on="Period" class="DigNum (strict)"(error in=w1531, "Visible"=w1535) -> (error out=w1530:errorcluster)  [unwired: 1 in, 1 out]
        n1246 = property on="Ampl" class="DigNum (strict)"(error in=w1530, "Visible"=w1535) -> (error out=w1529:errorcluster)  [unwired: 1 in, 1 out]
        n1247 = property on="HighL" class="DigNum (strict)"(error in=w1529, "Visible"=w1535) -> (error out=w1532:errorcluster)  [unwired: 1 in, 1 out]
        n1248 = property on="Offset" class="DigNum (strict)"(error in=w1532, "Visible"=w1535) -> (error out=w1528:errorcluster)  [unwired: 1 in, 1 out]
        n1249 = property on="LowL" class="DigNum (strict)"(error in=w1528, "Visible"=w1535) -> (error out=w1527:errorcluster)  [unwired: 1 in, 1 out]
        n1250 = property on="PhaseDBL" class="DigNum (strict)"(error in=w1527, "Visible"=w1535) -> (error out=w1533:errorcluster)  [unwired: 1 in, 1 out]
        n1251 = property on="Duty" class="DigNum (strict)"(error in=w1533, "Visible"=w1535) -> (error out=w1534:errorcluster)  [unwired: 1 in, 1 out]
        n1252 = property on="SymmDBL" class="DigNum (strict)"(error in=w1534, "Visible"=w1535) -> (error out=w1526:errorcluster)  [unwired: 1 in, 1 out]
        n1253 = property on="Width" class="DigNum (strict)"(error in=w1526, "Visible"=w1535) -> (error out=w1525:errorcluster)  [unwired: 1 in, 1 out]
        n1254 = property on="RisEdgeDBL" class="DigNum (strict)"(error in=w1525, "Visible"=w1535) -> (error out=w1524:errorcluster)  [unwired: 1 in, 1 out]
        n1255 = property on="FallEdgeDBL" class="DigNum (strict)"(error in=w1524, "Visible"=w1535) -> (error out=w1523:errorcluster)  [unwired: 1 in, 1 out]
        n1256 = property on="PhaseDBL" class="DigNum (strict)"(error in=w1523, "Visible"=TRUE) -> (error out=w1552:errorcluster)  [unwired: 1 in, 1 out]
        n1257 = call "RDG822 Update Screen.vi"("error in"=w1552, "Path to file"=w1553) -> ("error out"=w1551:errorcluster, "Screen"=w1550:picture)  [unwired: 8 in]
        n1258 = local write "Screen"(w1550) -> ()
        n1259 = property on="OK" class="Bool (strict)"("Visible"=TRUE) -> ()  [unwired: 2 in, 2 out]
        n1260 = property on="Slider" class="Bool (strict)"("Visible"=FALSE) -> ()  [unwired: 2 in, 2 out]
      }
      event "Duty-Width": Mouse Down {
        w1571 = FALSE ("Visible")
        w1573 = FALSE ("Visible")
        w1583 = FALSE ("Visible")
        # "AllValuesVisible?"
        # "AllSwapButtonsVisible?"
        # "AllStringsVisible?"
        n1261 = event-data() -> ()  [unwired: 1 in, 8 out]
        n1262 = property on="Freq-Period" class="Str"("Visible"=w1583) -> (error out=w1581:errorcluster)  [unwired: 2 in, 1 out]
        n1263 = property on="Ampl-HighL" class="Str"(error in=w1581, "Visible"=w1583) -> (error out=w1580:errorcluster)  [unwired: 1 in, 1 out]
        n1264 = property on="Offset-LowL" class="Str"(error in=w1580, "Visible"=w1583) -> (error out=w1579:errorcluster)  [unwired: 1 in, 1 out]
        n1265 = property on="PhaseStr" class="Str"(error in=w1579, "Visible"=w1583) -> (error out=w1582:errorcluster)  [unwired: 1 in, 1 out]
        n1266 = property on="Duty-Width" class="Str"(error in=w1582, "Visible"=w1583) -> (error out=w1585:errorcluster)  [unwired: 1 in, 1 out]
        n1267 = property on="SymmStr" class="Str"(error in=w1585, "Visible"=w1583) -> (error out=w1584:errorcluster)  [unwired: 1 in, 1 out]
        n1268 = property on="RisEdgeStr" class="Str"(error in=w1584, "Visible"=w1583) -> (error out=w1578:errorcluster)  [unwired: 1 in, 1 out]
        n1269 = property on="FallEdgeStr" class="Str"(error in=w1578, "Visible"=w1583) -> (error out=w1572:errorcluster)  [unwired: 1 in, 1 out]
        n1270 = property on="Freq/Period" class="Bool (strict)"(error in=w1572, "Visible"=w1573) -> (error out=w1576:errorcluster)  [unwired: 1 in, 1 out]
        n1271 = property on="Ampl/HighL" class="Bool (strict)"(error in=w1576, "Visible"=w1573) -> (error out=w1575:errorcluster)  [unwired: 1 in, 1 out]
        n1272 = property on="Offset/LowL" class="Bool (strict)"(error in=w1575, "Visible"=w1573) -> (error out=w1574:errorcluster)  [unwired: 1 in, 1 out]
        n1273 = property on="Duty/Width" class="Bool (strict)"(error in=w1574, "Visible"=w1573) -> (error out=w1558:errorcluster)  [unwired: 1 in, 1 out]
        n1274 = property on="Freq" class="DigNum (strict)"(error in=w1558, "Visible"=w1571) -> (error out=w1567:errorcluster)  [unwired: 1 in, 1 out]
        n1275 = property on="Period" class="DigNum (strict)"(error in=w1567, "Visible"=w1571) -> (error out=w1566:errorcluster)  [unwired: 1 in, 1 out]
        n1276 = property on="Ampl" class="DigNum (strict)"(error in=w1566, "Visible"=w1571) -> (error out=w1565:errorcluster)  [unwired: 1 in, 1 out]
        n1277 = property on="HighL" class="DigNum (strict)"(error in=w1565, "Visible"=w1571) -> (error out=w1568:errorcluster)  [unwired: 1 in, 1 out]
        n1278 = property on="Offset" class="DigNum (strict)"(error in=w1568, "Visible"=w1571) -> (error out=w1564:errorcluster)  [unwired: 1 in, 1 out]
        n1279 = property on="LowL" class="DigNum (strict)"(error in=w1564, "Visible"=w1571) -> (error out=w1563:errorcluster)  [unwired: 1 in, 1 out]
        n1280 = property on="PhaseDBL" class="DigNum (strict)"(error in=w1563, "Visible"=w1571) -> (error out=w1569:errorcluster)  [unwired: 1 in, 1 out]
        n1281 = property on="Duty" class="DigNum (strict)"(error in=w1569, "Visible"=w1571) -> (error out=w1570:errorcluster)  [unwired: 1 in, 1 out]
        n1282 = property on="SymmDBL" class="DigNum (strict)"(error in=w1570, "Visible"=w1571) -> (error out=w1562:errorcluster)  [unwired: 1 in, 1 out]
        n1283 = property on="Width" class="DigNum (strict)"(error in=w1562, "Visible"=w1571) -> (error out=w1561:errorcluster)  [unwired: 1 in, 1 out]
        n1284 = property on="RisEdgeDBL" class="DigNum (strict)"(error in=w1561, "Visible"=w1571) -> (error out=w1560:errorcluster)  [unwired: 1 in, 1 out]
        n1285 = property on="FallEdgeDBL" class="DigNum (strict)"(error in=w1560, "Visible"=w1571) -> (error out=w1559:errorcluster)  [unwired: 1 in, 1 out]
        n1286 = case shown="False" w1586 {
          tunnel: [w1598 w1604] -> w1588
          tunnel: w1587 -> [w1596 w1602]
          tunnel: w1559 -> [w1594 w1600]
          tunnel: [w1593 w1599] -> w1589
          frame False {
            n1287 = property on="Duty" class="DigNum (strict)"(error in=w1594, "Visible"=TRUE) -> (error out=w1593:errorcluster)  [unwired: 1 in, 1 out]
            n1288 = Build Path(base path=w1596, name or relative path="Duty.bmp") -> (appended path=w1598:path)
          }
          frame True {
            n1289 = property on="Width" class="DigNum (strict)"(error in=w1600, "Visible"=TRUE) -> (error out=w1599:errorcluster)  [unwired: 1 in, 1 out]
            n1290 = Build Path(base path=w1602, name or relative path="Width.bmp") -> (appended path=w1604:path)
          }
        }
        n1291 = call "RDG822 Update Screen.vi"("error in"=w1589, "Path to file"=w1588) -> ("error out"=w1591:errorcluster, "Screen"=w1590:picture)  [unwired: 8 in]
        n1292 = local write "Screen"(w1590) -> ()
        n1293 = property on="OK" class="Bool (strict)"("Visible"=TRUE) -> ()  [unwired: 2 in, 2 out]
        n1294 = property on="Slider" class="Bool (strict)"("Visible"=FALSE) -> ()  [unwired: 2 in, 2 out]
      }
      event "SymmStr": Mouse Down {
        w1618 = FALSE ("Visible")
        w1620 = FALSE ("Visible")
        w1630 = FALSE ("Visible")
        # "AllValuesVisible?"
        # "AllSwapButtonsVisible?"
        # "AllStringsVisible?"
        n1295 = event-data() -> ()  [unwired: 1 in, 8 out]
        n1296 = property on="Freq-Period" class="Str"("Visible"=w1630) -> (error out=w1628:errorcluster)  [unwired: 2 in, 1 out]
        n1297 = property on="Ampl-HighL" class="Str"(error in=w1628, "Visible"=w1630) -> (error out=w1627:errorcluster)  [unwired: 1 in, 1 out]
        n1298 = property on="Offset-LowL" class="Str"(error in=w1627, "Visible"=w1630) -> (error out=w1626:errorcluster)  [unwired: 1 in, 1 out]
        n1299 = property on="PhaseStr" class="Str"(error in=w1626, "Visible"=w1630) -> (error out=w1629:errorcluster)  [unwired: 1 in, 1 out]
        n1300 = property on="Duty-Width" class="Str"(error in=w1629, "Visible"=w1630) -> (error out=w1632:errorcluster)  [unwired: 1 in, 1 out]
        n1301 = property on="SymmStr" class="Str"(error in=w1632, "Visible"=w1630) -> (error out=w1631:errorcluster)  [unwired: 1 in, 1 out]
        n1302 = property on="RisEdgeStr" class="Str"(error in=w1631, "Visible"=w1630) -> (error out=w1625:errorcluster)  [unwired: 1 in, 1 out]
        n1303 = property on="FallEdgeStr" class="Str"(error in=w1625, "Visible"=w1630) -> (error out=w1619:errorcluster)  [unwired: 1 in, 1 out]
        n1304 = property on="Freq/Period" class="Bool (strict)"(error in=w1619, "Visible"=w1620) -> (error out=w1623:errorcluster)  [unwired: 1 in, 1 out]
        n1305 = property on="Ampl/HighL" class="Bool (strict)"(error in=w1623, "Visible"=w1620) -> (error out=w1622:errorcluster)  [unwired: 1 in, 1 out]
        n1306 = property on="Offset/LowL" class="Bool (strict)"(error in=w1622, "Visible"=w1620) -> (error out=w1621:errorcluster)  [unwired: 1 in, 1 out]
        n1307 = property on="Duty/Width" class="Bool (strict)"(error in=w1621, "Visible"=w1620) -> (error out=w1606:errorcluster)  [unwired: 1 in, 1 out]
        n1308 = Build Path(base path=w1639, name or relative path="Symm.bmp") -> (appended path=w1637:path)
        n1309 = property on="Freq" class="DigNum (strict)"(error in=w1606, "Visible"=w1618) -> (error out=w1614:errorcluster)  [unwired: 1 in, 1 out]
        n1310 = property on="Period" class="DigNum (strict)"(error in=w1614, "Visible"=w1618) -> (error out=w1613:errorcluster)  [unwired: 1 in, 1 out]
        n1311 = property on="Ampl" class="DigNum (strict)"(error in=w1613, "Visible"=w1618) -> (error out=w1612:errorcluster)  [unwired: 1 in, 1 out]
        n1312 = property on="HighL" class="DigNum (strict)"(error in=w1612, "Visible"=w1618) -> (error out=w1615:errorcluster)  [unwired: 1 in, 1 out]
        n1313 = property on="Offset" class="DigNum (strict)"(error in=w1615, "Visible"=w1618) -> (error out=w1611:errorcluster)  [unwired: 1 in, 1 out]
        n1314 = property on="LowL" class="DigNum (strict)"(error in=w1611, "Visible"=w1618) -> (error out=w1610:errorcluster)  [unwired: 1 in, 1 out]
        n1315 = property on="PhaseDBL" class="DigNum (strict)"(error in=w1610, "Visible"=w1618) -> (error out=w1616:errorcluster)  [unwired: 1 in, 1 out]
        n1316 = property on="Duty" class="DigNum (strict)"(error in=w1616, "Visible"=w1618) -> (error out=w1617:errorcluster)  [unwired: 1 in, 1 out]
        n1317 = property on="SymmDBL" class="DigNum (strict)"(error in=w1617, "Visible"=w1618) -> (error out=w1609:errorcluster)  [unwired: 1 in, 1 out]
        n1318 = property on="Width" class="DigNum (strict)"(error in=w1609, "Visible"=w1618) -> (error out=w1608:errorcluster)  [unwired: 1 in, 1 out]
        n1319 = property on="RisEdgeDBL" class="DigNum (strict)"(error in=w1608, "Visible"=w1618) -> (error out=w1607:errorcluster)  [unwired: 1 in, 1 out]
        n1320 = property on="FallEdgeDBL" class="DigNum (strict)"(error in=w1607, "Visible"=w1618) -> (error out=w1605:errorcluster)  [unwired: 1 in, 1 out]
        n1321 = property on="SymmDBL" class="DigNum (strict)"(error in=w1605, "Visible"=TRUE) -> (error out=w1636:errorcluster)  [unwired: 1 in, 1 out]
        n1322 = call "RDG822 Update Screen.vi"("error in"=w1636, "Path to file"=w1637) -> ("error out"=w1635:errorcluster, "Screen"=w1634:picture)  [unwired: 8 in]
        n1323 = local write "Screen"(w1634) -> ()
        n1324 = property on="OK" class="Bool (strict)"("Visible"=TRUE) -> ()  [unwired: 2 in, 2 out]
        n1325 = property on="Slider" class="Bool (strict)"("Visible"=FALSE) -> ()  [unwired: 2 in, 2 out]
      }
      event "RisEdgeStr": Mouse Down {
        w1654 = FALSE ("Visible")
        w1657 = FALSE ("Visible")
        w1666 = FALSE ("Visible")
        # "AllValuesVisible?"
        # "AllSwapButtonsVisible?"
        # "AllStringsVisible?"
        n1326 = event-data() -> ()  [unwired: 1 in, 8 out]
        n1327 = property on="Freq-Period" class="Str"("Visible"=w1666) -> (error out=w1664:errorcluster)  [unwired: 2 in, 1 out]
        n1328 = property on="Ampl-HighL" class="Str"(error in=w1664, "Visible"=w1666) -> (error out=w1663:errorcluster)  [unwired: 1 in, 1 out]
        n1329 = property on="Offset-LowL" class="Str"(error in=w1663, "Visible"=w1666) -> (error out=w1662:errorcluster)  [unwired: 1 in, 1 out]
        n1330 = property on="PhaseStr" class="Str"(error in=w1662, "Visible"=w1666) -> (error out=w1665:errorcluster)  [unwired: 1 in, 1 out]
        n1331 = property on="Duty-Width" class="Str"(error in=w1665, "Visible"=w1666) -> (error out=w1668:errorcluster)  [unwired: 1 in, 1 out]
        n1332 = property on="SymmStr" class="Str"(error in=w1668, "Visible"=w1666) -> (error out=w1667:errorcluster)  [unwired: 1 in, 1 out]
        n1333 = property on="RisEdgeStr" class="Str"(error in=w1667, "Visible"=w1666) -> (error out=w1661:errorcluster)  [unwired: 1 in, 1 out]
        n1334 = property on="FallEdgeStr" class="Str"(error in=w1661, "Visible"=w1666) -> (error out=w1656:errorcluster)  [unwired: 1 in, 1 out]
        n1335 = property on="Freq/Period" class="Bool (strict)"(error in=w1656, "Visible"=w1657) -> (error out=w1660:errorcluster)  [unwired: 1 in, 1 out]
        n1336 = property on="Ampl/HighL" class="Bool (strict)"(error in=w1660, "Visible"=w1657) -> (error out=w1659:errorcluster)  [unwired: 1 in, 1 out]
        n1337 = property on="Offset/LowL" class="Bool (strict)"(error in=w1659, "Visible"=w1657) -> (error out=w1658:errorcluster)  [unwired: 1 in, 1 out]
        n1338 = property on="Duty/Width" class="Bool (strict)"(error in=w1658, "Visible"=w1657) -> (error out=w1642:errorcluster)  [unwired: 1 in, 1 out]
        n1339 = Build Path(base path=w1675, name or relative path="RisEdge.bmp") -> (appended path=w1672:path)
        n1340 = property on="Freq" class="DigNum (strict)"(error in=w1642, "Visible"=w1654) -> (error out=w1650:errorcluster)  [unwired: 1 in, 1 out]
        n1341 = property on="Period" class="DigNum (strict)"(error in=w1650, "Visible"=w1654) -> (error out=w1649:errorcluster)  [unwired: 1 in, 1 out]
        n1342 = property on="Ampl" class="DigNum (strict)"(error in=w1649, "Visible"=w1654) -> (error out=w1648:errorcluster)  [unwired: 1 in, 1 out]
        n1343 = property on="HighL" class="DigNum (strict)"(error in=w1648, "Visible"=w1654) -> (error out=w1651:errorcluster)  [unwired: 1 in, 1 out]
        n1344 = property on="Offset" class="DigNum (strict)"(error in=w1651, "Visible"=w1654) -> (error out=w1647:errorcluster)  [unwired: 1 in, 1 out]
        n1345 = property on="LowL" class="DigNum (strict)"(error in=w1647, "Visible"=w1654) -> (error out=w1646:errorcluster)  [unwired: 1 in, 1 out]
        n1346 = property on="PhaseDBL" class="DigNum (strict)"(error in=w1646, "Visible"=w1654) -> (error out=w1652:errorcluster)  [unwired: 1 in, 1 out]
        n1347 = property on="Duty" class="DigNum (strict)"(error in=w1652, "Visible"=w1654) -> (error out=w1653:errorcluster)  [unwired: 1 in, 1 out]
        n1348 = property on="SymmDBL" class="DigNum (strict)"(error in=w1653, "Visible"=w1654) -> (error out=w1645:errorcluster)  [unwired: 1 in, 1 out]
        n1349 = property on="Width" class="DigNum (strict)"(error in=w1645, "Visible"=w1654) -> (error out=w1644:errorcluster)  [unwired: 1 in, 1 out]
        n1350 = property on="RisEdgeDBL" class="DigNum (strict)"(error in=w1644, "Visible"=w1654) -> (error out=w1643:errorcluster)  [unwired: 1 in, 1 out]
        n1351 = property on="FallEdgeDBL" class="DigNum (strict)"(error in=w1643, "Visible"=w1654) -> (error out=w1641:errorcluster)  [unwired: 1 in, 1 out]
        n1352 = property on="RisEdgeDBL" class="DigNum (strict)"(error in=w1641, "Visible"=TRUE) -> (error out=w1671:errorcluster)  [unwired: 1 in, 1 out]
        n1353 = call "RDG822 Update Screen.vi"("error in"=w1671, "Path to file"=w1672) -> ("error out"=w1670:errorcluster, "Screen"=w1669:picture)  [unwired: 8 in]
        n1354 = local write "Screen"(w1669) -> ()
        n1355 = property on="OK" class="Bool (strict)"("Visible"=TRUE) -> ()  [unwired: 2 in, 2 out]
        n1356 = property on="Slider" class="Bool (strict)"("Visible"=FALSE) -> ()  [unwired: 2 in, 2 out]
      }
      event "FallEdgeStr": Mouse Down {
        w1690 = FALSE ("Visible")
        w1693 = FALSE ("Visible")
        w1700 = FALSE ("Visible")
        # "AllValuesVisible?"
        # "AllSwapButtonsVisible?"
        # "AllStringsVisible?"
        n1357 = event-data() -> ()  [unwired: 1 in, 8 out]
        n1358 = property on="Freq-Period" class="Str"("Visible"=w1700) -> (error out=w1698:errorcluster)  [unwired: 2 in, 1 out]
        n1359 = property on="Ampl-HighL" class="Str"(error in=w1698, "Visible"=w1700) -> (error out=w1697:errorcluster)  [unwired: 1 in, 1 out]
        n1360 = property on="Offset-LowL" class="Str"(error in=w1697, "Visible"=w1700) -> (error out=w1696:errorcluster)  [unwired: 1 in, 1 out]
        n1361 = property on="PhaseStr" class="Str"(error in=w1696, "Visible"=w1700) -> (error out=w1699:errorcluster)  [unwired: 1 in, 1 out]
        n1362 = property on="Duty-Width" class="Str"(error in=w1699, "Visible"=w1700) -> (error out=w1702:errorcluster)  [unwired: 1 in, 1 out]
        n1363 = property on="SymmStr" class="Str"(error in=w1702, "Visible"=w1700) -> (error out=w1701:errorcluster)  [unwired: 1 in, 1 out]
        n1364 = property on="RisEdgeStr" class="Str"(error in=w1701, "Visible"=w1700) -> (error out=w1695:errorcluster)  [unwired: 1 in, 1 out]
        n1365 = property on="FallEdgeStr" class="Str"(error in=w1695, "Visible"=w1700) -> (error out=w1692:errorcluster)  [unwired: 1 in, 1 out]
        n1366 = property on="Freq/Period" class="Bool (strict)"(error in=w1692, "Visible"=w1693) -> (error out=w1712:errorcluster)  [unwired: 1 in, 1 out]
        n1367 = property on="Ampl/HighL" class="Bool (strict)"(error in=w1712, "Visible"=w1693) -> (error out=w1711:errorcluster)  [unwired: 1 in, 1 out]
        n1368 = property on="Offset/LowL" class="Bool (strict)"(error in=w1711, "Visible"=w1693) -> (error out=w1694:errorcluster)  [unwired: 1 in, 1 out]
        n1369 = property on="Duty/Width" class="Bool (strict)"(error in=w1694, "Visible"=w1693) -> (error out=w1678:errorcluster)  [unwired: 1 in, 1 out]
        n1370 = Build Path(base path=w1709, name or relative path="FallEdge.bmp") -> (appended path=w1706:path)
        n1371 = property on="Freq" class="DigNum (strict)"(error in=w1678, "Visible"=w1690) -> (error out=w1686:errorcluster)  [unwired: 1 in, 1 out]
        n1372 = property on="Period" class="DigNum (strict)"(error in=w1686, "Visible"=w1690) -> (error out=w1685:errorcluster)  [unwired: 1 in, 1 out]
        n1373 = property on="Ampl" class="DigNum (strict)"(error in=w1685, "Visible"=w1690) -> (error out=w1684:errorcluster)  [unwired: 1 in, 1 out]
        n1374 = property on="HighL" class="DigNum (strict)"(error in=w1684, "Visible"=w1690) -> (error out=w1687:errorcluster)  [unwired: 1 in, 1 out]
        n1375 = property on="Offset" class="DigNum (strict)"(error in=w1687, "Visible"=w1690) -> (error out=w1683:errorcluster)  [unwired: 1 in, 1 out]
        n1376 = property on="LowL" class="DigNum (strict)"(error in=w1683, "Visible"=w1690) -> (error out=w1682:errorcluster)  [unwired: 1 in, 1 out]
        n1377 = property on="PhaseDBL" class="DigNum (strict)"(error in=w1682, "Visible"=w1690) -> (error out=w1688:errorcluster)  [unwired: 1 in, 1 out]
        n1378 = property on="Duty" class="DigNum (strict)"(error in=w1688, "Visible"=w1690) -> (error out=w1689:errorcluster)  [unwired: 1 in, 1 out]
        n1379 = property on="SymmDBL" class="DigNum (strict)"(error in=w1689, "Visible"=w1690) -> (error out=w1681:errorcluster)  [unwired: 1 in, 1 out]
        n1380 = property on="Width" class="DigNum (strict)"(error in=w1681, "Visible"=w1690) -> (error out=w1680:errorcluster)  [unwired: 1 in, 1 out]
        n1381 = property on="RisEdgeDBL" class="DigNum (strict)"(error in=w1680, "Visible"=w1690) -> (error out=w1679:errorcluster)  [unwired: 1 in, 1 out]
        n1382 = property on="FallEdgeDBL" class="DigNum (strict)"(error in=w1679, "Visible"=w1690) -> (error out=w1677:errorcluster)  [unwired: 1 in, 1 out]
        n1383 = property on="FallEdgeDBL" class="DigNum (strict)"(error in=w1677, "Visible"=TRUE) -> (error out=w1705:errorcluster)  [unwired: 1 in, 1 out]
        n1384 = call "RDG822 Update Screen.vi"("error in"=w1705, "Path to file"=w1706) -> ("error out"=w1704:errorcluster, "Screen"=w1703:picture)  [unwired: 8 in]
        n1385 = local write "Screen"(w1703) -> ()
        n1386 = property on="Slider" class="Bool (strict)"("Visible"=FALSE) -> ()  [unwired: 2 in, 2 out]
        n1387 = property on="OK" class="Bool (strict)"("Visible"=TRUE) -> ()  [unwired: 2 in, 2 out]
      }
      event "Freq/Period": Value Change {
        n1388 = event-data() -> ("NewVal"=w1713:bool)  [unwired: 1 in, 5 out]
        n1389 = case shown="False" w1713 {
          tunnel: [w1717 w1723] -> w1714
          frame False {
            n1390 = local read "Period"() -> (w1720:dbl)
            n1391 = Divide(x=1000.0, y=w1720) -> (x/y=w1718:dbl)
            n1392 = local write "Freq"(w1718) -> ()
            n1393 = Number To Fractional String(number=w1718, precision (6)=i16 6) -> (F-format string=w1715:string)  [unwired: 2 in]
            n1394 = Concatenate Strings(w1715, " Hz" ("string")) -> (w1717:string)
          }
          frame True {
            n1395 = local read "Freq"() -> (w1726:dbl)
            n1396 = Divide(x=1000.0, y=w1726) -> (x/y=w1725:dbl)
            n1397 = local write "Period"(w1725) -> ()
            n1398 = Number To Fractional String(number=w1725, precision (6)=i16 7) -> (F-format string=w1722:string)  [unwired: 2 in]
            n1399 = Concatenate Strings(w1722, " ms" ("string")) -> (w1723:string)
          }
        }
        n1400 = local write "Freq-Period"(w1714) -> ()
      }
      event "Ampl/HighL": Value Change {
        n1401 = event-data() -> ("NewVal"=w1730:bool)  [unwired: 1 in, 5 out]
        n1402 = case shown="False" w1730 {
          tunnel: [w1740 w1748] -> w1731
          frame False {
            n1403 = local read "HighL"() -> (w1735:dbl)
            n1404 = local read "LowL"() -> (w1734:dbl)
            n1405 = Add(x=w1735, y=w1734) -> (x+y=w1737:dbl)
            n1406 = Divide(x=w1737, y=2.0) -> (x/y=w1733:dbl)
            n1407 = Number To Fractional String(number=w1733, precision (6)=i16 4) -> (F-format string=w1738:string)  [unwired: 2 in]
            n1408 = local write "Offset"(w1733) -> ()
            n1409 = Concatenate Strings(w1738, " Vdc" ("string")) -> (w1740:string)
          }
          frame True {
            n1410 = local read "Offset"() -> (w1744:dbl)
            n1411 = local read "Ampl"() -> (w1743:dbl)
            n1412 = Divide(x=w1743, y=2.0) -> (x/y=w1746:dbl)
            n1413 = Subtract(x=w1744, y=w1746) -> (x-y=w1745:dbl)
            n1414 = local write "LowL"(w1745) -> ()
            n1415 = Number To Fractional String(number=w1745, precision (6)=i16 4) -> (F-format string=w1747:string)  [unwired: 2 in]
            n1416 = Concatenate Strings(w1747, " V" ("string")) -> (w1748:string)
          }
        }
        n1417 = case shown="False" w1730 {
          tunnel: [w1755 w1764] -> w1732
          frame False {
            n1418 = local read "HighL"() -> (w1753:dbl)
            n1419 = local read "LowL"() -> (w1752:dbl)
            n1420 = Subtract(x=w1753, y=w1752) -> (x-y=w1751:dbl)
            n1421 = Number To Fractional String(number=w1751, precision (6)=i16 4) -> (F-format string=w1754:string)  [unwired: 2 in]
            n1422 = local write "Ampl"(w1751) -> ()
            n1423 = Concatenate Strings(w1754, " Vpp" ("string")) -> (w1755:string)
          }
          frame True {
            n1424 = local read "Offset"() -> (w1760:dbl)
            n1425 = local read "Ampl"() -> (w1761:dbl)
            n1426 = Divide(x=w1761, y=2.0) -> (x/y=w1759:dbl)
            n1427 = Add(x=w1760, y=w1759) -> (x+y=w1758:dbl)
            n1428 = Number To Fractional String(number=w1758, precision (6)=i16 4) -> (F-format string=w1763:string)  [unwired: 2 in]
            n1429 = local write "HighL"(w1758) -> ()
            n1430 = Concatenate Strings(w1763, " V" ("string")) -> (w1764:string)
          }
        }
        n1431 = local read "Ampl/HighL"() -> (w1729:bool)
        n1432 = local write "Offset/LowL"(w1729) -> ()
        n1433 = local write "Offset-LowL"(w1731) -> ()
        n1434 = local write "Ampl-HighL"(w1732) -> ()
      }
      event "Offset/LowL": Value Change {
        n1435 = event-data() -> ("NewVal"=w1768:bool)  [unwired: 1 in, 5 out]
        n1436 = case shown="False" w1768 {
          tunnel: [w1778 w1786] -> w1769
          frame False {
            n1437 = local read "HighL"() -> (w1773:dbl)
            n1438 = local read "LowL"() -> (w1772:dbl)
            n1439 = Add(x=w1773, y=w1772) -> (x+y=w1775:dbl)
            n1440 = Divide(x=w1775, y=2.0) -> (x/y=w1771:dbl)
            n1441 = Number To Fractional String(number=w1771, precision (6)=i16 4) -> (F-format string=w1776:string)  [unwired: 2 in]
            n1442 = local write "Offset"(w1771) -> ()
            n1443 = Concatenate Strings(w1776, " Vdc" ("string")) -> (w1778:string)
          }
          frame True {
            n1444 = local read "Offset"() -> (w1782:dbl)
            n1445 = local read "Ampl"() -> (w1781:dbl)
            n1446 = Divide(x=w1781, y=2.0) -> (x/y=w1784:dbl)
            n1447 = Subtract(x=w1782, y=w1784) -> (x-y=w1783:dbl)
            n1448 = local write "LowL"(w1783) -> ()
            n1449 = Number To Fractional String(number=w1783, precision (6)=i16 4) -> (F-format string=w1785:string)  [unwired: 2 in]
            n1450 = Concatenate Strings(w1785, " V" ("string")) -> (w1786:string)
          }
        }
        n1451 = case shown="False" w1768 {
          tunnel: [w1793 w1802] -> w1770
          frame False {
            n1452 = local read "HighL"() -> (w1791:dbl)
            n1453 = local read "LowL"() -> (w1790:dbl)
            n1454 = Subtract(x=w1791, y=w1790) -> (x-y=w1789:dbl)
            n1455 = Number To Fractional String(number=w1789, precision (6)=i16 4) -> (F-format string=w1792:string)  [unwired: 2 in]
            n1456 = local write "Ampl"(w1789) -> ()
            n1457 = Concatenate Strings(w1792, " Vpp" ("string")) -> (w1793:string)
          }
          frame True {
            n1458 = local read "Offset"() -> (w1798:dbl)
            n1459 = local read "Ampl"() -> (w1799:dbl)
            n1460 = Divide(x=w1799, y=2.0) -> (x/y=w1797:dbl)
            n1461 = Add(x=w1798, y=w1797) -> (x+y=w1796:dbl)
            n1462 = Number To Fractional String(number=w1796, precision (6)=i16 4) -> (F-format string=w1801:string)  [unwired: 2 in]
            n1463 = local write "HighL"(w1796) -> ()
            n1464 = Concatenate Strings(w1801, " V" ("string")) -> (w1802:string)
          }
        }
        n1465 = local read "Offset/LowL"() -> (w1767:bool)
        n1466 = local write "Ampl/HighL"(w1767) -> ()
        n1467 = local write "Offset-LowL"(w1769) -> ()
        n1468 = local write "Ampl-HighL"(w1770) -> ()
      }
      event "Duty/Width": Value Change {
        n1469 = event-data() -> ("NewVal"=w1805:bool)  [unwired: 1 in, 5 out]
        n1470 = case shown="True" w1805 {
          tunnel: [w1814 w1822] -> w1806
          frame False {
            n1471 = local read "Period"() -> (w1810:dbl)
            n1472 = local read "Width"() -> (w1811:dbl)
            n1473 = Divide(x=w1811, y=w1810) -> (x/y=w1809:dbl)
            n1474 = Multiply(x=w1809, y=0.1) -> (x*y=w1807:dbl)
            n1475 = local write "Duty"(w1807) -> ()
            n1476 = Number To Fractional String(number=w1807, precision (6)=i16 3) -> (F-format string=w1812:string)  [unwired: 2 in]
            n1477 = Concatenate Strings(w1812, " %" ("string")) -> (w1814:string)
          }
          frame True {
            n1478 = local read "Duty"() -> (w1820:dbl)
            n1479 = local read "Period"() -> (w1817:dbl)
            n1480 = Divide(x=w1820, y=0.1) -> (x/y=w1818:dbl)
            n1481 = Multiply(x=w1818, y=w1817) -> (x*y=w1816:dbl)
            n1482 = local write "Width"(w1816) -> ()
            n1483 = Number To Fractional String(number=w1816, precision (6)=i16 4) -> (F-format string=w1821:string)  [unwired: 2 in]
            n1484 = Concatenate Strings(w1821, " us" ("string")) -> (w1822:string)
          }
        }
        n1485 = local write "Duty-Width"(w1806) -> ()
      }
      event "Out1": Mouse Down {
        w1832 = FALSE ("Visible")
        w1845 = FALSE ("Visible")
        w1852 = FALSE ("Visible")
        w1855 = FALSE ("Visible")
        w1875 = 0 items=["Vpp", "Vrms", "dBm"] ("Amplitude Unit (0: Vpp)")
        w1886 = u16 2 items=["Send", "Read", "Download", "Remove"] ("Send/Read/Download/Remove")
        w1887 = u16 0 items=["Send", "Read", "Download", "Remove"] ("Send/Read/Download/Remove")
        w1890 = 1 items=["Channel 1"=1, "Channel 2"=2] ("Output Channel (1: Channel 1)")
        # "AllWaveformsVisible?"
        # "AllValuesVisible?"
        # "AllStringsVisible?"
        # "AllSwapButtonsVisible?"
        # "Add values checking and coercing before sending (as in OK case)"
        n1486 = event-data() -> ()  [unwired: 1 in, 8 out]
        n1487 = local read "MenuCount"() -> (w1869:u32)
        n1488 = case shown="32" w1869 {
          tunnel: ["Sine" "Square" "Ramp" "Pulse" "Noise" "DC"] -> w1870
          frame 1, Default {
          }
          frame 2 {
          }
          frame 4 {
          }
          frame 8 {
          }
          frame 16 {
          }
          frame 32 {
          }
        }
        n1489 = Quotient & Remainder(x=w1860, y=360.0) -> (x-y*floor(x/y)=w1861:dbl)  [unwired: 1 out]
        n1490 = case shown="True" w1902 {
          tunnel: w1901 -> [w1940 _]
          tunnel: w1862 -> [_ w1942]
          tunnel: [w1940 w1941] -> w1874
          frame False {
            # "Freq"
          }
          frame True {
            # "Period"
            n1491 = Divide(x=1000.0, y=w1942) -> (x/y=w1941:dbl)
          }
        }
        n1492 = case shown="True" w1903 {
          tunnel: w1900 -> [w1931 _]
          tunnel: w1897 -> [_ w1938]
          tunnel: [w1931 w1932] -> w1871
          tunnel: w1898 -> [_ w1937]
          frame False {
            # "Ampl"
          }
          frame True {
            # "High-Low"
            n1493 = Subtract(x=w1938, y=w1937) -> (x-y=w1934:dbl)
            n1494 = In Range and Coerce(upper limit=20.0, x=w1934, lower limit=0.002 ("t")) -> (coerced(x)=w1932:dbl, In Range?=w1933:bool)
            n1495 = case shown="False" w1933 {
              frame False {
                n1496 = One Button Dialog(message="Amplitude can`t be less than 2 mVpp\nor greater than 20 Vpp!") -> ()  [unwired: 1 in, 1 out]
              }
              frame True {
              }
            }
          }
        }
        n1497 = case shown="True" w1899 {
          tunnel: w1873 -> [w1925 _]
          tunnel: w1898 -> [_ w1930]
          tunnel: [w1925 w1926] -> w1872
          tunnel: w1897 -> [_ w1927]
          frame False {
            # "Offset"
          }
          frame True {
            # "HOffset"
            n1498 = Add(x=w1927, y=w1930) -> (x+y=w1929:dbl)
            n1499 = Divide(x=w1929, y=2.0) -> (x/y=w1926:dbl)
          }
        }
        n1500 = case shown="True" w1866 {
          tunnel: w1865 -> [w1904 _]
          tunnel: [w1904 w1907] -> w1864
          tunnel: w1863 -> [_ w1906]
          tunnel: w1862 -> [_ w1905]
          frame False {
            # "Duty"
          }
          frame True {
            # "Width"
            n1501 = Divide(x=w1906, y=w1905) -> (x/y=w1909:dbl)
            n1502 = Multiply(x=w1909, y=100.0) -> (x*y=w1907:dbl)
          }
        }
        n1503 = disable-structure shown="Enabled" {
          disable-tunnel: w1868 -> [_ w1910]
          disable-tunnel: [_ w1911] -> w1867
          frame Disabled {
          }
          frame Enabled {
            n1504 = In Range and Coerce(upper limit=100.0, x=w1910, lower limit=0.0 ("upper limit")) -> (coerced(x)=w1911:dbl)  [unwired: 1 out]
          }
        }
        n1505 = call "RDG822 Standard Waveform.vi"("Configure"=w1870, "Output Channel (1: Channel 1)"=w1890, "Amplitude Unit (0: Vpp)"=w1875, "Phase (0 Degree)"=w1861, "error in (no error)"=w1892, "Amplitude (0.1 Vpp)"=w1871, "Duty Cycle (50 %)"=w1864, "Frequency (1000 Hz)"=w1874, "DC Offset (0.00 V)"=w1872, "Ramp Symmetry (0 %)"=w1867) -> ("resulting string"=w1876:string, "error out"=w1889:errorcluster)  [unwired: 8 in]
        n1506 = call "HTTPGetRequest_Inst.vi"("Send/Read/Download/Remove"=w1887, "error in (no error)"=w1889, "userdata="=w1876, "userID"=w1891) -> ("error out"=w1879:errorcluster, "ReqNum"=w1877:string)  [unwired: 5 in, 1 out]
        n1507 = Build Path(base path=w1880, name or relative path=path "Results") -> (appended path=w1882:path)
        n1508 = call "QueryDoneFlag.vi"("error in (no error)"=w1879, "ReqNum"=w1877) -> ("error out"=w1878:errorcluster)  [unwired: 9 in]
        n1509 = call "HTTPGetRequest_Inst.vi"("Send/Read/Download/Remove"=w1886, "Path to FP"=w1882, "error in (no error)"=w1878, "ReqNum"=w1877) -> ("error out"=w1893:errorcluster)  [unwired: 5 in, 2 out]
        n1510 = call "UnZipFile.vi"("error in (no error)"=w1893, "Zip name"=w1877, "Path to FP"=w1882) -> ("error out"=w1888:errorcluster, "File path"=w1884:path)  [unwired: 7 in]
        n1511 = case shown="True" "RemoveReq?" {
          tunnel: w1888 -> [w1920 w1924]
          tunnel: [w1920 w1923] -> w1825
          tunnel: w1877 -> [_ w1921]
          frame False {
          }
          frame True {
            w1922 = u16 3 items=["Send", "Read", "Download", "Remove"] ("Send/Read/Download/Remove")
            n1512 = call "HTTPGetRequest_Inst.vi"("Send/Read/Download/Remove"=w1922, "error in (no error)"=w1924, "ReqNum"=w1921) -> ("error out"=w1923:errorcluster)  [unwired: 6 in, 2 out]
          }
        }
        n1513 = property on="Freq-Period" class="Str"(error in=w1825, "Visible"=w1852) -> (error out=w1850:errorcluster)  [unwired: 1 in, 1 out]
        n1514 = property on="Ampl-HighL" class="Str"(error in=w1850, "Visible"=w1852) -> (error out=w1849:errorcluster)  [unwired: 1 in, 1 out]
        n1515 = property on="Offset-LowL" class="Str"(error in=w1849, "Visible"=w1852) -> (error out=w1848:errorcluster)  [unwired: 1 in, 1 out]
        n1516 = property on="PhaseStr" class="Str"(error in=w1848, "Visible"=w1852) -> (error out=w1851:errorcluster)  [unwired: 1 in, 1 out]
        n1517 = property on="Duty-Width" class="Str"(error in=w1851, "Visible"=w1852) -> (error out=w1854:errorcluster)  [unwired: 1 in, 1 out]
        n1518 = property on="SymmStr" class="Str"(error in=w1854, "Visible"=w1852) -> (error out=w1853:errorcluster)  [unwired: 1 in, 1 out]
        n1519 = property on="RisEdgeStr" class="Str"(error in=w1853, "Visible"=w1852) -> (error out=w1847:errorcluster)  [unwired: 1 in, 1 out]
        n1520 = property on="FallEdgeStr" class="Str"(error in=w1847, "Visible"=w1852) -> (error out=w1846:errorcluster)  [unwired: 1 in, 1 out]
        n1521 = property on="Freq/Period" class="Bool (strict)"(error in=w1846, "Visible"=w1855) -> (error out=w1858:errorcluster)  [unwired: 1 in, 1 out]
        n1522 = property on="Ampl/HighL" class="Bool (strict)"(error in=w1858, "Visible"=w1855) -> (error out=w1857:errorcluster)  [unwired: 1 in, 1 out]
        n1523 = property on="Offset/LowL" class="Bool (strict)"(error in=w1857, "Visible"=w1855) -> (error out=w1856:errorcluster)  [unwired: 1 in, 1 out]
        n1524 = property on="Duty/Width" class="Bool (strict)"(error in=w1856, "Visible"=w1855) -> (error out=w1833:errorcluster)  [unwired: 1 in, 1 out]
        n1525 = call "RDG822 Update Screen.vi"("error in"=w1825, "Path to file"=w1884) -> ("error out"=w1894:errorcluster, "Screen"=w1885:picture)  [unwired: 8 in]
        n1526 = property on="Freq" class="DigNum (strict)"(error in=w1833, "Visible"=w1845) -> (error out=w1841:errorcluster)  [unwired: 1 in, 1 out]
        n1527 = property on="Period" class="DigNum (strict)"(error in=w1841, "Visible"=w1845) -> (error out=w1840:errorcluster)  [unwired: 1 in, 1 out]
        n1528 = property on="Ampl" class="DigNum (strict)"(error in=w1840, "Visible"=w1845) -> (error out=w1839:errorcluster)  [unwired: 1 in, 1 out]
        n1529 = property on="HighL" class="DigNum (strict)"(error in=w1839, "Visible"=w1845) -> (error out=w1842:errorcluster)  [unwired: 1 in, 1 out]
        n1530 = property on="Offset" class="DigNum (strict)"(error in=w1842, "Visible"=w1845) -> (error out=w1838:errorcluster)  [unwired: 1 in, 1 out]
        n1531 = property on="LowL" class="DigNum (strict)"(error in=w1838, "Visible"=w1845) -> (error out=w1837:errorcluster)  [unwired: 1 in, 1 out]
        n1532 = property on="PhaseDBL" class="DigNum (strict)"(error in=w1837, "Visible"=w1845) -> (error out=w1843:errorcluster)  [unwired: 1 in, 1 out]
        n1533 = property on="Duty" class="DigNum (strict)"(error in=w1843, "Visible"=w1845) -> (error out=w1844:errorcluster)  [unwired: 1 in, 1 out]
        n1534 = property on="SymmDBL" class="DigNum (strict)"(error in=w1844, "Visible"=w1845) -> (error out=w1836:errorcluster)  [unwired: 1 in, 1 out]
        n1535 = property on="Width" class="DigNum (strict)"(error in=w1836, "Visible"=w1845) -> (error out=w1835:errorcluster)  [unwired: 1 in, 1 out]
        n1536 = property on="RisEdgeDBL" class="DigNum (strict)"(error in=w1835, "Visible"=w1845) -> (error out=w1834:errorcluster)  [unwired: 1 in, 1 out]
        n1537 = property on="FallEdgeDBL" class="DigNum (strict)"(error in=w1834, "Visible"=w1845) -> (error out=w1826:errorcluster)  [unwired: 1 in, 1 out]
        n1538 = local write "error out"(w1894) -> ()
        n1539 = local write "Screen"(w1885) -> ()
        n1540 = call "Time Delay5"() -> ("error out"=w1896:errorcluster)  [unwired: 11 in]
        n1541 = property on="Sine" class="Bool (strict)"(error in=w1826, "Visible"=w1832) -> (error out=w1829:errorcluster)  [unwired: 1 in, 1 out]
        n1542 = property on="Square" class="Bool (strict)"(error in=w1829, "Visible"=w1832) -> (error out=w1828:errorcluster)  [unwired: 1 in, 1 out]
        n1543 = property on="Ramp" class="Bool (strict)"(error in=w1828, "Visible"=w1832) -> (error out=w1827:errorcluster)  [unwired: 1 in, 1 out]
        n1544 = property on="Pulse" class="Bool (strict)"(error in=w1827, "Visible"=w1832) -> (error out=w1830:errorcluster)  [unwired: 1 in, 1 out]
        n1545 = property on="Noise" class="Bool (strict)"(error in=w1830, "Visible"=w1832) -> (error out=w1831:errorcluster)  [unwired: 1 in, 1 out]
        n1546 = property on="DC" class="Bool (strict)"(error in=w1831, "Visible"=w1832) -> ()  [unwired: 1 in, 2 out]
        n1547 = property on="Out1" class="Bool (strict)"(error in=w1896, "Value"=FALSE ("Out1")) -> ()  [unwired: 1 in, 2 out]
      }
      event "Out2": Value Change {
        (unwired) 2 items=["Channel 1"=1, "Channel 2"=2] ("Output Channel (1: Channel 1)")
        # "Same as Out1 eventually"
        n1548 = event-data() -> ()  [unwired: 1 in, 6 out]
      }
    }
  }
